vi "JSONtext Path Library Comparison.vi"() -> ()   [LabVIEW 2017]
uses:
  7f925563-714d-4489-9e01-5d8a939aa36c.vi
  <vilib>/addons/JSON API/JSON Value/Set from JSON string.vi
  Find Multiple Items.vi
  7f925563-714d-4489-9e01-5d8a939aa36c.vi/b1efde3c-89ab-4274-81c5-8c2e9ff736ec.vi
  String Subset.vi
  support/Strip Quotes and Unescape.vi
  Parse Full Path or Item Name.vi
  Find Item Locations by Path.vi
  support/Unescape JSON string.vi
  JSON text to Variant.vi
  <vilib>/addons/JSON API/Variant JSON/Get as Variant.vi
  <vilib>/addons/JSON API/JSON Value/JSON Value.lvclass
  <vilib>/addons/JSON API/Get Polymorphic/JSON GetSet.lvlib
  <vilib>/addons/JSON API/Variant JSON/Variant JSON.lvlib
  <vilib>/addons/_JKI.lib/Serialization/JSON/JKI JSON Serialization.lvlib
panel:
  in  "Library to use":T1(ring) caption="Enum 3"
  out "Array of Data":T2(array[cluster])
  out "JSON size (bytes)":i32 format="%.0p"
  out "Elements Returned":i32 format="%#.3p"
  out "Execution Time":dbl format="%#_3p"
  out "error out":errorcluster
  in  "Example JSON":string="[\n  {\n    \"_id\": \"59b53bcb02b0cb1b19bb98a8\",\n    \"index\": 0,\n    \"guid\": \"787c1912-662d-48b9-b395-2ad75d217224\",\n    \"isActive\": true,\n    \"balance\": \"$3,889.42\",\n    \"picture\": \"http://placehold.it/32x32\",\n    \"age\": 28,\n    \"eyeColor\": \"green\",\n    \"name\": \"Brady York\",\n    \"gender\": \"male\",\n    \"company\": \"ELEMANTRA\",\n    \"email\": \"bradyyork@elemantra.com\",\n    \"phone\": \"+1 (932) 487-2014\",\n    \"address\": \"349 Amber Street, Day, Rhode Island, 8815\",\n    \"about\": \"Culpa magna magna incididunt aliquip adipisicing incididunt. Culpa ex qui aliqua aliqua sint aliqua incididunt duis. Labore consectetur in pariatur qui anim reprehenderit duis.\\r\\n\",\n    \"registered\": \"2014-10-21T08:11:24 -01:00\",\n    \"latitude\": -14.331614,\n    \"longitude\": -65.032248,\n    \"tags\": [\n      \"sint\",\n      \"sint\",\n      \"magna\",\n      \"laboris\",\n      \"irure\",\n      \"aliquip\",\n      \"voluptate\"\n    ],\n    \"friends\": [\n      {\n        \"id\": 0,\n        \"name\": \"Magdalena Stanley\"\n      },\n      {\n        \"id\": 1,\n        \"name\": \"Gill Alvarez\"\n      },\n      {\n        \"id\": 2,\n        \"name\": \"Alston Pacheco\"\n      }\n    ],\n    \"greeting\": \"Hello, Brady York! You have 8 unread messages.\",\n    \"favoriteFruit\": \"banana\"\n  },\n  {\n    \"_id\": \"59b53bcb7e0f92dbc6bce359\",\n    \"index\": 1,\n    \"guid\": \"d1f7a7d2-daca-4b07-b037-18389dc096b8\",\n    \"isActive\": true,\n    \"balance\": \"$1,568.70\",\n    \"picture\": \"http://placehold.it/32x32\",\n    \"age\": 24,\n    \"eyeColor\": \"brown\",\n    \"name\": \"Eula Price\",\n    \"gender\": \"female\",\n    \"company\": \"LIMAGE\",\n    \"email\": \"eulaprice@limage.com\",\n    \"phone\": \"+1 (901) 569-3603\",\n    \"address\": \"883 Chester Avenue, Zeba, New Jersey, 8959\",\n    \"about\": \"Eiusmod aute do deserunt do sunt occaecat. Elit Lorem consequat consequat dolor. Ea ex exercitation nulla voluptate duis commodo fugiat tempor dolor exercitation nulla tempor. Incididunt ipsum sit minim eu excepteur commodo aliquip enim est incididunt dolore aute.\\r\\n\",\n    \"registered\": \"2017-06-22T12:52:36 -01:00\",\n    \"latitude\": -9.342636,\n    \"longitude\": -164.688312,\n    \"tags\": [\n      \"aliqua\",\n      \"anim\",\n      \"laboris\",\n      \"aliqua\",\n      \"dolore\",\n      \"reprehenderit\",\n      \"aute\"\n    ],\n    \"friends\": [\n      {\n        \"id\": 0,\n        \"name\": \"Lelia Gray\"\n      },\n      {\n        \"id\": 1,\n        \"name\": \"Gaines Owen\"\n      },\n      {\n        \"id\": 2,\n        \"name\": \"Lana Schneider\"\n      }\n    ],\n    \"greeting\": \"Hello, Eula Price! You have 6 unread messages.\",\n    \"favoriteFruit\": \"strawberry\"\n  },\n  {\n    \"_id\": \"59b53bcbc4753318b4f57283\",\n    \"index\": 2,\n    \"guid\": \"6fdbd945-01ed-452f-ad4a-aea4d254b9e8\",\n    \"isActive\": false,\n    \"balance\": \"$2,290.73\",\n    \"picture\": \"http://placehold.it/32x32\",\n    \"age\": 27,\n    \"eyeColor\": \"brown\",\n    \"name\": \"Kirk Battle\",\n    \"gender\": \"male\",\n    \"company\": \"TWIIST\",\n    \"email\": \"kirkbattle@twiist.com\",\n    \"phone\": \"+1 (880) 533-3536\",\n    \"address\": \"947 Evergreen Avenue, Eagletown, Kentucky, 5383\",\n    \"about\": \"Nostrud et pariatur labore sint. Est magna cillum enim consectetur veniam reprehenderit fugiat labore consectetur quis. Id ullamco minim amet ut cupidatat exercitation. Ullamco minim et do elit in voluptate voluptate duis. Voluptate duis ad sunt adipisicing minim officia velit dolore ea culpa eiusmod.\\r\\n\",\n    \"registered\": \"2015-06-20T10:39:15 -01:00\",\n    \"latitude\": 6.407172,\n    \"longitude\": -0.155464,\n    \"tags\": [\n      \"tempor\",\n      \"id\",\n      \"pariatur\",\n      \"dolore\",\n      \"nisi\",\n      \"sint\",\n      \"Lorem\"\n    ],\n    \"friends\": [\n      {\n        \"id\": 0,\n        \"name\": \"Dominguez Rasmussen\"\n      },\n      {\n        \"id\": 1,\n        \"name\": \"Augusta Gardner\"\n      },\n      {\n        \"id\": 2,\n        \"name\": \"Odom Nelson\"\n      }\n    ],\n    \"greeting\": \"Hello, Kirk Battle! You have 8 unread messages.\",\n    \"favoriteFruit\": \"banana\"\n  },\n  {\n    \"_id\": \"59b53bcb6051aabb2b97f0db\",\n    \"index\": 3,\n    \"guid\": \"2eb5b3b2-ee26-4324-ab7e-5653592530f9\",\n    \"isActive\": true,\n    \"balance\": \"$2,336.96\",\n    \"picture\": \"http://placehold.it/32x32\",\n    \"age\": 22,\n    \"eyeColor\": \"blue\",\n    \"name\": \"Bonnie Bell\",\n    \"gender\": \"female\",\n    \"company\": \"VIRVA\",\n    \"email\": \"bonniebell@virva.com\",\n    \"phone\": \"+1 (810) 554-2772\",\n    \"address\": \"559 Dakota Place, Kenmar, Arizona, 4025\",\n    \"about\": \"Anim in aliquip sunt fugiat laborum ea elit minim. Cillum nostrud ullamco ut minim nisi qui quis consequat deserunt in. Nostrud exercitation excepteur quis pariatur deserunt ea proident Lorem nostrud occaecat eu incididunt aute.\\r\\n\",\n    \"registered\": \"2016-10-31T11:45:40 -00:00\",\n    \"latitude\": -65.962147,\n    \"longitude\": 21.528794,\n    \"tags\": [\n      \"et\",\n      \"ex\",\n      \"in\",\n      \"ipsum\",\n      \"consectetur\",\n      \"eu\",\n      \"laborum\"\n    ],\n    \"friends\": [\n      {\n        \"id\": 0,\n        \"name\": \"Kirsten Keller\"\n      },\n      {\n        \"id\": 1,\n        \"name\": \"Martina Ferrell\"\n      },\n      {\n        \"id\": 2,\n        \"name\": \"Lambert Sutton\"\n      }\n    ],\n    \"greeting\": \"Hello, Bonnie Bell! You have 3 unread messages.\",\n    \"favoriteFruit\": \"banana\"\n  },\n  {\n    \"_id\": \"59b53bcb7231edd238041f2d\",\n    \"index\": 4,\n    \"guid\": \"f09317d0-8eee-46ff-9b91-58a5b0d46ece\",\n    \"isActive\": true,\n    \"balance\": \"$3,106.19\",\n    \"picture\": \"http://placehold.it/32x32\",\n    \"age\": 30,\n    \"eyeColor\": \"blue\",\n    \"name\": \"Krista Nichols\",\n    \"gender\": \"female\",\n    \"company\": \"ZORROMOP\",\n    \"email\": \"kristanichols@zorromop.com\",\n    \"phone\": \"+1 (807) 565-2677\",\n    \"address\": \"894 Norfolk Street, Clarktown, American Samoa, 9119\",\n    \"about\": \"Do est commodo esse in amet commodo non occaecat. Duis dolore ipsum fugiat amet aliqua ipsum est sunt est minim aliqua. Elit sit sit labore cupidatat do amet nulla.\\r\\n\",\n    \"registered\": \"2015-10-09T10:59:26 -01:00\",\n    \"latitude\": 54.865149,\n    \"longitude\": -44.341326,\n    \"tags\": [\n      \"sint\",\n      \"deserunt\",\n      \"elit\",\n      \"dolore\",\n      \"incididunt\",\n      \"sit\",\n      \"nostrud\"\n    ],\n    \"friends\": [\n      {\n        \"id\": 0,\n        \"name\": \"Sadie Carroll\"\n      },\n      {\n        \"id\": 1,\n        \"name\": \"Alice Oliver\"\n      },\n      {\n        \"id\": 2,\n        \"name\": \"Haynes Morris\"\n      }\n    ],\n    \"greeting\": \"Hello, Krista Nichols! You have 9 unread messages.\",\n    \"favoriteFruit\": \"banana\"\n  },\n  {\n    \"_id\": \"59b53bcbe9ba31e9db12c1da\",\n    \"index\": 5,\n    \"guid\": \"a3768281-1188-4880-8873-7d13400a9810\",\n    \"isActive\": true,\n    \"balance\": \"$2,102.60\",\n    \"picture\": \"http://placehold.it/32x32\",\n    \"age\": 37,\n    \"eyeColor\": \"blue\",\n    \"name\": \"Carver Gay\",\n    \"gender\": \"male\",\n    \"company\": \"COMTOURS\",\n    \"email\": \"carvergay@comtours.com\",\n    \"phone\": \"+1 (820) 410-2285\",\n    \"address\": \"253 Dare Court, Henrietta, Massachusetts, 2610\",\n    \"about\": \"Eiusmod magna Lorem anim incididunt do. Labore sunt id tempor veniam aliquip veniam non non reprehenderit reprehenderit consectetur amet. Do ad fugiat esse do ut proident dolore ad irure fugiat id fugiat aliqua consequat. Est quis consequat incididunt duis amet.\\r\\n\",\n    \"registered\": \"2016-03-09T10:06:33 -00:00\",\n    \"latitude\": -71.722611,\n    \"longitude\": 93.206354,\n    \"tags\": [\n      \"Lorem\",\n      \"laborum\",\n      \"cillum\",\n      \"culpa\",\n      \"quis\",\n      \"anim\",\n      \"Lorem\"\n    ],\n    \"friends\": [\n      {\n        \"id\": 0,\n        \"name\": \"Gibbs Silva\"\n      },\n      {\n        \"id\": 1,\n        \"name\": \"Vincent Herring\"\n      },\n      {\n        \"id\": 2,\n        \"name\": \"Bauer Edwards\"\n      }\n    ],\n    \"greeting\": \"Hello, Carver Gay! You have 2 unread messages.\",\n    \"favoriteFruit\": \"strawberry\"\n  },\n  {\n    \"_id\": \"59b53bcb7bbaae10a2aefeae\",\n    \"index\": 6,\n    \"guid\": \"bb9b5fd7-c1e4-4f49-b969-c4ee1fd49b81\",\n    \"isActive\": true,\n    \"balance\": \"$1,213.38\",\n    \"picture\": \"http://placehold.it/32x32\",\n    \"age\": 36,\n    \"eyeColor\": \"blue\",\n    \"name\": \"Jacobson Carlson\",\n    \"gender\": \"male\",\n    \"company\": \"GRONK\",\n    \"email\": \"jacobsoncarlson@gronk.com\",\n    \"phone\": \"+1 (892) 428-3382\",\n    \"address\": \"267 Empire Boulevard, Sena, Maine, 8522\",\n    \"about\": \"Eu nulla tempor reprehenderit laboris nostrud eiusmod. Elit aliquip veniam sit qui nisi ipsum enim cupidatat est qui adipisicing aute. Pariatur non et aliquip est. Consectetur cupidatat cupidatat consectetur nostrud dolor nostrud. Excepteur aliquip ut ipsum mollit culpa magna consequat adipisicing labore id est tempor amet. Incididunt ad tempor sit eiusmod officia duis amet.\\r\\n\",\n    \"registered\": \"2014-11-08T12:40:45 -00:00\",\n    \"latitude\": 74.024148,\n    \"longitude\": -149.038221,\n    \"tags\": [\n      \"deserunt\",\n      \"aliqua\",\n      \"do\",\n      \"excepteur\",\n      \"do\",\n      \"consequat\",\n      \"eiusmod\"\n    ],\n    \"friends\": [\n      {\n        \"id\": 0,\n        \"name\": \"Schmidt Boone\"\n      },\n      {\n        \"id\": 1,\n        \"name\": \"Chandler Guthrie\"\n      },\n      {\n        \"id\": 2,\n        \"name\": \"Mavis Beard\"\n      }\n    ],\n    \"greeting\": \"Hello, Jacobson Carlson! You have 4 unread messages.\",\n    \"favoriteFruit\": \"strawberry\"\n  },\n  {\n    \"_id\": \"59b53bcb03716bd89bef4059\",\n    \"index\": 7,\n    \"guid\": \"78ea5110-fabf-45ce-980c-5751b3eb6da0\",\n    \"isActive\": true,\n    \"balance\": \"$3,940.00\",\n    \"picture\": \"http://placehold.it/32x32\",\n    \"age\": 39,\n    \"eyeColor\": \"blue\",\n    \"name\": \"Holt Kirk\",\n    \"gender\": \"male\",\n    \"company\": \"GLEAMINK\",\n    \"email\": \"holtkirk@gleamink.com\",\n    \"phone\": \"+1 (978) 536-2129\",\n    \"address\": \"977 Maujer Street, Oberlin, Guam, 2555\",\n    \"about\": \"Ullamco dolore dolore cupidatat et occaecat nisi sunt et ea tempor qui est in. Elit amet ex ad ullamco tempor ea. Ipsum occaecat id culpa enim laborum id laborum aute dolor ullamco. Dolore est ut exercitation fugiat ad mollit consectetur. Labore esse non magna duis do. Est qui enim nisi exercitation ullamco ea cillum do ullamco.\\r\\n\",\n    \"registered\": \"2014-01-26T04:53:21 -00:00\",\n    \"latitude\": 80.154467,\n    \"longitude\": -139.457001,\n    \"tags\": [\n      \"in\",\n      \"proident\",\n      \"eu\",\n      \"esse\",\n      \"aute\",\n      \"ea\",\n      \"laborum\"\n    ],\n    \"friends\": [\n      {\n        \"id\": 0,\n        \"name\": \"Ayers Collins\"\n      },\n      {\n        \"id\": 1,\n        \"name\": \"Morgan Lynch\"\n      },\n      {\n        \"id\": 2,\n        \"name\": \"Millicent Rodriquez\"\n      }\n    ],\n    \"greeting\": \"Hello, Holt Kirk! You have 7 unread messages.\",\n    \"favoriteFruit\": \"strawberry\"\n  },\n  {\n    \"_id\": \"59b53bcbe46b05505f1d73c6\",\n    \"index\": 8,\n    \"guid\": \"5c0b76e2-83b6-48c8-a04b-d989644174a0\",\n    \"isActive\": false,\n    \"balance\": \"$2,251.01\",\n    \"picture\": \"http://placehold.it/32x32\",\n    \"age\": 34,\n    \"eyeColor\": \"blue\",\n    \"name\": \"Patrica Gates\",\n    \"gender\": \"female\",\n    \"company\": \"PAPRIKUT\",\n    \"email\": \"patricagates@paprikut.com\",\n    \"phone\": \"+1 (989) 486-2454\",\n    \"address\": \"284 Kane Street, Sheatown, Texas, 2404\",\n    \"about\": \"Veniam nostrud non veniam eiusmod mollit fugiat duis. Et Lorem elit ea eiusmod elit aute aute officia sit cillum. Consectetur cillum est duis sunt amet ex velit enim. Do consectetur sint deserunt deserunt minim esse dolore sit nisi ullamco cillum.\\r\\n\",\n    \"registered\": \"2014-10-22T11:45:11 -01:00\",\n    \"latitude\": -25.077939,\n    \"longitude\": -10.063782,\n    \"tags\": [\n      \"id\",\n      \"adipisicing\",\n      \"amet\",\n      \"nostrud\",\n      \"aliquip\",\n      \"ut\",\n      \"dolor\"\n    ],\n    \"friends\": [\n      {\n        \"id\": 0,\n        \"name\": \"Pollard Sawyer\"\n      },\n      {\n        \"id\": 1,\n        \"name\": \"Ortiz Perry\"\n      },\n      {\n        \"id\": 2,\n        \"name\": \"Britney Mullins\"\n      }\n    ],\n    \"greeting\": \"Hello, Patrica Gates! You have 5 unread messages.\",\n    \"favoriteFruit\": \"apple\"\n  },\n  {\n    \"_id\": \"59b53bcbcc629b542a162d0b\",\n    \"index\": 9,\n    \"guid\": \"4bc20eef-7f7d-48d6-8d1a-8c46d3ecaa0a\",\n    \"isActive\": true,\n    \"balance\": \"$1,093.57\",\n    \"picture\": \"http://placehold.it/32x32\",\n    \"age\": 24,\n    \"eyeColor\": \"green\",\n    \"name\": \"Latasha Holland\",\n    \"gender\": \"female\",\n    \"company\": \"CYTREX\",\n    \"email\": \"latashaholland@cytrex.com\",\n    \"phone\": \"+1 (898) 545-2211\",\n    \"address\": \"353 Elm Avenue, Steinhatchee, Colorado, 8565\",\n    \"about\": \"Laborum consectetur cupidatat fugiat laborum nulla enim exercitation. Esse amet quis eiusmod veniam est qui excepteur labore nisi ut aliqua incididunt occaecat ea. Tempor veniam laborum laboris in adipisicing veniam ex dolor nulla eiusmod voluptate qui ex irure.\\r\\n\",\n    \"registered\": \"2015-03-18T11:53:50 -00:00\",\n    \"latitude\": 18.52921,\n    \"longitude\": 82.506415,\n    \"tags\": [\n      \"ad\",\n      \"voluptate\",\n      \"aliquip\",\n      \"velit\",\n      \"non\",\n      \"qui\",\n      \"eiusmod\"\n    ],\n    \"friends\": [\n      {\n        \"id\": 0,\n        \"name\": \"Virginia Kramer\"\n      },\n      {\n        \"id\": 1,\n        \"name\": \"Alba Valencia\"\n      },\n      {\n        \"id\": 2,\n        \"name\": \"Alexandria Webster\"\n      }\n    ],\n    \"greeting\": \"Hello, Latasha Holland! You have 8 unread messages.\",\n    \"favoriteFruit\": \"strawberry\"\n  },\n  {\n    \"_id\": \"59b53bcb597148582fb2963b\",\n    \"index\": 10,\n    \"guid\": \"11d9df14-d3e9-4f7b-bb2c-951e6152d5dd\",\n    \"isActive\": false,\n    \"balance\": \"$1,684.85\",\n    \"picture\": \"http://placehold.it/32x32\",\n    \"age\": 39,\n    \"eyeColor\": \"green\",\n    \"name\": \"Dena Webb\",\n    \"gender\": \"female\",\n    \"company\": \"OPTIQUE\",\n    \"email\": \"denawebb@optique.com\",\n    \"phone\": \"+1 (814) 500-3050\",\n    \"address\": \"542 Bouck Court, Dixonville, Utah, 4706\",\n    \"about\": \"Ad esse duis id excepteur cillum est proident do ullamco. Nulla sunt non fugiat nulla velit ex qui pariatur reprehenderit proident ullamco est. Nulla culpa ullamco minim dolor elit cupidatat veniam sit incididunt mollit elit consequat sit velit. Est quis occaecat ut do id aute. Minim laboris minim ut duis labore do laboris officia. In occaecat et officia reprehenderit amet laborum dolor ullamco. Labore dolor ipsum anim qui cupidatat non magna sunt id mollit aliquip commodo id.\\r\\n\",\n    \"registered\": \"2014-06-03T06:37:29 -01:00\",\n    \"latitude\": 51.581221,\n    \"longitude\": 165.78903,\n    \"tags\": [\n      \"occaecat\",\n      \"magna\",\n      \"consequat\",\n      \"do\",\n      \"ullamco\",\n      \"eiusmod\",\n      \"consectetur\"\n    ],\n    \"friends\": [\n      {\n        \"id\": 0,\n        \"name\": \"Sharron Cleveland\"\n      },\n      {\n        \"id\": 1,\n        \"name\": \"Rosanna Chase\"\n      },\n      {\n        \"id\": 2,\n        \"name\": \"Amanda Lara\"\n      }\n    ],\n    \"greeting\": \"Hello, Dena Webb! You have 2 unread messages.\",\n    \"favoriteFruit\": \"banana\"\n  },\n  {\n    \"_id\": \"59b53bcbd26ca7bf6f477c07\",\n    \"index\": 11,\n    \"guid\": \"b2758586-d7dc-4aee-bf7e-ec0e02885def\",\n    \"isActive\": true,\n    \"balance\": \"$3,763.33\",\n    \"picture\": \"http://placehold.it/32x32\",\n    \"age\": 32,\n    \"eyeColor\": \"blue\",\n    \"name\": \"Howe Conner\",\n    \"gender\": \"male\",\n    \"company\": \"ATOMICA\",\n    \"email\": \"howeconner@atomica.com\",\n    \"phone\": \"+1 (945) 508-3886\",\n    \"address\": \"335 Cumberland Street, Glenville, Montana, 8652\",\n    \"about\": \"Aute culpa ipsum id anim veniam. Duis laboris ad ullamco proident veniam minim. Cillum velit aliqua amet est. Eu fugiat occaecat sunt pariatur ex.\\r\\n\",\n    \"registered\": \"2015-03-15T08:28:33 -00:00\",\n    \"latitude\": -28.365675,\n    \"longitude\": -65.023882,\n    \"tags\": [\n      \"adipisicing\",\n      \"proident\",\n      \"qui\",\n      \"aute\",\n      \"excepteur\",\n      \"Lorem\",\n      \"nostrud\"\n    ],\n    \"friends\": [\n      {\n        \"id\": 0,\n        \"name\": \"Lucinda Mcclain\"\n      },\n      {\n        \"id\": 1,\n        \"name\": \"Butler Guerrero\"\n      },\n      {\n        \"id\": 2,\n        \"name\": \"Lakeisha Spears\"\n      }\n    ],\n    \"greeting\": \"Hello, Howe Conner! You have 2 unread messages.\",\n    \"favoriteFruit\": \"banana\"\n  },\n  {\n    \"_id\": \"59b53bcbb5418a3e477d54c9\",\n    \"index\": 12,\n    \"guid\": \"e66672d5-084b-400c-9106-13a25f1ffc78\",\n    \"isActive\": true,\n    \"balance\": \"$1,591.82\",\n    \"picture\": \"http://placehold.it/32x32\",\n    \"age\": 27,\n    \"eyeColor\": \"brown\",\n    \"name\": \"Anne Nielsen\",\n    \"gender\": \"female\",\n    \"company\": \"VIOCULAR\",\n    \"email\": \"annenielsen@viocular.com\",\n    \"phone\": \"+1 (970) 495-2904\",\n    \"address\": \"855 Caton Place, Como, Maryland, 9034\",\n    \"about\": \"Tempor anim quis ut aliqua nulla officia occaecat do sit anim ad. Occaecat dolor dolor ad incididunt quis veniam. Labore velit do elit duis laborum consequat Lorem aliquip. Est aliqua occaecat reprehenderit eu laborum ea et sint ea anim consectetur. Anim dolore officia nostrud aute ad adipisicing laboris et occaecat mollit. Tempor dolor ex eu proident elit in.\\r\\n\",\n    \"registered\": \"2017-05-08T12:38:29 -01:00\",\n    \"latitude\": -47.604574,\n    \"longitude\": 7.244034,\n    \"tags\": [\n      \"amet\",\n      \"consequat\",\n      \"magna\",\n      \"excepteur\",\n      \"laboris\",\n      \"tempor\",\n      \"minim\"\n    ],\n    \"friends\": [\n      {\n        \"id\": 0,\n        \"name\": \"Nita Ellison\"\n      },\n      {\n        \"id\": 1,\n        \"name\": \"Kelley England\"\n      },\n      {\n        \"id\": 2,\n        \"name\": \"Blanca Duke\"\n      }\n    ],\n    \"greeting\": \"Hello, Anne Nielsen! You have 5 unread messages.\",\n    \"favoriteFruit\": \"strawberry\"\n  },\n  {\n    \"_id\": \"59b53bcb4ce81ca8bb52f70c\",\n    \"index\": 13,\n    \"guid\": \"2ab4ca63-31a2-4867-9969-bff002881044\",\n    \"isActive\": true,\n    \"balance\": \"$2,822.43\",\n    \"picture\": \"http://placehold.it/32x32\",\n    \"age\": 32,\n    \"eyeColor\": \"green\",\n    \"name\": \"Carroll Kline\",\n    \"gender\": \"male\",\n    \"company\": \"FORTEAN\",\n    \"email\": \"carrollkline@fortean.com\",\n    \"phone\": \"+1 (980) 498-3294\",\n    \"address\": \"111 Goodwin Place, Jardine, Connecticut, 370\",\n    \"about\": \"Lorem aute laborum id labore non nisi veniam ad fugiat labore. Minim fugiat reprehenderit exercitation aliqua ipsum velit Lorem labore ad aliquip nisi cillum eiusmod. Quis aliquip reprehenderit commodo pariatur aliquip eu aute quis dolore occaecat. Nisi id esse ea pariatur voluptate et elit ut ut mollit ea.\\r\\n\",\n    \"registered\": \"2014-12-13T11:18:37 -00:00\",\n    \"latitude\": 44.611706,\n    \"longitude\": -75.982853,\n    \"tags\": [\n      \"non\",\n      \"mollit\",\n      \"pariatur\",\n      \"ad\",\n      \"aliqua\",\n      \"do\",\n      \"laboris\"\n    ],\n    \"friends\": [\n      {\n        \"id\": 0,\n        \"name\": \"Cannon Navarro\"\n      },\n      {\n        \"id\": 1,\n        \"name\": \"Terri Byers\"\n      },\n      {\n        \"id\": 2,\n        \"name\": \"Janell Robinson\"\n      }\n    ],\n    \"greeting\": \"Hello, Carroll Kline! You have 4 unread messages.\",\n    \"favoriteFruit\": \"banana\"\n  },\n  {\n    \"_id\": \"59b53bcb034cefc38e5f718d\",\n    \"index\": 14,\n    \"guid\": \"1b75941b-966f-4520-bda0-746f5f72a03e\",\n    \"isActive\": false,\n    \"balance\": \"$2,799.30\",\n    \"picture\": \"http://placehold.it/32x32\",\n    \"age\": 32,\n    \"eyeColor\": \"brown\",\n    \"name\": \"Forbes Tran\",\n    \"gender\": \"male\",\n    \"company\": \"LYRIA\",\n    \"email\": \"forbestran@lyria.com\",\n    \"phone\": \"+1 (932) 582-3482\",\n    \"address\": \"689 Cook Street, Cleary, Iowa, 2553\",\n    \"about\": \"Occaecat tempor sint nisi amet ex veniam culpa adipisicing ad. Incididunt duis elit amet deserunt eiusmod officia occaecat eiusmod qui incididunt. Eiusmod laboris esse sit incididunt enim eu excepteur est mollit anim ad quis. Mollit nulla culpa veniam incididunt ipsum sit officia sunt aliqua reprehenderit dolor dolore. Culpa excepteur consequat magna elit id ullamco deserunt est in et irure.\\r\\n\",\n    \"registered\": \"2015-05-22T09:52:23 -01:00\",\n    \"latitude\": 9.60954,\n    \"longitude\": -42.310375,\n    \"tags\": [\n      \"mollit\",\n      \"proident\",\n      \"veniam\",\n      \"irure\",\n      \"esse\",\n      \"Lorem\",\n      \"dolore\"\n    ],\n    \"friends\": [\n      {\n        \"id\": 0,\n        \"name\": \"Leila Sims\"\n      },\n      {\n        \"id\": 1,\n        \"name\": \"Desiree Savage\"\n      },\n      {\n        \"id\": 2,\n        \"name\": \"Johnston Hensley\"\n      }\n    ],\n    \"greeting\": \"Hello, Forbes Tran! You have 3 unread messages.\",\n    \"favoriteFruit\": \"banana\"\n  },\n  {\n    \"_id\": \"59b53bcb9a6e9676f507278e\",\n    \"index\": 15,\n    \"guid\": \"3bed5db5-ef23-4804-a3e0-08b3c940d53f\",\n    \"isActive\": true,\n    \"balance\": \"$1,219.22\",\n    \"picture\": \"http://placehold.it/32x32\",\n    \"age\": 39,\n    \"eyeColor\": \"brown\",\n    \"name\": \"Carlson Klein\",\n    \"gender\": \"male\",\n    \"company\": \"AQUACINE\",\n    \"email\": \"carlsonklein@aquacine.com\",\n    \"phone\": \"+1 (978) 572-2330\",\n    \"address\": \"863 Woods Place, Movico, Wyoming, 810\",\n    \"about\": \"Do excepteur nostrud est nisi minim incididunt cillum. Et veniam do in proident deserunt minim sit. Sunt pariatur ipsum tempor elit duis sint sit non non qui laborum duis esse. Sint eiusmod irure pariatur occaecat reprehenderit anim.\\r\\n\",\n    \"registered\": \"2014-05-03T11:19:28 -01:00\",\n    \"latitude\": -56.803333,\n    \"longitude\": -128.863204,\n    \"tags\": [\n      \"tempor\",\n      \"velit\",\n      \"voluptate\",\n      \"et\",\n      \"laboris\",\n      \"consequat\",\n      \"cillum\"\n    ],\n    \"friends\": [\n      {\n        \"id\": 0,\n        \"name\": \"Liliana Sellers\"\n      },\n      {\n        \"id\": 1,\n        \"name\": \"Garcia Larsen\"\n      },\n      {\n        \"id\": 2,\n        \"name\": \"Long Fitzpatrick\"\n      }\n    ],\n    \"greeting\": \"Hello, Carlson Klein! You have 4 unread messages.\",\n    \"favoriteFruit\": \"strawberry\"\n  },\n  {\n    \"_id\": \"59b53bcbac141192de4ff36f\",\n    \"index\": 16,\n    \"guid\": \"5c96733c-76df-40fa-b2b3-d65d58dc0720\",\n    \"isActive\": true,\n    \"balance\": \"$2,144.12\",\n    \"picture\": \"http://placehold.it/32x32\",\n    \"age\": 38,\n    \"eyeColor\": \"blue\",\n    \"name\": \"Maryann Adams\",\n    \"gender\": \"female\",\n    \"company\": \"GEEKY\",\n    \"email\": \"maryannadams@geeky.com\",\n    \"phone\": \"+1 (814) 507-3036\",\n    \"address\": \"701 Albemarle Terrace, Datil, Marshall Islands, 1322\",\n    \"about\": \"Ipsum velit nostrud minim aute velit ut esse occaecat ad voluptate qui ad. Mollit pariatur ullamco Lorem quis elit incididunt anim ullamco officia laborum. Ad incididunt ut ipsum elit elit culpa magna. Nulla quis ex est elit commodo deserunt culpa culpa sint occaecat do. Consectetur irure officia culpa id ex. Et est id minim proident Lorem ea esse aute et qui. Quis enim duis minim sint elit nostrud.\\r\\n\",\n    \"registered\": \"2016-11-20T04:37:14 -00:00\",\n    \"latitude\": -61.054651,\n    \"longitude\": -110.864468,\n    \"tags\": [\n      \"excepteur\",\n      \"minim\",\n      \"amet\",\n      \"magna\",\n      \"fugiat\",\n      \"excepteur\",\n      \"consectetur\"\n    ],\n    \"friends\": [\n      {\n        \"id\": 0,\n        \"name\": \"Megan Petersen\"\n      },\n      {\n        \"id\": 1,\n        \"name\": \"Arline Solis\"\n      },\n      {\n        \"id\": 2,\n        \"name\": \"Carpenter Bishop\"\n      }\n    ],\n    \"greeting\": \"Hello, Maryann Adams! You have 4 unread messages.\",\n    \"favoriteFruit\": \"apple\"\n  },\n  {\n    \"_id\": \"59b53bcbd4794b54dacb02ff\",\n    \"index\": 17,\n    \"guid\": \"9b12691d-534a-49ef-9453-e6db5e086fa3\",\n    \"isActive\": true,\n    \"balance\": \"$1,444.83\",\n    \"picture\": \"http://placehold.it/32x32\",\n    \"age\": 23,\n    \"eyeColor\": \"brown\",\n    \"name\": \"Zelma Hooper\",\n    \"gender\": \"female\",\n    \"company\": \"ENDICIL\",\n    \"email\": \"zelmahooper@endicil.com\",\n    \"phone\": \"+1 (953) 529-2225\",\n    \"address\": \"327 Cherry Street, Sylvanite, Nevada, 1609\",\n    \"about\": \"Aliquip consectetur dolor magna irure voluptate ea. Labore id aute incididunt eiusmod ad cillum est exercitation excepteur officia cupidatat aute. Sit et magna duis duis excepteur ad est sit sint adipisicing commodo. Sint est quis amet ullamco cupidatat nisi enim sint do et.\\r\\n\",\n    \"registered\": \"2015-10-10T05:49:22 -01:00\",\n    \"latitude\": -69.361083,\n    \"longitude\": -9.671064,\n    \"tags\": [\n      \"veniam\",\n      \"officia\",\n      \"dolore\",\n      \"dolore\",\n      \"occaecat\",\n      \"excepteur\",\n      \"dolore\"\n    ],\n    \"friends\": [\n      {\n        \"id\": 0,\n        \"name\": \"Hughes Mcgowan\"\n      },\n      {\n        \"id\": 1,\n        \"name\": \"Corrine Velazquez\"\n      },\n      {\n        \"id\": 2,\n        \"name\": \"Wade Kirkland\"\n      }\n    ],\n    \"greeting\": \"Hello, Zelma Hooper! You have 6 unread messages.\",\n    \"favoriteFruit\": \"strawberry\"\n  },\n  {\n    \"_id\": \"59b53bcb68e219d872f06a49\",\n    \"index\": 18,\n    \"guid\": \"861c801f-0f15-4390-8104-311e6d6f83d8\",\n    \"isActive\": true,\n    \"balance\": \"$2,222.35\",\n    \"picture\": \"http://placehold.it/32x32\",\n    \"age\": 34,\n    \"eyeColor\": \"green\",\n    \"name\": \"Gwen Cook\",\n    \"gender\": \"female\",\n    \"company\": \"BESTO\",\n    \"email\": \"gwencook@besto.com\",\n    \"phone\": \"+1 (999) 515-3826\",\n    \"address\": \"151 Wythe Place, Hessville, North Carolina, 3410\",\n    \"about\": \"Fugiat aliqua nulla ea et do tempor ex sit mollit. Aliquip id dolor incididunt eu anim. Qui ex Lorem ut tempor veniam sit nostrud. Sint elit adipisicing laboris exercitation enim sint. Ipsum in anim quis magna. Ullamco deserunt voluptate reprehenderit tempor ea proident ea. Ea ad deserunt esse anim quis.\\r\\n\",\n    \"registered\": \"2016-01-02T10:58:42 -00:00\",\n    \"latitude\": 62.88102,\n    \"longitude\": -110.611076,\n    \"tags\": [\n      \"veniam\",\n      \"consectetur\",\n      \"consequat\",\n      \"fugiat\",\n      \"aliqua\",\n      \"incididunt\",\n      \"deserunt\"\n    ],\n    \"friends\": [\n      {\n        \"id\": 0,\n        \"name\": \"Powell Burris\"\n      },\n      {\n        \"id\": 1,\n        \"name\": \"Nina Burt\"\n      },\n      {\n        \"id\": 2,\n        \"name\": \"Brandi Barber\"\n      }\n    ],\n    \"greeting\": \"Hello, Gwen Cook! You have 4 unread messages.\",\n    \"favoriteFruit\": \"apple\"\n  },\n  {\n    \"_id\": \"59b53bcb7b31d5c7dd72738c\",\n    \"index\": 19,\n    \"guid\": \"a44d6ef3-72ce-47e3-be35-e26aef54e05c\",\n    \"isActive\": true,\n    \"balance\": \"$2,772.61\",\n    \"picture\": \"http://placehold.it/32x32\",\n    \"age\": 27,\n    \"eyeColor\": \"brown\",\n    \"name\": \"Ray Sheppard\",\n    \"gender\": \"male\",\n    \"company\": \"STEELFAB\",\n    \"email\": \"raysheppard@steelfab.com\",\n    \"phone\": \"+1 (833) 576-3166\",\n    \"address\": \"421 Noel Avenue, Fruitdale, New Mexico, 1023\",\n    \"about\": \"Nisi tempor ea nostrud reprehenderit labore Lorem proident adipisicing aliqua anim ad. Lorem id mollit nisi et minim nostrud proident commodo et dolore ex. Lorem anim eu eu sint exercitation sint.\\r\\n\",\n    \"registered\": \"2016-10-14T02:28:34 -01:00\",\n    \"latitude\": -21.473911,\n    \"longitude\": -178.75414,\n    \"tags\": [\n      \"deserunt\",\n      \"sint\",\n      \"culpa\",\n      \"mollit\",\n      \"minim\",\n      \"aute\",\n      \"dolor\"\n    ],\n    \"friends\": [\n      {\n        \"id\": 0,\n        \"name\": \"Joan Donaldson\"\n      },\n      {\n        \"id\": 1,\n        \"name\": \"Lilly Hansen\"\n      },\n      {\n        \"id\": 2,\n        \"name\": \"Francis Foster\"\n      }\n    ],\n    \"greeting\": \"Hello, Ray Sheppard! You have 1 unread messages.\",\n    \"favoriteFruit\": \"banana\"\n  },\n  {\n    \"_id\": \"59b53bcbfc475205683d24fb\",\n    \"index\": 20,\n    \"guid\": \"70656bad-68de-4581-9553-567f23d70256\",\n    \"isActive\": false,\n    \"balance\": \"$1,071.41\",\n    \"picture\": \"http://placehold.it/32x32\",\n    \"age\": 23,\n    \"eyeColor\": \"green\",\n    \"name\": \"Kerr Bowman\",\n    \"gender\": \"male\",\n    \"company\": \"SUPPORTAL\",\n    \"email\": \"kerrbowman@supportal.com\",\n    \"phone\": \"+1 (915) 525-3701\",\n    \"address\": \"387 Gallatin Place, Williston, Michigan, 658\",\n    \"about\": \"Sint nostrud qui deserunt sit tempor esse do sunt amet exercitation anim nulla. Eiusmod ex tempor in officia consequat dolor exercitation irure incididunt nulla nulla do. Mollit magna do et ea cupidatat elit ipsum adipisicing voluptate cupidatat eiusmod non.\\r\\n\",\n    \"registered\": \"2015-07-19T05:10:09 -01:00\",\n    \"latitude\": -61.588655,\n    \"longitude\": -69.987029,\n    \"tags\": [\n      \"laborum\",\n      \"laborum\",\n      \"consequat\",\n      \"ut\",\n      \"magna\",\n      \"voluptate\",\n      \"esse\"\n    ],\n    \"friends\": [\n      {\n        \"id\": 0,\n        \"name\": \"Beryl Wolfe\"\n      },\n      {\n        \"id\": 1,\n        \"name\": \"Viola Hamilton\"\n      },\n      {\n        \"id\": 2,\n        \"name\": \"Jannie Whitehead\"\n      }\n    ],\n    \"greeting\": \"Hello, Kerr Bowman! You have 2 unread messages.\",\n    \"favoriteFruit\": \"banana\"\n  },\n  {\n    \"_id\": \"59b53bcb8d287deabf6d0b79\",\n    \"index\": 21,\n    \"guid\": \"7c1a5e48-bb0e-4c13-81d4-88d15f5cbdd2\",\n    \"isActive\": false,\n    \"balance\": \"$3,025.85\",\n    \"picture\": \"http://placehold.it/32x32\",\n    \"age\": 31,\n    \"eyeColor\": \"green\",\n    \"name\": \"Aline Fleming\",\n    \"gender\": \"female\",\n    \"company\": \"COMCUR\",\n    \"email\": \"alinefleming@comcur.com\",\n    \"phone\": \"+1 (973) 454-2935\",\n    \"address\": \"736 Harbor Court, Allison, Oregon, 7524\",\n    \"about\": \"Do dolore deserunt dolor anim ex cillum ea amet ipsum in irure. Labore nisi culpa deserunt ipsum quis exercitation fugiat esse velit dolor reprehenderit. Ea id non quis ipsum officia. Enim veniam minim excepteur do dolore commodo nulla culpa irure.\\r\\n\",\n    \"registered\": \"2015-03-20T09:17:16 -00:00\",\n    \"latitude\": -85.661732,\n    \"longitude\": -109.540686,\n    \"tags\": [\n      \"laborum\",\n      \"aute\",\n      \"do\",\n      \"magna\",\n      \"do\",\n      \"Lorem\",\n      \"officia\"\n    ],\n    \"friends\": [\n      {\n        \"id\": 0,\n        \"name\": \"Corinne Rush\"\n      },\n      {\n        \"id\": 1,\n        \"name\": \"Pearlie Fuentes\"\n      },\n      {\n        \"id\": 2,\n        \"name\": \"Shelton Mendoza\"\n      }\n    ],\n    \"greeting\": \"Hello, Aline Fleming! You have 9 unread messages.\",\n    \"favoriteFruit\": \"banana\"\n  },\n  {\n    \"_id\": \"59b53bcb21bc1b9e689f86cd\",\n    \"index\": 22,\n    \"guid\": \"89e79c28-d1d3-4cf0-a7db-e52663288896\",\n    \"isActive\": false,\n    \"balance\": \"$1,913.46\",\n    \"picture\": \"http://placehold.it/32x32\",\n    \"age\": 20,\n    \"eyeColor\": \"green\",\n    \"name\": \"Stacey Hickman\",\n    \"gender\": \"female\",\n    \"company\": \"OLYMPIX\",\n    \"email\": \"staceyhickman@olympix.com\",\n    \"phone\": \"+1 (885) 484-3824\",\n    \"address\": \"738 Oxford Walk, Bagtown, Florida, 6859\",\n    \"about\": \"Occaecat in in do commodo esse aute. Consectetur voluptate amet dolore ad amet reprehenderit. Ut ullamco velit labore exercitation commodo adipisicing ea ea. Cupidatat do pariatur excepteur commodo tempor aute sint exercitation.\\r\\n\",\n    \"registered\": \"2017-06-13T05:36:22 -01:00\",\n    \"latitude\": 48.262654,\n    \"longitude\": -98.857032,\n    \"tags\": [\n      \"culpa\",\n      \"excepteur\",\n      \"irure\",\n      \"officia\",\n      \"minim\",\n      \"mollit\",\n      \"officia\"\n    ],\n    \"friends\": [\n      {\n        \"id\": 0,\n        \"name\": \"Natasha Anderson\"\n      },\n      {\n        \"id\": 1,\n        \"name\": \"Blackwell Blanchard\"\n      },\n      {\n        \"id\": 2,\n        \"name\": \"Iva Riggs\"\n      }\n    ],\n    \"greeting\": \"Hello, Stacey Hickman! You have 1 unread messages.\",\n    \"favoriteFruit\": \"banana\"\n  },\n  {\n    \"_id\": \"59b53bcbf9cf2b4cfa69d511\",\n    \"index\": 23,\n    \"guid\": \"54e3fdd1-4f8d-42dc-9828-ba8270d810c4\",\n    \"isActive\": true,\n    \"balance\": \"$1,863.08\",\n    \"picture\": \"http://placehold.it/32x32\",\n    \"age\": 30,\n    \"eyeColor\": \"brown\",\n    \"name\": \"Dora Larson\",\n    \"gender\": \"female\",\n    \"company\": \"XTH\",\n    \"email\": \"doralarson@xth.com\",\n    \"phone\": \"+1 (817) 432-2284\",\n    \"address\": \"433 Love Lane, Cliff, Minnesota, 8201\",\n    \"about\": \"Ad id pariatur nulla Lorem consequat. In veniam dolore do nisi incididunt. Mollit occaecat quis irure ut consectetur in duis culpa adipisicing in sunt consequat adipisicing.\\r\\n\",\n    \"registered\": \"2015-03-08T09:12:31 -00:00\",\n    \"latitude\": 42.824631,\n    \"longitude\": -141.172328,\n    \"tags\": [\n      \"laborum\",\n      \"ut\",\n      \"fugiat\",\n      \"veniam\",\n      \"cupidatat\",\n      \"sit\",\n      \"et\"\n    ],\n    \"friends\": [\n      {\n        \"id\": 0,\n        \"name\": \"Coffey Munoz\"\n      },\n      {\n        \"id\": 1,\n        \"name\": \"Hope Case\"\n      },\n      {\n        \"id\": 2,\n        \"name\": \"Marquez Hutchinson\"\n      }\n    ],\n    \"greeting\": \"Hello, Dora Larson! You have 9 unread messages.\",\n    \"favoriteFruit\": \"banana\"\n  },\n  {\n    \"_id\": \"59b53bcb7452ac2216503911\",\n    \"index\": 24,\n    \"guid\": \"305c5641-1f82-4362-953f-80e8de19eacf\",\n    \"isActive\": false,\n    \"balance\": \"$3,504.96\",\n    \"picture\": \"http://placehold.it/32x32\",\n    \"age\": 32,\n    \"eyeColor\": \"brown\",\n    \"name\": \"Estes Wilkins\",\n    \"gender\": \"male\",\n    \"company\": \"GUSHKOOL\",\n    \"email\": \"esteswilkins@gushkool.com\",\n    \"phone\": \"+1 (957) 533-3834\",\n    \"address\": \"168 Krier Place, Cartwright, Hawaii, 187\",\n    \"about\": \"Elit consectetur minim quis esse proident cillum cupidatat. Occaecat aute velit do Lorem ullamco esse. Duis eu sint dolore ut mollit cupidatat consectetur minim et in nostrud. Adipisicing labore incididunt id eiusmod elit reprehenderit. Ea ullamco aliquip cillum proident mollit aliqua nostrud. Dolore aliqua mollit deserunt aliqua deserunt veniam.\\r\\n\",\n    \"registered\": \"2015-06-16T05:18:07 -01:00\",\n    \"latitude\": -48.357251,\n    \"longitude\": 179.978918,\n    \"tags\": [\n      \"id\",\n      \"ullamco\",\n      \"exercitation\",\n      \"adipisicing\",\n      \"esse\",\n      \"eu\",\n      \"veniam\"\n    ],\n    \"friends\": [\n      {\n        \"id\": 0,\n        \"name\": \"Small Gibson\"\n      },\n      {\n        \"id\": 1,\n        \"name\": \"Gonzalez Potts\"\n      },\n      {\n        \"id\": 2,\n        \"name\": \"Alvarez Mcguire\"\n      }\n    ],\n    \"greeting\": \"Hello, Estes Wilkins! You have 10 unread messages.\",\n    \"favoriteFruit\": \"strawberry\"\n  },\n  {\n    \"_id\": \"59b53bcb9a5eee5c2af3c441\",\n    \"index\": 25,\n    \"guid\": \"c524b090-0f2c-4b34-b60b-c57e786f3800\",\n    \"isActive\": false,\n    \"balance\": \"$3,668.62\",\n    \"picture\": \"http://placehold.it/32x32\",\n    \"age\": 25,\n    \"eyeColor\": \"blue\",\n    \"name\": \"Betsy Leblanc\",\n    \"gender\": \"female\",\n    \"company\": \"FANFARE\",\n    \"email\": \"betsyleblanc@fanfare.com\",\n    \"phone\": \"+1 (879) 416-2965\",\n    \"address\": \"393 Prospect Avenue, Thermal, Pennsylvania, 1021\",\n    \"about\": \"Voluptate do duis amet ut dolor eiusmod nisi deserunt fugiat consequat. Proident officia reprehenderit voluptate nisi qui anim incididunt reprehenderit id. Culpa dolor adipisicing eu duis aute occaecat irure adipisicing aliqua. Duis sunt eiusmod occaecat ipsum do anim elit consectetur magna irure elit. Laboris nisi ea in elit sit pariatur est nostrud amet.\\r\\n\",\n    \"registered\": \"2014-08-22T09:02:28 -01:00\",\n    \"latitude\": -20.158386,\n    \"longitude\": 36.762045,\n    \"tags\": [\n      \"veniam\",\n      \"id\",\n      \"deserunt\",\n      \"aliquip\",\n      \"labore\",\n      \"consectetur\",\n      \"voluptate\"\n    ],\n    \"friends\": [\n      {\n        \"id\": 0,\n        \"name\": \"Esperanza Meadows\"\n      },\n      {\n        \"id\": 1,\n        \"name\": \"Jacquelyn Booker\"\n      },\n      {\n        \"id\": 2,\n        \"name\": \"Justine Higgins\"\n      }\n    ],\n    \"greeting\": \"Hello, Betsy Leblanc! You have 4 unread messages.\",\n    \"favoriteFruit\": \"apple\"\n  },\n  {\n    \"_id\": \"59b53bcb8b6a556b334bc9b5\",\n    \"index\": 26,\n    \"guid\": \"c4d258cd-4b15-4f62-a48a-45ae318736cc\",\n    \"isActive\": false,\n    \"balance\": \"$1,381.58\",\n    \"picture\": \"http://placehold.it/32x32\",\n    \"age\": 27,\n    \"eyeColor\": \"brown\",\n    \"name\": \"Gabriela Knowles\",\n    \"gender\": \"female\",\n    \"company\": \"GOLISTIC\",\n    \"email\": \"gabrielaknowles@golistic.com\",\n    \"phone\": \"+1 (984) 554-3557\",\n    \"address\": \"108 Gerry Street, Ryderwood, Virginia, 954\",\n    \"about\": \"Nostrud adipisicing duis cupidatat mollit incididunt velit commodo ea elit commodo. Magna duis consectetur labore ullamco ullamco. Proident enim ad enim ex aliquip dolor duis non ipsum nulla do enim nostrud cillum. Anim cillum labore mollit proident cillum esse culpa consequat id exercitation dolor officia sunt. Anim ipsum deserunt enim proident cupidatat tempor.\\r\\n\",\n    \"registered\": \"2017-03-10T12:46:33 -00:00\",\n    \"latitude\": -72.605964,\n    \"longitude\": -124.787196,\n    \"tags\": [\n      \"in\",\n      \"dolore\",\n      \"elit\",\n      \"magna\",\n      \"in\",\n      \"occaecat\",\n      \"ipsum\"\n    ],\n    \"friends\": [\n      {\n        \"id\": 0,\n        \"name\": \"Shannon Nolan\"\n      },\n      {\n        \"id\": 1,\n        \"name\": \"Leann Herrera\"\n      },\n      {\n        \"id\": 2,\n        \"name\": \"Sheppard Frost\"\n      }\n    ],\n    \"greeting\": \"Hello, Gabriela Knowles! You have 6 unread messages.\",\n    \"favoriteFruit\": \"banana\"\n  },\n  {\n    \"_id\": \"59b53bcb93de39cd0c0af940\",\n    \"index\": 27,\n    \"guid\": \"0f0552d9-e7b3-4c57-b6c7-1e2135a1104f\",\n    \"isActive\": false,\n    \"balance\": \"$3,811.17\",\n    \"picture\": \"http://placehold.it/32x32\",\n    \"age\": 38,\n    \"eyeColor\": \"brown\",\n    \"name\": \"Merrill Ray\",\n    \"gender\": \"male\",\n    \"company\": \"SOLAREN\",\n    \"email\": \"merrillray@solaren.com\",\n    \"phone\": \"+1 (835) 524-2354\",\n    \"address\": \"227 Seacoast Terrace, Waterford, Kansas, 9740\",\n    \"about\": \"Magna eiusmod duis pariatur eiusmod minim et officia sit amet ipsum ut sint magna Lorem. Nisi velit sit adipisicing deserunt voluptate consectetur dolor officia voluptate elit adipisicing sit. Sint dolore occaecat ea duis voluptate duis sint ullamco in quis pariatur irure. Ipsum magna voluptate nulla deserunt eiusmod consectetur ut tempor qui pariatur quis duis. Lorem dolore qui adipisicing pariatur mollit cillum sunt nisi id deserunt tempor nisi amet. Sit cillum nisi dolore magna exercitation anim ad id consequat duis.\\r\\n\",\n    \"registered\": \"2016-06-15T02:30:18 -01:00\",\n    \"latitude\": 82.245484,\n    \"longitude\": -22.28782,\n    \"tags\": [\n      \"quis\",\n      \"pariatur\",\n      \"nisi\",\n      \"culpa\",\n      \"ut\",\n      \"minim\",\n      \"amet\"\n    ],\n    \"friends\": [\n      {\n        \"id\": 0,\n        \"name\": \"Fleming Rosario\"\n      },\n      {\n        \"id\": 1,\n        \"name\": \"Mcconnell Griffin\"\n      },\n      {\n        \"id\": 2,\n        \"name\": \"Marian Bradley\"\n      }\n    ],\n    \"greeting\": \"Hello, Merrill Ray! You have 3 unread messages.\",\n    \"favoriteFruit\": \"strawberry\"\n  },\n  {\n    \"_id\": \"59b53bcb56ebb2118edadabb\",\n    \"index\": 28,\n    \"guid\": \"31fd77e0-df37-4030-b598-6469f87deaaa\",\n    \"isActive\": false,\n    \"balance\": \"$1,128.38\",\n    \"picture\": \"http://placehold.it/32x32\",\n    \"age\": 22,\n    \"eyeColor\": \"green\",\n    \"name\": \"Cunningham Blevins\",\n    \"gender\": \"male\",\n    \"company\": \"SHOPABOUT\",\n    \"email\": \"cunninghamblevins@shopabout.com\",\n    \"phone\": \"+1 (960) 458-2822\",\n    \"address\": \"730 Llama Court, Riner, Puerto Rico, 7836\",\n    \"about\": \"Dolor quis officia nulla dolor amet sint excepteur enim esse est do. Eu ex ut aliquip velit do sint ullamco laborum. Occaecat eiusmod eiusmod velit adipisicing sit. Mollit eu pariatur eu consequat dolore irure fugiat sunt eiusmod cillum duis adipisicing eiusmod. Do commodo nisi irure cillum magna nulla enim aliqua dolor ullamco dolore pariatur.\\r\\n\",\n    \"registered\": \"2016-09-06T04:22:46 -01:00\",\n    \"latitude\": 83.759644,\n    \"longitude\": -43.131498,\n    \"tags\": [\n      \"velit\",\n      \"fugiat\",\n      \"dolor\",\n      \"ad\",\n      \"elit\",\n      \"dolore\",\n      \"ea\"\n    ],\n    \"friends\": [\n      {\n        \"id\": 0,\n        \"name\": \"Sanford Shannon\"\n      },\n      {\n        \"id\": 1,\n        \"name\": \"Burt Cherry\"\n      },\n      {\n        \"id\": 2,\n        \"name\": \"Kline Hale\"\n      }\n    ],\n    \"greeting\": \"Hello, Cunningham Blevins! You have 10 unread messages.\",\n    \"favoriteFruit\": \"strawberry\"\n  },\n  {\n    \"_id\": \"59b53bcb90a0cd7d08d9bf70\",\n    \"index\": 29,\n    \"guid\": \"8fb07447-f204-4b08-975d-44052bc193eb\",\n    \"isActive\": false,\n    \"balance\": \"$3,739.37\",\n    \"picture\": \"http://placehold.it/32x32\",\n    \"age\": 36,\n    \"eyeColor\": \"brown\",\n    \"name\": \"Bonner Lane\",\n    \"gender\": \"male\",\n    \"company\": \"COMVEY\",\n    \"email\": \"bonnerlane@comvey.com\",\n    \"phone\": \"+1 (847) 514-2794\",\n    \"address\": \"269 Dupont Street, Cedarville, South Carolina, 6587\",\n    \"about\": \"Velit Lorem magna deserunt minim ea exercitation quis veniam. Culpa cillum do aliquip exercitation enim aute in incididunt nostrud esse nostrud ullamco in. Amet mollit laborum eu laborum magna. Duis ad proident cillum esse fugiat enim est sit commodo. Dolore consectetur ut duis deserunt elit aliqua ad fugiat consectetur. Est aute aliquip ea consequat reprehenderit eiusmod. Consectetur tempor consequat duis voluptate mollit elit labore voluptate do cillum ex.\\r\\n\",\n    \"registered\": \"2017-02-20T02:31:32 -00:00\",\n    \"latitude\": -71.168208,\n    \"longitude\": -127.709761,\n    \"tags\": [\n      \"voluptate\",\n      \"consequat\",\n      \"incididunt\",\n      \"occaecat\",\n      \"amet\",\n      \"consequat\",\n      \"id\"\n    ],\n    \"friends\": [\n      {\n        \"id\": 0,\n        \"name\": \"Josie Horne\"\n      },\n      {\n        \"id\": 1,\n        \"name\": \"Nichole Weiss\"\n      },\n      {\n        \"id\": 2,\n        \"name\": \"Kristina Davidson\"\n      }\n    ],\n    \"greeting\": \"Hello, Bonner Lane! You have 3 unread messages.\",\n    \"favoriteFruit\": \"apple\"\n  },\n  {\n    \"_id\": \"59b53bcb35a25f2270b16071\",\n    \"index\": 30,\n    \"guid\": \"267938cb-8119-471f-85af-aa7a668d65fd\",\n    \"isActive\": false,\n    \"balance\": \"$2,354.36\",\n    \"picture\": \"http://placehold.it/32x32\",\n    \"age\": 35,\n    \"eyeColor\": \"blue\",\n    \"name\": \"Nielsen Burnett\",\n    \"gender\": \"male\",\n    \"company\": \"TURNABOUT\",\n    \"email\": \"nielsenburnett@turnabout.com\",\n    \"phone\": \"+1 (901) 404-2369\",\n    \"address\": \"499 Hart Place, Chesterfield, Mississippi, 6896\",\n    \"about\": \"Sunt magna sint ea deserunt reprehenderit aliqua in et proident. Minim consectetur dolore et commodo. Voluptate consectetur qui occaecat dolore eiusmod proident fugiat aute nulla id ad culpa exercitation occaecat.\\r\\n\",\n    \"registered\": \"2015-02-20T12:03:11 -00:00\",\n    \"latitude\": -46.775808,\n    \"longitude\": 173.193033,\n    \"tags\": [\n      \"enim\",\n      \"dolor\",\n      \"duis\",\n      \"Lorem\",\n      \"in\",\n      \"reprehenderit\",\n      \"ullamco\"\n    ],\n    \"friends\": [\n      {\n        \"id\": 0,\n        \"name\": \"Barlow Mcfadden\"\n      },\n      {\n        \"id\": 1,\n        \"name\": \"Clarissa Charles\"\n      },\n      {\n        \"id\": 2,\n        \"name\": \"Bray Patel\"\n      }\n    ],\n    \"greeting\": \"Hello, Nielsen Burnett! You have 7 unread messages.\",\n    \"favoriteFruit\": \"strawberry\"\n  },\n  {\n    \"_id\": \"59b53bcbe85d478fcadd3603\",\n    \"index\": 31,\n    \"guid\": \"3be04d8f-e807-4ad6-8ebd-c23cdbfe3dc4\",\n    \"isActive\": false,\n    \"balance\": \"$1,972.40\",\n    \"picture\": \"http://placehold.it/32x32\",\n    \"age\": 37,\n    \"eyeColor\": \"blue\",\n    \"name\": \"Elaine Allison\",\n    \"gender\": \"female\",\n    \"company\": \"QUANTASIS\",\n    \"email\": \"elaineallison@quantasis.com\",\n    \"phone\": \"+1 (981) 596-2824\",\n    \"address\": \"921 Kent Avenue, Breinigsville, Wisconsin, 3750\",\n    \"about\": \"Minim cillum ea irure officia. Irure in dolor ea veniam adipisicing sint nisi amet ipsum excepteur nisi excepteur est deserunt. Consequat voluptate mollit sint magna Lorem in nulla proident Lorem. Proident est id esse ad ea. Dolore Lorem aliquip officia veniam anim velit et id ullamco et dolor eu aliqua quis. Dolore magna est mollit in ut ea voluptate nostrud do aliquip. In reprehenderit non eiusmod veniam ex.\\r\\n\",\n    \"registered\": \"2017-03-24T04:15:39 -00:00\",\n    \"latitude\": 7.656665,\n    \"longitude\": 56.755826,\n    \"tags\": [\n      \"nisi\",\n      \"labore\",\n      \"fugiat\",\n      \"ex\",\n      \"reprehenderit\",\n      \"nisi\",\n      \"sint\"\n    ],\n    \"friends\": [\n      {\n        \"id\": 0,\n        \"name\": \"Alta Bruce\"\n      },\n      {\n        \"id\": 1,\n        \"name\": \"Cora Ruiz\"\n      },\n      {\n        \"id\": 2,\n        \"name\": \"Mercer Barron\"\n      }\n    ],\n    \"greeting\": \"Hello, Elaine Allison! You have 1 unread messages.\",\n    \"favoriteFruit\": \"banana\"\n  },\n  {\n    \"_id\": \"59b53bcbf5dcc9341b3c298d\",\n    \"index\": 32,\n    \"guid\": \"bf62375b-123f-4c02-85e3-3a78c18e6f70\",\n    \"isActive\": false,\n    \"balance\": \"$1,895.96\",\n    \"picture\": \"http://placehold.it/32x32\",\n    \"age\": 28,\n    \"eyeColor\": \"brown\",\n    \"name\": \"Christa Robertson\",\n    \"gender\": \"female\",\n    \"company\": \"ICOLOGY\",\n    \"email\": \"christarobertson@icology.com\",\n    \"phone\": \"+1 (888) 410-3337\",\n    \"address\": \"989 Clara Street, Ogema, Indiana, 2922\",\n    \"about\": \"Enim mollit officia occaecat non nostrud ad cupidatat amet. Sunt ipsum proident consectetur voluptate id excepteur id magna. Do commodo culpa id esse officia cupidatat dolore duis non laboris veniam. Laboris ad dolor qui anim et ut dolor excepteur irure elit adipisicing ex labore eiusmod. Sunt minim velit nostrud irure quis consequat officia fugiat amet ipsum. Nostrud laboris do fugiat proident reprehenderit duis exercitation aute enim ex ullamco proident. Qui sint adipisicing occaecat aliqua non culpa esse id dolor voluptate ipsum deserunt in.\\r\\n\",\n    \"registered\": \"2015-02-16T07:12:55 -00:00\",\n    \"latitude\": 52.102423,\n    \"longitude\": -24.794434,\n    \"tags\": [\n      \"dolore\",\n      \"fugiat\",\n      \"aliqua\",\n      \"minim\",\n      \"pariatur\",\n      \"laborum\",\n      \"qui\"\n    ],\n    \"friends\": [\n      {\n        \"id\": 0,\n        \"name\": \"Cathy Cohen\"\n      },\n      {\n        \"id\": 1,\n        \"name\": \"Shawna Green\"\n      },\n      {\n        \"id\": 2,\n        \"name\": \"Ward Mckay\"\n      }\n    ],\n    \"greeting\": \"Hello, Christa Robertson! You have 9 unread messages.\",\n    \"favoriteFruit\": \"banana\"\n  },\n  {\n    \"_id\": \"59b53bcb8f369a2e50811288\",\n    \"index\": 33,\n    \"guid\": \"74275f14-281e-4519-a0c4-b708fa901d88\",\n    \"isActive\": true,\n    \"balance\": \"$2,269.82\",\n    \"picture\": \"http://placehold.it/32x32\",\n    \"age\": 36,\n    \"eyeColor\": \"green\",\n    \"name\": \"Castillo Kerr\",\n    \"gender\": \"male\",\n    \"company\": \"ZENTHALL\",\n    \"email\": \"castillokerr@zenthall.com\",\n    \"phone\": \"+1 (964) 406-2670\",\n    \"address\": \"210 Campus Road, Templeton, Tennessee, 2482\",\n    \"about\": \"Irure ut nisi adipisicing non duis mollit. Tempor deserunt ut nostrud ipsum enim dolore Lorem labore. Duis sint magna nisi et anim ex. Ea eu exercitation est laboris nostrud qui eiusmod. Ullamco amet ut Lorem eu adipisicing incididunt qui aliquip pariatur sint proident anim voluptate veniam. Excepteur aute velit deserunt deserunt et ex elit excepteur enim reprehenderit. Commodo ad aliquip Lorem excepteur reprehenderit quis in ea sint esse proident.\\r\\n\",\n    \"registered\": \"2016-05-03T04:24:26 -01:00\",\n    \"latitude\": -38.877683,\n    \"longitude\": -171.766918,\n    \"tags\": [\n      \"officia\",\n      \"aliquip\",\n      \"consequat\",\n      \"voluptate\",\n      \"cillum\",\n      \"do\",\n      \"officia\"\n    ],\n    \"friends\": [\n      {\n        \"id\": 0,\n        \"name\": \"Cara Hoffman\"\n      },\n      {\n        \"id\": 1,\n        \"name\": \"Joyner Beasley\"\n      },\n      {\n        \"id\": 2,\n        \"name\": \"Lucy Grimes\"\n      }\n    ],\n    \"greeting\": \"Hello, Castillo Kerr! You have 9 unread messages.\",\n    \"favoriteFruit\": \"strawberry\"\n  },\n  {\n    \"_id\": \"59b53bcbb2ac6162cf8d89a7\",\n    \"index\": 34,\n    \"guid\": \"3d62cd17-ac67-4b71-a5da-4ccef6cce1d0\",\n    \"isActive\": false,\n    \"balance\": \"$1,731.00\",\n    \"picture\": \"http://placehold.it/32x32\",\n    \"age\": 24,\n    \"eyeColor\": \"blue\",\n    \"name\": \"Melissa Gregory\",\n    \"gender\": \"female\",\n    \"company\": \"UPLINX\",\n    \"email\": \"melissagregory@uplinx.com\",\n    \"phone\": \"+1 (907) 532-2994\",\n    \"address\": \"394 Miller Avenue, Cashtown, Georgia, 520\",\n    \"about\": \"Consequat mollit occaecat proident officia reprehenderit. Ipsum minim ex reprehenderit et reprehenderit sunt. Esse ea quis nulla do. Cupidatat sit et tempor tempor voluptate qui est ad. Ad magna adipisicing excepteur excepteur ad quis. Fugiat laborum adipisicing do commodo ex qui ut minim ipsum commodo irure ex ea. Fugiat ad anim dolor do adipisicing veniam laboris laboris nostrud reprehenderit mollit eiusmod dolore laboris.\\r\\n\",\n    \"registered\": \"2016-03-22T12:23:21 -00:00\",\n    \"latitude\": -13.24058,\n    \"longitude\": 174.343852,\n    \"tags\": [\n      \"aliqua\",\n      \"veniam\",\n      \"do\",\n      \"tempor\",\n      \"voluptate\",\n      \"officia\",\n      \"id\"\n    ],\n    \"friends\": [\n      {\n        \"id\": 0,\n        \"name\": \"Mccall Baker\"\n      },\n      {\n        \"id\": 1,\n        \"name\": \"Elena Raymond\"\n      },\n      {\n        \"id\": 2,\n        \"name\": \"Harvey Hubbard\"\n      }\n    ],\n    \"greeting\": \"Hello, Melissa Gregory! You have 7 unread messages.\",\n    \"favoriteFruit\": \"banana\"\n  },\n  {\n    \"_id\": \"59b53bcb9bea1476ae4824c8\",\n    \"index\": 35,\n    \"guid\": \"705c7090-a759-43dc-b18c-63ad736d29ca\",\n    \"isActive\": false,\n    \"balance\": \"$2,004.78\",\n    \"picture\": \"http://placehold.it/32x32\",\n    \"age\": 37,\n    \"eyeColor\": \"brown\",\n    \"name\": \"Lancaster Welch\",\n    \"gender\": \"male\",\n    \"company\": \"JIMBIES\",\n    \"email\": \"lancasterwelch@jimbies.com\",\n    \"phone\": \"+1 (961) 509-2893\",\n    \"address\": \"477 Crystal Street, Lindcove, New Hampshire, 655\",\n    \"about\": \"Anim ex duis laboris non ullamco non deserunt magna ex voluptate mollit in excepteur. Sit excepteur proident ad magna esse elit veniam qui ad veniam cupidatat non duis. Eiusmod laboris id cupidatat exercitation quis adipisicing sunt eiusmod enim magna. Qui aliqua qui dolore enim veniam consequat ea cillum cupidatat voluptate excepteur in. Eu culpa anim veniam nisi officia consectetur ut exercitation fugiat quis sit ipsum enim quis. Lorem ut magna in sit.\\r\\n\",\n    \"registered\": \"2016-07-01T05:06:00 -01:00\",\n    \"latitude\": 29.49636,\n    \"longitude\": -45.617538,\n    \"tags\": [\n      \"adipisicing\",\n      \"enim\",\n      \"do\",\n      \"culpa\",\n      \"esse\",\n      \"proident\",\n      \"velit\"\n    ],\n    \"friends\": [\n      {\n        \"id\": 0,\n        \"name\": \"Whitehead Moss\"\n      },\n      {\n        \"id\": 1,\n        \"name\": \"Melisa Bridges\"\n      },\n      {\n        \"id\": 2,\n        \"name\": \"Helene Barrett\"\n      }\n    ],\n    \"greeting\": \"Hello, Lancaster Welch! You have 4 unread messages.\",\n    \"favoriteFruit\": \"strawberry\"\n  },\n  {\n    \"_id\": \"59b53bcb1dfb6733db2fc827\",\n    \"index\": 36,\n    \"guid\": \"0d80f8b7-650a-4492-b9ae-8c5d36bf2d83\",\n    \"isActive\": true,\n    \"balance\": \"$3,087.53\",\n    \"picture\": \"http://placehold.it/32x32\",\n    \"age\": 21,\n    \"eyeColor\": \"brown\",\n    \"name\": \"Clemons Juarez\",\n    \"gender\": \"male\",\n    \"company\": \"EMERGENT\",\n    \"email\": \"clemonsjuarez@emergent.com\",\n    \"phone\": \"+1 (899) 574-2444\",\n    \"address\": \"962 Seagate Avenue, Diaperville, Louisiana, 9282\",\n    \"about\": \"Labore adipisicing in enim eu laboris veniam minim sit do velit. Nulla amet ullamco anim cupidatat. Aliquip officia laborum nulla nisi aliqua dolore elit aute tempor ut culpa commodo. Esse cupidatat officia pariatur pariatur.\\r\\n\",\n    \"registered\": \"2015-07-29T04:09:12 -01:00\",\n    \"latitude\": 16.025236,\n    \"longitude\": -68.678922,\n    \"tags\": [\n      \"et\",\n      \"sunt\",\n      \"enim\",\n      \"dolor\",\n      \"labore\",\n      \"nostrud\",\n      \"adipisicing\"\n    ],\n    \"friends\": [\n      {\n        \"id\": 0,\n        \"name\": \"Dorothea Barnett\"\n      },\n      {\n        \"id\": 1,\n        \"name\": \"Terrie Knox\"\n      },\n      {\n        \"id\": 2,\n        \"name\": \"Dodson Dale\"\n      }\n    ],\n    \"greeting\": \"Hello, Clemons Juarez! You have 7 unread messages.\",\n    \"favoriteFruit\": \"apple\"\n  },\n  {\n    \"_id\": \"59b53bcba7232f419ad64f14\",\n    \"index\": 37,\n    \"guid\": \"15bec63f-2a77-45db-a3cf-11092f20cb9e\",\n    \"isActive\": false,\n    \"balance\": \"$3,716.74\",\n    \"picture\": \"http://placehold.it/32x32\",\n    \"age\": 29,\n    \"eyeColor\": \"green\",\n    \"name\": \"Hillary Waller\",\n    \"gender\": \"female\",\n    \"company\": \"MUSIX\",\n    \"email\": \"hillarywaller@musix.com\",\n    \"phone\": \"+1 (947) 549-3976\",\n    \"address\": \"601 Kay Court, Rockhill, Oklahoma, 5198\",\n    \"about\": \"Sit reprehenderit ad mollit reprehenderit do aliquip fugiat aute consectetur eu excepteur eiusmod dolor Lorem. Deserunt consectetur ex et deserunt velit quis excepteur labore deserunt cillum. Dolore mollit qui proident minim eiusmod.\\r\\n\",\n    \"registered\": \"2015-10-22T03:23:57 -01:00\",\n    \"latitude\": 2.128634,\n    \"longitude\": 43.198503,\n    \"tags\": [\n      \"duis\",\n      \"non\",\n      \"dolore\",\n      \"aliqua\",\n      \"culpa\",\n      \"proident\",\n      \"sint\"\n    ],\n    \"friends\": [\n      {\n        \"id\": 0,\n        \"name\": \"Vega Lawson\"\n      },\n      {\n        \"id\": 1,\n        \"name\": \"Phelps Wolf\"\n      },\n      {\n        \"id\": 2,\n        \"name\": \"Gloria Mcmillan\"\n      }\n    ],\n    \"greeting\": \"Hello, Hillary Waller! You have 10 unread messages.\",\n    \"favoriteFruit\": \"apple\"\n  },\n  {\n    \"_id\": \"59b53bcb1344ea6331b52625\",\n    \"index\": 38,\n    \"guid\": \"561edd27-6d57-4a6f-956c-f3bf54efe435\",\n    \"isActive\": true,\n    \"balance\": \"$3,213.23\",\n    \"picture\": \"http://placehold.it/32x32\",\n    \"age\": 32,\n    \"eyeColor\": \"brown\",\n    \"name\": \"Jackie Lott\",\n    \"gender\": \"female\",\n    \"company\": \"ORBIN\",\n    \"email\": \"jackielott@orbin.com\",\n    \"phone\": \"+1 (825) 509-2344\",\n    \"address\": \"921 Frost Street, Dubois, Alaska, 1796\",\n    \"about\": \"Reprehenderit veniam Lorem ea do proident in fugiat aliqua. Id proident nostrud aliqua tempor reprehenderit eiusmod ullamco velit duis. Anim ipsum nulla reprehenderit do exercitation consequat nisi in commodo qui fugiat nostrud.\\r\\n\",\n    \"registered\": \"2017-08-19T04:32:54 -01:00\",\n    \"latitude\": 23.292166,\n    \"longitude\": 35.845555,\n    \"tags\": [\n      \"dolore\",\n      \"veniam\",\n      \"labore\",\n      \"et\",\n      \"culpa\",\n      \"est\",\n      \"officia\"\n    ],\n    \"friends\": [\n      {\n        \"id\": 0,\n        \"name\": \"Diaz Warren\"\n      },\n      {\n        \"id\": 1,\n        \"name\": \"Sullivan Watkins\"\n      },\n      {\n        \"id\": 2,\n        \"name\": \"Maynard Page\"\n      }\n    ],\n    \"greeting\": \"Hello, Jackie Lott! You have 4 unread messages.\",\n    \"favoriteFruit\": \"apple\"\n  },\n  {\n    \"_id\": \"59b53bcb21e1aba2d54ad2f8\",\n    \"index\": 39,\n    \"guid\": \"c9ee8206-d3bd-48ae-9fda-5b5529ac4057\",\n    \"isActive\": false,\n    \"balance\": \"$3,035.61\",\n    \"picture\": \"http://placehold.it/32x32\",\n    \"age\": 29,\n    \"eyeColor\": \"green\",\n    \"name\": \"Flynn Pruitt\",\n    \"gender\": \"male\",\n    \"company\": \"ORBEAN\",\n    \"email\": \"flynnpruitt@orbean.com\",\n    \"phone\": \"+1 (866) 596-2533\",\n    \"address\": \"274 Ridgewood Place, Durham, North Dakota, 3534\",\n    \"about\": \"Commodo sint irure deserunt Lorem laboris laborum mollit ea ipsum incididunt laboris adipisicing proident. Velit tempor minim et occaecat exercitation et commodo consequat velit. Minim irure esse ullamco commodo labore ex mollit esse. Ipsum nostrud est ex Lorem culpa.\\r\\n\",\n    \"registered\": \"2015-06-20T09:17:37 -01:00\",\n    \"latitude\": -50.018521,\n    \"longitude\": 165.121492,\n    \"tags\": [\n      \"irure\",\n      \"ea\",\n      \"quis\",\n      \"dolore\",\n      \"irure\",\n      \"aliqua\",\n      \"pariatur\"\n    ],\n    \"friends\": [\n      {\n        \"id\": 0,\n        \"name\": \"Carla Snow\"\n      },\n      {\n        \"id\": 1,\n        \"name\": \"Cochran Thomas\"\n      },\n      {\n        \"id\": 2,\n        \"name\": \"Guy Roberts\"\n      }\n    ],\n    \"greeting\": \"Hello, Flynn Pruitt! You have 10 unread messages.\",\n    \"favoriteFruit\": \"banana\"\n  },\n  {\n    \"_id\": \"59b53bcb88a5fd7e5b5805c7\",\n    \"index\": 40,\n    \"guid\": \"ef10c0b3-7ab0-4313-b2b2-462164f5485a\",\n    \"isActive\": true,\n    \"balance\": \"$1,173.28\",\n    \"picture\": \"http://placehold.it/32x32\",\n    \"age\": 39,\n    \"eyeColor\": \"brown\",\n    \"name\": \"Shelby Albert\",\n    \"gender\": \"female\",\n    \"company\": \"HYDROCOM\",\n    \"email\": \"shelbyalbert@hydrocom.com\",\n    \"phone\": \"+1 (977) 400-2351\",\n    \"address\": \"393 Glendale Court, Catharine, Washington, 6629\",\n    \"about\": \"Do laborum exercitation eiusmod sunt esse laboris qui Lorem dolor amet consectetur id. Officia est exercitation proident pariatur culpa ea sint veniam reprehenderit aliquip. Laborum dolore ad mollit nostrud cillum ad tempor anim occaecat sit. Amet consequat eiusmod laboris consectetur.\\r\\n\",\n    \"registered\": \"2015-07-17T06:49:02 -01:00\",\n    \"latitude\": -32.156776,\n    \"longitude\": -68.42255,\n    \"tags\": [\n      \"laborum\",\n      \"dolor\",\n      \"sit\",\n      \"sit\",\n      \"ad\",\n      \"sunt\",\n      \"minim\"\n    ],\n    \"friends\": [\n      {\n        \"id\": 0,\n        \"name\": \"Huber Hahn\"\n      },\n      {\n        \"id\": 1,\n        \"name\": \"Felicia Mooney\"\n      },\n      {\n        \"id\": 2,\n        \"name\": \"Kathryn Alvarado\"\n      }\n    ],\n    \"greeting\": \"Hello, Shelby Albert! You have 1 unread messages.\",\n    \"favoriteFruit\": \"banana\"\n  },\n  {\n    \"_id\": \"59b53bcbacd63a0258d513a3\",\n    \"index\": 41,\n    \"guid\": \"7142ec6a-9741-41fd-8c8f-fba9cc5ff0ab\",\n    \"isActive\": true,\n    \"balance\": \"$3,196.96\",\n    \"picture\": \"http://placehold.it/32x32\",\n    \"age\": 34,\n    \"eyeColor\": \"brown\",\n    \"name\": \"Bailey Snyder\",\n    \"gender\": \"male\",\n    \"company\": \"ISOSURE\",\n    \"email\": \"baileysnyder@isosure.com\",\n    \"phone\": \"+1 (976) 469-3334\",\n    \"address\": \"754 Emerson Place, Stagecoach, New York, 1029\",\n    \"about\": \"Veniam dolore qui elit ea qui ipsum exercitation sunt sunt in ad mollit. Excepteur adipisicing et consectetur proident veniam laborum adipisicing consectetur eiusmod. Culpa consequat officia ipsum nisi proident proident velit. Fugiat commodo ad do commodo tempor proident excepteur mollit magna.\\r\\n\",\n    \"registered\": \"2015-09-25T01:25:56 -01:00\",\n    \"latitude\": -76.0324,\n    \"longitude\": -73.748444,\n    \"tags\": [\n      \"minim\",\n      \"adipisicing\",\n      \"Lorem\",\n      \"eu\",\n      \"ex\",\n      \"deserunt\",\n      \"eu\"\n    ],\n    \"friends\": [\n      {\n        \"id\": 0,\n        \"name\": \"Waters Hartman\"\n      },\n      {\n        \"id\": 1,\n        \"name\": \"Valdez Baird\"\n      },\n      {\n        \"id\": 2,\n        \"name\": \"Serena Mills\"\n      }\n    ],\n    \"greeting\": \"Hello, Bailey Snyder! You have 5 unread messages.\",\n    \"favoriteFruit\": \"strawberry\"\n  },\n  {\n    \"_id\": \"59b53bcba4a6b906f6c552ad\",\n    \"index\": 42,\n    \"guid\": \"46d7ec6e-a1f2-4133-bd5d-cc56e5102a00\",\n    \"isActive\": true,\n    \"balance\": \"$3,341.48\",\n    \"picture\": \"http://placehold.it/32x32\",\n    \"age\": 32,\n    \"eyeColor\": \"brown\",\n    \"name\": \"Erika Porter\",\n    \"gender\": \"female\",\n    \"company\": \"ZENTIME\",\n    \"email\": \"erikaporter@zentime.com\",\n    \"phone\": \"+1 (937) 468-3114\",\n    \"address\": \"917 Ovington Avenue, Stouchsburg, Alabama, 9680\",\n    \"about\": \"Consectetur reprehenderit nisi cupidatat deserunt nulla laboris ut. Nisi deserunt dolore occaecat fugiat esse pariatur quis non commodo laboris elit voluptate. Nulla ex laborum Lorem ipsum incididunt reprehenderit elit dolore ullamco amet duis esse est ullamco. Enim in mollit labore laborum sunt.\\r\\n\",\n    \"registered\": \"2015-01-22T11:40:33 -00:00\",\n    \"latitude\": 53.845955,\n    \"longitude\": -126.430992,\n    \"tags\": [\n      \"incididunt\",\n      \"elit\",\n      \"duis\",\n      \"deserunt\",\n      \"sint\",\n      \"labore\",\n      \"irure\"\n    ],\n    \"friends\": [\n      {\n        \"id\": 0,\n        \"name\": \"Monica Lyons\"\n      },\n      {\n        \"id\": 1,\n        \"name\": \"Katrina Brennan\"\n      },\n      {\n        \"id\": 2,\n        \"name\": \"Kim Francis\"\n      }\n    ],\n    \"greeting\": \"Hello, Erika Porter! You have 4 unread messages.\",\n    \"favoriteFruit\": \"strawberry\"\n  },\n  {\n    \"_id\": \"59b53bcb1c73edcfc9efe849\",\n    \"index\": 43,\n    \"guid\": \"84a42cb7-4fea-42c7-961d-2535547c818b\",\n    \"isActive\": true,\n    \"balance\": \"$1,840.08\",\n    \"picture\": \"http://placehold.it/32x32\",\n    \"age\": 29,\n    \"eyeColor\": \"brown\",\n    \"name\": \"Marjorie Craig\",\n    \"gender\": \"female\",\n    \"company\": \"PROGENEX\",\n    \"email\": \"marjoriecraig@progenex.com\",\n    \"phone\": \"+1 (898) 534-3929\",\n    \"address\": \"262 Exeter Street, Elliott, Arkansas, 9839\",\n    \"about\": \"Ipsum esse irure dolor consectetur amet ullamco. Ut nostrud anim occaecat dolor dolor sit adipisicing cupidatat. Veniam velit pariatur id magna in sit.\\r\\n\",\n    \"registered\": \"2014-11-10T05:13:50 -00:00\",\n    \"latitude\": 74.482858,\n    \"longitude\": 69.078973,\n    \"tags\": [\n      \"excepteur\",\n      \"cillum\",\n      \"minim\",\n      \"aliqua\",\n      \"exercitation\",\n      \"incididunt\",\n      \"dolor\"\n    ],\n    \"friends\": [\n      {\n        \"id\": 0,\n        \"name\": \"Horton Taylor\"\n      },\n      {\n        \"id\": 1,\n        \"name\": \"Melinda Ashley\"\n      },\n      {\n        \"id\": 2,\n        \"name\": \"Margie Roy\"\n      }\n    ],\n    \"greeting\": \"Hello, Marjorie Craig! You have 6 unread messages.\",\n    \"favoriteFruit\": \"banana\"\n  },\n  {\n    \"_id\": \"59b53bcb2edcfd9a5f058115\",\n    \"index\": 44,\n    \"guid\": \"8101a8ef-a578-4a86-9b90-204b2b6ca3bc\",\n    \"isActive\": false,\n    \"balance\": \"$1,295.45\",\n    \"picture\": \"http://placehold.it/32x32\",\n    \"age\": 20,\n    \"eyeColor\": \"blue\",\n    \"name\": \"Tina Browning\",\n    \"gender\": \"female\",\n    \"company\": \"KNOWLYSIS\",\n    \"email\": \"tinabrowning@knowlysis.com\",\n    \"phone\": \"+1 (878) 557-2240\",\n    \"address\": \"470 Lawton Street, Avoca, Northern Mariana Islands, 1174\",\n    \"about\": \"Officia quis reprehenderit eiusmod sit mollit duis minim duis elit exercitation sunt quis aliquip est. Velit esse occaecat irure deserunt amet dolore voluptate deserunt exercitation id. Dolor culpa dolor adipisicing do irure. Ullamco incididunt elit non mollit excepteur nisi proident ut eu sit dolor excepteur. Reprehenderit Lorem adipisicing deserunt eu labore laborum cillum ullamco nisi esse magna. Amet et ad nisi ad elit velit in in sunt veniam occaecat pariatur quis exercitation.\\r\\n\",\n    \"registered\": \"2015-10-18T08:14:25 -01:00\",\n    \"latitude\": 35.369634,\n    \"longitude\": -88.568524,\n    \"tags\": [\n      \"eu\",\n      \"veniam\",\n      \"quis\",\n      \"sint\",\n      \"excepteur\",\n      \"fugiat\",\n      \"minim\"\n    ],\n    \"friends\": [\n      {\n        \"id\": 0,\n        \"name\": \"Yolanda Mcgee\"\n      },\n      {\n        \"id\": 1,\n        \"name\": \"Tara Rich\"\n      },\n      {\n        \"id\": 2,\n        \"name\": \"Walton Maynard\"\n      }\n    ],\n    \"greeting\": \"Hello, Tina Browning! You have 8 unread messages.\",\n    \"favoriteFruit\": \"apple\"\n  },\n  {\n    \"_id\": \"59b53bcb3e923247d8ec4740\",\n    \"index\": 45,\n    \"guid\": \"b966f77e-3e7a-4bc1-8268-d15e38d760e2\",\n    \"isActive\": false,\n    \"balance\": \"$1,071.05\",\n    \"picture\": \"http://placehold.it/32x32\",\n    \"age\": 34,\n    \"eyeColor\": \"blue\",\n    \"name\": \"Estela Morrison\",\n    \"gender\": \"female\",\n    \"company\": \"DELPHIDE\",\n    \"email\": \"estelamorrison@delphide.com\",\n    \"phone\": \"+1 (895) 541-2685\",\n    \"address\": \"492 Ryder Avenue, Sims, West Virginia, 7864\",\n    \"about\": \"Est aliqua sit consectetur do occaecat ullamco commodo fugiat et. Culpa amet ipsum enim quis duis exercitation non nisi adipisicing aliquip incididunt irure. Labore aliqua sint nulla reprehenderit in reprehenderit tempor ullamco quis ipsum. Fugiat irure ut sit adipisicing cillum magna ad sit enim elit irure. Proident aliqua eu et anim est reprehenderit fugiat non. Commodo enim id nulla sit nisi. Excepteur tempor officia ipsum in pariatur.\\r\\n\",\n    \"registered\": \"2015-01-29T12:06:00 -00:00\",\n    \"latitude\": -31.693065,\n    \"longitude\": -53.009874,\n    \"tags\": [\n      \"magna\",\n      \"consequat\",\n      \"enim\",\n      \"velit\",\n      \"anim\",\n      \"velit\",\n      \"ad\"\n    ],\n    \"friends\": [\n      {\n        \"id\": 0,\n        \"name\": \"Callahan King\"\n      },\n      {\n        \"id\": 1,\n        \"name\": \"Key Wallace\"\n      },\n      {\n        \"id\": 2,\n        \"name\": \"Carney Arnold\"\n      }\n    ],\n    \"greeting\": \"Hello, Estela Morrison! You have 3 unread messages.\",\n    \"favoriteFruit\": \"apple\"\n  },\n  {\n    \"_id\": \"59b53bcb1526a6fceba75760\",\n    \"index\": 46,\n    \"guid\": \"5ef8b250-99fd-4d8e-99c0-bb5f3d3bdac3\",\n    \"isActive\": false,\n    \"balance\": \"$2,675.97\",\n    \"picture\": \"http://placehold.it/32x32\",\n    \"age\": 31,\n    \"eyeColor\": \"green\",\n    \"name\": \"Adela Ryan\",\n    \"gender\": \"female\",\n    \"company\": \"FLUMBO\",\n    \"email\": \"adelaryan@flumbo.com\",\n    \"phone\": \"+1 (906) 429-3206\",\n    \"address\": \"952 Richmond Street, Rodanthe, South Dakota, 2236\",\n    \"about\": \"Ea non aliquip fugiat Lorem magna pariatur excepteur officia qui quis officia occaecat quis est. Amet incididunt nisi duis commodo sint cillum tempor. Minim reprehenderit ut Lorem labore eu magna proident voluptate occaecat amet quis. Ipsum nulla ullamco ad enim duis velit eiusmod consectetur aliqua ad. Nisi aliquip esse proident nostrud officia non sit laboris amet excepteur dolor commodo ad. Cillum velit et ad aliquip esse mollit in enim tempor dolor. Aliqua esse excepteur mollit mollit.\\r\\n\",\n    \"registered\": \"2014-08-15T04:54:20 -01:00\",\n    \"latitude\": 49.702844,\n    \"longitude\": 154.358542,\n    \"tags\": [\n      \"nostrud\",\n      \"non\",\n      \"laboris\",\n      \"nostrud\",\n      \"eu\",\n      \"adipisicing\",\n      \"ad\"\n    ],\n    \"friends\": [\n      {\n        \"id\": 0,\n        \"name\": \"Moss Bright\"\n      },\n      {\n        \"id\": 1,\n        \"name\": \"Houston Glass\"\n      },\n      {\n        \"id\": 2,\n        \"name\": \"Cherry Moon\"\n      }\n    ],\n    \"greeting\": \"Hello, Adela Ryan! You have 2 unread messages.\",\n    \"favoriteFruit\": \"apple\"\n  },\n  {\n    \"_id\": \"59b53bcbb6aeae8f27f300a9\",\n    \"index\": 47,\n    \"guid\": \"8e8ffd1c-34dd-4984-9245-b4713cc73b00\",\n    \"isActive\": true,\n    \"balance\": \"$3,353.90\",\n    \"picture\": \"http://placehold.it/32x32\",\n    \"age\": 36,\n    \"eyeColor\": \"blue\",\n    \"name\": \"Cote Barlow\",\n    \"gender\": \"male\",\n    \"company\": \"BEZAL\",\n    \"email\": \"cotebarlow@bezal.com\",\n    \"phone\": \"+1 (987) 473-2295\",\n    \"address\": \"560 Emmons Avenue, Wolcott, Delaware, 8148\",\n    \"about\": \"Qui aliqua sit laboris eu consectetur commodo qui ullamco cupidatat id enim ex sit. Anim reprehenderit tempor ut fugiat. Sunt et consequat proident proident. Irure sunt adipisicing commodo do enim exercitation fugiat aliqua consequat anim do et sint. Enim excepteur reprehenderit deserunt pariatur do voluptate ullamco aliqua magna labore deserunt tempor id. Enim dolor nostrud qui ullamco cillum officia mollit.\\r\\n\",\n    \"registered\": \"2014-04-10T08:27:55 -01:00\",\n    \"latitude\": 66.218671,\n    \"longitude\": 64.565323,\n    \"tags\": [\n      \"magna\",\n      \"reprehenderit\",\n      \"velit\",\n      \"nulla\",\n      \"aliqua\",\n      \"quis\",\n      \"nisi\"\n    ],\n    \"friends\": [\n      {\n        \"id\": 0,\n        \"name\": \"Stark Yates\"\n      },\n      {\n        \"id\": 1,\n        \"name\": \"Ginger Wilkinson\"\n      },\n      {\n        \"id\": 2,\n        \"name\": \"Bradford Durham\"\n      }\n    ],\n    \"greeting\": \"Hello, Cote Barlow! You have 10 unread messages.\",\n    \"favoriteFruit\": \"apple\"\n  },\n  {\n    \"_id\": \"59b53bcbb025a60e792d23e8\",\n    \"index\": 48,\n    \"guid\": \"399c42d0-8971-45d8-ac59-af2f1ffaebd0\",\n    \"isActive\": true,\n    \"balance\": \"$3,820.26\",\n    \"picture\": \"http://placehold.it/32x32\",\n    \"age\": 32,\n    \"eyeColor\": \"brown\",\n    \"name\": \"Higgins Randall\",\n    \"gender\": \"male\",\n    \"company\": \"ECSTASIA\",\n    \"email\": \"higginsrandall@ecstasia.com\",\n    \"phone\": \"+1 (895) 474-3692\",\n    \"address\": \"325 John Street, Welch, Nebraska, 2056\",\n    \"about\": \"Cupidatat non minim occaecat proident enim consectetur occaecat Lorem duis ut. Quis incididunt nostrud amet ut laborum consequat aliquip excepteur. Dolor ipsum aute consectetur id quis Lorem culpa nostrud sint ipsum esse reprehenderit aliqua. Dolor id ex consequat nisi quis esse officia veniam. Sit amet cillum ea irure consectetur exercitation laboris culpa deserunt magna aute dolor. Cillum deserunt irure velit quis ipsum esse cillum cillum ullamco id.\\r\\n\",\n    \"registered\": \"2014-04-12T05:46:39 -01:00\",\n    \"latitude\": -75.882125,\n    \"longitude\": -169.69303,\n    \"tags\": [\n      \"deserunt\",\n      \"nostrud\",\n      \"do\",\n      \"est\",\n      \"laboris\",\n      \"excepteur\",\n      \"fugiat\"\n    ],\n    \"friends\": [\n      {\n        \"id\": 0,\n        \"name\": \"Tran Baldwin\"\n      },\n      {\n        \"id\": 1,\n        \"name\": \"James Joyner\"\n      },\n      {\n        \"id\": 2,\n        \"name\": \"Lessie Velez\"\n      }\n    ],\n    \"greeting\": \"Hello, Higgins Randall! You have 5 unread messages.\",\n    \"favoriteFruit\": \"banana\"\n  },\n  {\n    \"_id\": \"59b53bcb5f007cb90b5b92ad\",\n    \"index\": 49,\n    \"guid\": \"9ae4ab4d-ba1b-405e-a321-ccd78ef7b7e2\",\n    \"isActive\": true,\n    \"balance\": \"$3,496.51\",\n    \"picture\": \"http://placehold.it/32x32\",\n    \"age\": 39,\n    \"eyeColor\": \"blue\",\n    \"name\": \"Roach Mosley\",\n    \"gender\": \"male\",\n    \"company\": \"GADTRON\",\n    \"email\": \"roachmosley@gadtron.com\",\n    \"phone\": \"+1 (866) 580-2668\",\n    \"address\": \"709 Hendrickson Place, Mooresburg, California, 2507\",\n    \"about\": \"Et nostrud voluptate sunt laborum id enim irure pariatur ea anim ex Lorem est sint. Cupidatat aliqua fugiat proident sunt ea et non sint sint. Ut cupidatat aliquip magna ullamco sit ipsum duis mollit Lorem exercitation ut qui consectetur.\\r\\n\",\n    \"registered\": \"2016-08-14T07:34:15 -01:00\",\n    \"latitude\": 35.818251,\n    \"longitude\": -110.714479,\n    \"tags\": [\n      \"et\",\n      \"enim\",\n      \"fugiat\",\n      \"dolore\",\n      \"enim\",\n      \"voluptate\",\n      \"sit\"\n    ],\n    \"friends\": [\n      {\n        \"id\": 0,\n        \"name\": \"Olga Bryant\"\n      },\n      {\n        \"id\": 1,\n        \"name\": \"Patricia Gill\"\n      },\n      {\n        \"id\": 2,\n        \"name\": \"Mandy Gallagher\"\n      }\n    ],\n    \"greeting\": \"Hello, Roach Mosley! You have 2 unread messages.\",\n    \"favoriteFruit\": \"apple\"\n  },\n  {\n    \"_id\": \"59b53bcbc26b07d63737890c\",\n    \"index\": 50,\n    \"guid\": \"5b403f4d-e53f-470c-9842-b661322b636e\",\n    \"isActive\": false,\n    \"balance\": \"$2,414.71\",\n    \"picture\": \"http://placehold.it/32x32\",\n    \"age\": 22,\n    \"eyeColor\": \"green\",\n    \"name\": \"Cleo Glenn\",\n    \"gender\": \"female\",\n    \"company\": \"OVERPLEX\",\n    \"email\": \"cleoglenn@overplex.com\",\n    \"phone\": \"+1 (814) 562-3233\",\n    \"address\": \"181 Grand Street, Bawcomville, Ohio, 9691\",\n    \"about\": \"Laboris dolor ullamco ad elit mollit magna. Ipsum velit cillum et sint ut ipsum voluptate ea commodo cupidatat pariatur ipsum irure. Ad nostrud sit Lorem ex proident irure.\\r\\n\",\n    \"registered\": \"2016-02-16T07:07:22 -00:00\",\n    \"latitude\": -8.199302,\n    \"longitude\": 101.098002,\n    \"tags\": [\n      \"consequat\",\n      \"voluptate\",\n      \"enim\",\n      \"sint\",\n      \"Lorem\",\n      \"cupidatat\",\n      \"ipsum\"\n    ],\n    \"friends\": [\n      {\n        \"id\": 0,\n        \"name\": \"Ollie Stafford\"\n      },\n      {\n        \"id\": 1,\n        \"name\": \"Meredith Terrell\"\n      },\n      {\n        \"id\": 2,\n        \"name\": \"Mcgee Salazar\"\n      }\n    ],\n    \"greeting\": \"Hello, Cleo Glenn! You have 9 unread messages.\",\n    \"favoriteFruit\": \"banana\"\n  },\n  {\n    \"_id\": \"59b53bcb235cd8621ba76b75\",\n    \"index\": 51,\n    \"guid\": \"d05378a5-ec58-4631-9007-10eb3f9b63c4\",\n    \"isActive\": true,\n    \"balance\": \"$2,009.31\",\n    \"picture\": \"http://placehold.it/32x32\",\n    \"age\": 38,\n    \"eyeColor\": \"blue\",\n    \"name\": \"Little Beck\",\n    \"gender\": \"male\",\n    \"company\": \"GOGOL\",\n    \"email\": \"littlebeck@gogol.com\",\n    \"phone\": \"+1 (928) 571-3851\",\n    \"address\": \"709 Willmohr Street, Jenkinsville, Federated States Of Micronesia, 8660\",\n    \"about\": \"Exercitation occaecat minim aute ex quis in qui ex cillum aute velit. Velit qui sunt velit exercitation veniam incididunt culpa nostrud do tempor non eiusmod. Ad do ad velit eiusmod laborum laboris reprehenderit occaecat tempor do. Excepteur laboris consectetur id occaecat qui cupidatat enim ullamco anim anim. Laborum occaecat dolor aliqua ipsum dolor labore in elit sit.\\r\\n\",\n    \"registered\": \"2014-06-22T01:39:32 -01:00\",\n    \"latitude\": 38.221291,\n    \"longitude\": -172.966121,\n    \"tags\": [\n      \"labore\",\n      \"ullamco\",\n      \"mollit\",\n      \"pariatur\",\n      \"quis\",\n      \"ipsum\",\n      \"qui\"\n    ],\n    \"friends\": [\n      {\n        \"id\": 0,\n        \"name\": \"Mckay Skinner\"\n      },\n      {\n        \"id\": 1,\n        \"name\": \"Amalia Valdez\"\n      },\n      {\n        \"id\": 2,\n        \"name\": \"Vazquez Cox\"\n      }\n    ],\n    \"greeting\": \"Hello, Little Beck! You have 3 unread messages.\",\n    \"favoriteFruit\": \"banana\"\n  },\n  {\n    \"_id\": \"59b53bcbd3aa145075803296\",\n    \"index\": 52,\n    \"guid\": \"bb4f7000-690a-4c88-be2f-37aaf08d774a\",\n    \"isActive\": false,\n    \"balance\": \"$3,595.09\",\n    \"picture\": \"http://placehold.it/32x32\",\n    \"age\": 37,\n    \"eyeColor\": \"green\",\n    \"name\": \"Alexander Jensen\",\n    \"gender\": \"male\",\n    \"company\": \"QUILK\",\n    \"email\": \"alexanderjensen@quilk.com\",\n    \"phone\": \"+1 (939) 458-3826\",\n    \"address\": \"911 Mill Street, Wyoming, Palau, 9790\",\n    \"about\": \"Ex nostrud id qui pariatur ex dolor velit adipisicing consectetur sit velit ullamco do. Reprehenderit incididunt labore commodo Lorem ex. Ea excepteur ullamco velit id non. Aliquip exercitation pariatur ullamco fugiat ad ipsum aute. Ipsum reprehenderit et consectetur eiusmod reprehenderit id. Aute eiusmod eu id do ut incididunt dolor occaecat cupidatat labore excepteur enim commodo deserunt.\\r\\n\",\n    \"registered\": \"2014-08-29T01:54:27 -01:00\",\n    \"latitude\": -67.074581,\n    \"longitude\": 64.927721,\n    \"tags\": [\n      \"cupidatat\",\n      \"nisi\",\n      \"tempor\",\n      \"reprehenderit\",\n      \"id\",\n      \"eiusmod\",\n      \"ad\"\n    ],\n    \"friends\": [\n      {\n        \"id\": 0,\n        \"name\": \"Hayes Reynolds\"\n      },\n      {\n        \"id\": 1,\n        \"name\": \"Saundra Travis\"\n      },\n      {\n        \"id\": 2,\n        \"name\": \"Fuller Lucas\"\n      }\n    ],\n    \"greeting\": \"Hello, Alexander Jensen! You have 10 unread messages.\",\n    \"favoriteFruit\": \"apple\"\n  },\n  {\n    \"_id\": \"59b53bcb9eed49e2dc2bb115\",\n    \"index\": 53,\n    \"guid\": \"813e3bc6-1517-40ea-8506-03e41eb6ac3a\",\n    \"isActive\": true,\n    \"balance\": \"$1,392.46\",\n    \"picture\": \"http://placehold.it/32x32\",\n    \"age\": 33,\n    \"eyeColor\": \"green\",\n    \"name\": \"Rivas Rosales\",\n    \"gender\": \"male\",\n    \"company\": \"IPLAX\",\n    \"email\": \"rivasrosales@iplax.com\",\n    \"phone\": \"+1 (931) 434-2575\",\n    \"address\": \"124 Lake Avenue, Marysville, District Of Columbia, 5693\",\n    \"about\": \"Anim in duis adipisicing elit cupidatat aliqua tempor excepteur consectetur exercitation. Excepteur occaecat eiusmod incididunt anim sit in occaecat reprehenderit. Eu officia mollit ipsum aliquip adipisicing in ex consectetur enim Lorem irure pariatur irure ex. Ipsum nostrud labore commodo tempor. Occaecat ut sint tempor sunt anim nostrud nostrud excepteur duis aliqua consequat excepteur. Dolore ullamco enim irure magna anim nisi nostrud eiusmod proident.\\r\\n\",\n    \"registered\": \"2015-10-29T07:59:47 -00:00\",\n    \"latitude\": 35.539559,\n    \"longitude\": -171.582713,\n    \"tags\": [\n      \"qui\",\n      \"dolore\",\n      \"duis\",\n      \"nulla\",\n      \"est\",\n      \"ad\",\n      \"nulla\"\n    ],\n    \"friends\": [\n      {\n        \"id\": 0,\n        \"name\": \"Richard Chen\"\n      },\n      {\n        \"id\": 1,\n        \"name\": \"Pennington Garner\"\n      },\n      {\n        \"id\": 2,\n        \"name\": \"Ball Jackson\"\n      }\n    ],\n    \"greeting\": \"Hello, Rivas Rosales! You have 1 unread messages.\",\n    \"favoriteFruit\": \"apple\"\n  },\n  {\n    \"_id\": \"59b53bcb9e6f7027ee03d702\",\n    \"index\": 54,\n    \"guid\": \"577fde9f-2854-4414-9b96-06448ecb4488\",\n    \"isActive\": false,\n    \"balance\": \"$2,398.27\",\n    \"picture\": \"http://placehold.it/32x32\",\n    \"age\": 33,\n    \"eyeColor\": \"blue\",\n    \"name\": \"Jody Lancaster\",\n    \"gender\": \"female\",\n    \"company\": \"KEENGEN\",\n    \"email\": \"jodylancaster@keengen.com\",\n    \"phone\": \"+1 (898) 502-2640\",\n    \"address\": \"996 Quentin Street, Hoehne, Missouri, 4990\",\n    \"about\": \"Ipsum aute aute elit ea commodo amet laborum. Culpa quis reprehenderit proident consequat et enim. Adipisicing occaecat velit do labore eu eu id exercitation veniam ullamco elit. In ad Lorem ipsum proident enim. Tempor dolore Lorem et aute do excepteur dolore esse ad. Ut laboris pariatur elit officia anim consequat consequat officia eiusmod qui velit fugiat occaecat. Irure reprehenderit laborum cupidatat sint exercitation fugiat voluptate fugiat.\\r\\n\",\n    \"registered\": \"2015-08-06T02:13:32 -01:00\",\n    \"latitude\": 50.613083,\n    \"longitude\": 133.267848,\n    \"tags\": [\n      \"occaecat\",\n      \"dolore\",\n      \"quis\",\n      \"ullamco\",\n      \"ex\",\n      \"in\",\n      \"occaecat\"\n    ],\n    \"friends\": [\n      {\n        \"id\": 0,\n        \"name\": \"Barber Parks\"\n      },\n      {\n        \"id\": 1,\n        \"name\": \"Tamika Whitney\"\n      },\n      {\n        \"id\": 2,\n        \"name\": \"Boyle Melendez\"\n      }\n    ],\n    \"greeting\": \"Hello, Jody Lancaster! You have 6 unread messages.\",\n    \"favoriteFruit\": \"apple\"\n  },\n  {\n    \"_id\": \"59b53bcb218762e06bacfef0\",\n    \"index\": 55,\n    \"guid\": \"527e3426-cbe5-4fdc-ba02-0376d706325b\",\n    \"isActive\": true,\n    \"balance\": \"$2,126.86\",\n    \"picture\": \"http://placehold.it/32x32\",\n    \"age\": 22,\n    \"eyeColor\": \"brown\",\n    \"name\": \"Stout Lowe\",\n    \"gender\": \"male\",\n    \"company\": \"CHORIZON\",\n    \"email\": \"stoutlowe@chorizon.com\",\n    \"phone\": \"+1 (868) 502-2344\",\n    \"address\": \"228 Bliss Terrace, Loma, Illinois, 3866\",\n    \"about\": \"Nostrud et cillum nisi ea duis voluptate consequat excepteur labore laborum ut duis. Magna quis duis adipisicing duis elit nisi consequat duis laborum sint dolore. Esse adipisicing consectetur est esse amet ipsum Lorem aute incididunt amet. Enim est ea exercitation incididunt in.\\r\\n\",\n    \"registered\": \"2017-03-06T09:36:11 -00:00\",\n    \"latitude\": -33.017343,\n    \"longitude\": -113.928437,\n    \"tags\": [\n      \"labore\",\n      \"veniam\",\n      \"commodo\",\n      \"minim\",\n      \"qui\",\n      \"ad\",\n      \"et\"\n    ],\n    \"friends\": [\n      {\n        \"id\": 0,\n        \"name\": \"Trujillo Britt\"\n      },\n      {\n        \"id\": 1,\n        \"name\": \"Frye Moody\"\n      },\n      {\n        \"id\": 2,\n        \"name\": \"Gertrude Oneil\"\n      }\n    ],\n    \"greeting\": \"Hello, Stout Lowe! You have 1 unread messages.\",\n    \"favoriteFruit\": \"banana\"\n  },\n  {\n    \"_id\": \"59b53bcb16085e98ed2cea70\",\n    \"index\": 56,\n    \"guid\": \"3a610b27-0f08-447e-9216-39f2ad19273d\",\n    \"isActive\": true,\n    \"balance\": \"$1,799.97\",\n    \"picture\": \"http://placehold.it/32x32\",\n    \"age\": 38,\n    \"eyeColor\": \"brown\",\n    \"name\": \"Gwendolyn Farrell\",\n    \"gender\": \"female\",\n    \"company\": \"GEEKMOSIS\",\n    \"email\": \"gwendolynfarrell@geekmosis.com\",\n    \"phone\": \"+1 (807) 531-2875\",\n    \"address\": \"158 Chase Court, Riegelwood, Idaho, 6733\",\n    \"about\": \"Et Lorem reprehenderit aliqua pariatur velit dolor laboris fugiat. Consequat est dolor cillum consectetur cillum adipisicing laborum deserunt commodo non laboris. Non officia consequat consequat esse esse consequat. Eu fugiat minim ex deserunt.\\r\\n\",\n    \"registered\": \"2016-11-20T08:50:14 -00:00\",\n    \"latitude\": -38.469019,\n    \"longitude\": 102.32787,\n    \"tags\": [\n      \"ullamco\",\n      \"labore\",\n      \"dolor\",\n      \"consectetur\",\n      \"nisi\",\n      \"elit\",\n      \"cupidatat\"\n    ],\n    \"friends\": [\n      {\n        \"id\": 0,\n        \"name\": \"Blair Jordan\"\n      },\n      {\n        \"id\": 1,\n        \"name\": \"Wheeler Cannon\"\n      },\n      {\n        \"id\": 2,\n        \"name\": \"Dillon Fernandez\"\n      }\n    ],\n    \"greeting\": \"Hello, Gwendolyn Farrell! You have 4 unread messages.\",\n    \"favoriteFruit\": \"banana\"\n  },\n  {\n    \"_id\": \"59b53bcbd8b24e12c8941f72\",\n    \"index\": 57,\n    \"guid\": \"49be7373-8c53-4df1-9f56-ab81f211b8bf\",\n    \"isActive\": false,\n    \"balance\": \"$1,098.85\",\n    \"picture\": \"http://placehold.it/32x32\",\n    \"age\": 32,\n    \"eyeColor\": \"blue\",\n    \"name\": \"Gentry Anthony\",\n    \"gender\": \"male\",\n    \"company\": \"COGENTRY\",\n    \"email\": \"gentryanthony@cogentry.com\",\n    \"phone\": \"+1 (961) 457-3294\",\n    \"address\": \"807 Lewis Avenue, Aberdeen, Virgin Islands, 4388\",\n    \"about\": \"Qui cupidatat do veniam labore anim ullamco. Quis minim eu eiusmod labore consequat nulla labore. Est aliquip ut deserunt eiusmod occaecat laborum occaecat. Deserunt aliquip elit nostrud voluptate culpa magna occaecat non fugiat tempor labore elit cupidatat labore.\\r\\n\",\n    \"registered\": \"2016-04-30T03:18:07 -01:00\",\n    \"latitude\": 43.380138,\n    \"longitude\": -135.024374,\n    \"tags\": [\n      \"laboris\",\n      \"cillum\",\n      \"deserunt\",\n      \"excepteur\",\n      \"exercitation\",\n      \"do\",\n      \"tempor\"\n    ],\n    \"friends\": [\n      {\n        \"id\": 0,\n        \"name\": \"Janis Drake\"\n      },\n      {\n        \"id\": 1,\n        \"name\": \"Morse Huffman\"\n      },\n      {\n        \"id\": 2,\n        \"name\": \"Luna Davenport\"\n      }\n    ],\n    \"greeting\": \"Hello, Gentry Anthony! You have 7 unread messages.\",\n    \"favoriteFruit\": \"strawberry\"\n  },\n  {\n    \"_id\": \"59b53bcb21054f548ac53e2c\",\n    \"index\": 58,\n    \"guid\": \"efd6f059-3641-4df4-867c-58f72b8188dc\",\n    \"isActive\": false,\n    \"balance\": \"$3,534.32\",\n    \"picture\": \"http://placehold.it/32x32\",\n    \"age\": 26,\n    \"eyeColor\": \"brown\",\n    \"name\": \"Potter Hays\",\n    \"gender\": \"male\",\n    \"company\": \"ENTROFLEX\",\n    \"email\": \"potterhays@entroflex.com\",\n    \"phone\": \"+1 (905) 442-3818\",\n    \"address\": \"813 Erasmus Street, Northridge, Rhode Island, 5582\",\n    \"about\": \"Eiusmod Lorem laboris fugiat cupidatat qui dolore nulla nisi qui adipisicing. Cillum aute aliqua Lorem eiusmod. Ipsum sint eiusmod veniam pariatur excepteur officia consectetur deserunt. Cillum deserunt amet nostrud eiusmod deserunt labore nisi.\\r\\n\",\n    \"registered\": \"2017-05-24T04:37:42 -01:00\",\n    \"latitude\": 33.926864,\n    \"longitude\": -111.931141,\n    \"tags\": [\n      \"ipsum\",\n      \"commodo\",\n      \"dolor\",\n      \"nisi\",\n      \"dolore\",\n      \"laborum\",\n      \"incididunt\"\n    ],\n    \"friends\": [\n      {\n        \"id\": 0,\n        \"name\": \"Rosalie Livingston\"\n      },\n      {\n        \"id\": 1,\n        \"name\": \"Hannah Hardin\"\n      },\n      {\n        \"id\": 2,\n        \"name\": \"Madge Copeland\"\n      }\n    ],\n    \"greeting\": \"Hello, Potter Hays! You have 1 unread messages.\",\n    \"favoriteFruit\": \"apple\"\n  },\n  {\n    \"_id\": \"59b53bcbb0f4dd29011a5262\",\n    \"index\": 59,\n    \"guid\": \"530d5f1b-e3eb-49cc-8c7a-fc6f01b8ecdd\",\n    \"isActive\": false,\n    \"balance\": \"$3,138.39\",\n    \"picture\": \"http://placehold.it/32x32\",\n    \"age\": 20,\n    \"eyeColor\": \"blue\",\n    \"name\": \"Silvia Ortega\",\n    \"gender\": \"female\",\n    \"company\": \"CENTREXIN\",\n    \"email\": \"silviaortega@centrexin.com\",\n    \"phone\": \"+1 (980) 426-2287\",\n    \"address\": \"800 Williams Place, Chicopee, New Jersey, 3296\",\n    \"about\": \"Voluptate dolore do velit Lorem est voluptate ipsum aliquip ad officia exercitation laborum. Commodo consequat quis anim minim qui ut consectetur quis pariatur. Aute veniam sit Lorem voluptate esse amet. Esse cupidatat consequat cupidatat deserunt cillum magna ut reprehenderit esse non velit sint. Dolore nostrud ullamco ipsum culpa ad duis duis exercitation excepteur. Id consequat eu duis aliqua mollit.\\r\\n\",\n    \"registered\": \"2015-08-22T11:24:13 -01:00\",\n    \"latitude\": 81.63324,\n    \"longitude\": -118.965344,\n    \"tags\": [\n      \"laborum\",\n      \"excepteur\",\n      \"labore\",\n      \"ut\",\n      \"officia\",\n      \"in\",\n      \"eu\"\n    ],\n    \"friends\": [\n      {\n        \"id\": 0,\n        \"name\": \"Santiago Gentry\"\n      },\n      {\n        \"id\": 1,\n        \"name\": \"Melendez Pierce\"\n      },\n      {\n        \"id\": 2,\n        \"name\": \"Wood Stokes\"\n      }\n    ],\n    \"greeting\": \"Hello, Silvia Ortega! You have 8 unread messages.\",\n    \"favoriteFruit\": \"banana\"\n  },\n  {\n    \"_id\": \"59b53bcb2f824ae4587d2af7\",\n    \"index\": 60,\n    \"guid\": \"afe00138-7d3e-4a5b-9411-00d6155745e7\",\n    \"isActive\": true,\n    \"balance\": \"$2,759.26\",\n    \"picture\": \"http://placehold.it/32x32\",\n    \"age\": 34,\n    \"eyeColor\": \"green\",\n    \"name\": \"Combs Frazier\",\n    \"gender\": \"male\",\n    \"company\": \"ZIGGLES\",\n    \"email\": \"combsfrazier@ziggles.com\",\n    \"phone\": \"+1 (941) 567-3129\",\n    \"address\": \"154 Sedgwick Street, Elbert, Kentucky, 5956\",\n    \"about\": \"Anim incididunt dolor in eiusmod nulla do. Non consequat fugiat mollit laborum laborum occaecat nisi sunt Lorem consectetur laborum. Consequat laborum cupidatat dolore excepteur consequat adipisicing voluptate veniam aliquip elit do. Sint ut proident ex ea dolor aute fugiat et consequat minim pariatur do. Commodo laboris ea labore eiusmod labore fugiat consectetur enim. Cupidatat occaecat non minim dolor est commodo laborum excepteur anim. Eiusmod laboris laboris ullamco aliquip reprehenderit velit commodo aliqua magna anim irure non Lorem esse.\\r\\n\",\n    \"registered\": \"2016-07-23T05:27:36 -01:00\",\n    \"latitude\": -60.790167,\n    \"longitude\": -6.995975,\n    \"tags\": [\n      \"eu\",\n      \"irure\",\n      \"cupidatat\",\n      \"pariatur\",\n      \"sint\",\n      \"dolor\",\n      \"aliqua\"\n    ],\n    \"friends\": [\n      {\n        \"id\": 0,\n        \"name\": \"Karin Cortez\"\n      },\n      {\n        \"id\": 1,\n        \"name\": \"Ellen Ramos\"\n      },\n      {\n        \"id\": 2,\n        \"name\": \"Lynda Underwood\"\n      }\n    ],\n    \"greeting\": \"Hello, Combs Frazier! You have 6 unread messages.\",\n    \"favoriteFruit\": \"strawberry\"\n  },\n  {\n    \"_id\": \"59b53bcbebab6fc06e22bcf4\",\n    \"index\": 61,\n    \"guid\": \"30d1f10f-aad1-41f4-8621-5280977328d7\",\n    \"isActive\": true,\n    \"balance\": \"$2,802.02\",\n    \"picture\": \"http://placehold.it/32x32\",\n    \"age\": 33,\n    \"eyeColor\": \"blue\",\n    \"name\": \"Lyons Mccormick\",\n    \"gender\": \"male\",\n    \"company\": \"DECRATEX\",\n    \"email\": \"lyonsmccormick@decratex.com\",\n    \"phone\": \"+1 (978) 591-2593\",\n    \"address\": \"574 Kingsland Avenue, Calvary, Arizona, 2085\",\n    \"about\": \"Dolore cupidatat magna esse est est eiusmod non fugiat ipsum minim non duis do elit. Ut ad voluptate quis ea nostrud duis deserunt sit aliqua est sit consectetur. Aute eiusmod Lorem labore sint qui commodo. Quis quis ut minim ullamco. Nostrud in et enim sunt do voluptate qui nisi laborum non excepteur.\\r\\n\",\n    \"registered\": \"2014-08-18T12:17:12 -01:00\",\n    \"latitude\": 3.509991,\n    \"longitude\": -45.531481,\n    \"tags\": [\n      \"aliqua\",\n      \"culpa\",\n      \"et\",\n      \"eiusmod\",\n      \"nulla\",\n      \"esse\",\n      \"ad\"\n    ],\n    \"friends\": [\n      {\n        \"id\": 0,\n        \"name\": \"Rollins Owens\"\n      },\n      {\n        \"id\": 1,\n        \"name\": \"Erna Kim\"\n      },\n      {\n        \"id\": 2,\n        \"name\": \"Ferrell Blackburn\"\n      }\n    ],\n    \"greeting\": \"Hello, Lyons Mccormick! You have 3 unread messages.\",\n    \"favoriteFruit\": \"strawberry\"\n  },\n  {\n    \"_id\": \"59b53bcb4179085566efccff\",\n    \"index\": 62,\n    \"guid\": \"00011346-88e6-4501-9736-1458bea145f9\",\n    \"isActive\": false,\n    \"balance\": \"$3,659.33\",\n    \"picture\": \"http://placehold.it/32x32\",\n    \"age\": 40,\n    \"eyeColor\": \"green\",\n    \"name\": \"Cornelia Bray\",\n    \"gender\": \"female\",\n    \"company\": \"COMVEYER\",\n    \"email\": \"corneliabray@comveyer.com\",\n    \"phone\": \"+1 (959) 580-2744\",\n    \"address\": \"532 Butler Street, Crumpler, American Samoa, 8116\",\n    \"about\": \"Commodo commodo id amet minim labore mollit nulla et magna irure duis laboris. Culpa sunt Lorem eu cupidatat do aute nulla esse duis non velit incididunt commodo nulla. Pariatur in labore Lorem id in sit magna enim. Lorem Lorem exercitation velit sint do ullamco. Ipsum quis consequat elit nisi dolore ipsum. Non cillum est ad est sint nisi et. Reprehenderit tempor do minim ullamco consectetur.\\r\\n\",\n    \"registered\": \"2016-12-09T07:09:57 -00:00\",\n    \"latitude\": 2.702237,\n    \"longitude\": -80.758148,\n    \"tags\": [\n      \"cillum\",\n      \"excepteur\",\n      \"enim\",\n      \"amet\",\n      \"ipsum\",\n      \"mollit\",\n      \"dolore\"\n    ],\n    \"friends\": [\n      {\n        \"id\": 0,\n        \"name\": \"Hazel Steele\"\n      },\n      {\n        \"id\": 1,\n        \"name\": \"Beach Harmon\"\n      },\n      {\n        \"id\": 2,\n        \"name\": \"Olive Burton\"\n      }\n    ],\n    \"greeting\": \"Hello, Cornelia Bray! You have 7 unread messages.\",\n    \"favoriteFruit\": \"banana\"\n  },\n  {\n    \"_id\": \"59b53bcb3405dcede35b5a96\",\n    \"index\": 63,\n    \"guid\": \"db2142fc-3e37-4bd8-9c17-9891fe34a3b2\",\n    \"isActive\": true,\n    \"balance\": \"$1,405.92\",\n    \"picture\": \"http://placehold.it/32x32\",\n    \"age\": 36,\n    \"eyeColor\": \"brown\",\n    \"name\": \"Mcdonald Wade\",\n    \"gender\": \"male\",\n    \"company\": \"COMVERGES\",\n    \"email\": \"mcdonaldwade@comverges.com\",\n    \"phone\": \"+1 (937) 425-2339\",\n    \"address\": \"793 Elliott Walk, Waumandee, Massachusetts, 219\",\n    \"about\": \"Tempor irure minim proident adipisicing ad veniam magna minim nulla non sunt. Et eu ad non ea in occaecat irure dolore ex ipsum sunt. Adipisicing quis fugiat nostrud proident ullamco enim nostrud. Deserunt excepteur dolore anim sunt deserunt dolore non exercitation ex cupidatat eiusmod do. Tempor fugiat elit commodo id.\\r\\n\",\n    \"registered\": \"2015-04-21T01:38:34 -01:00\",\n    \"latitude\": -86.33219,\n    \"longitude\": -116.14479,\n    \"tags\": [\n      \"ex\",\n      \"in\",\n      \"et\",\n      \"est\",\n      \"officia\",\n      \"Lorem\",\n      \"qui\"\n    ],\n    \"friends\": [\n      {\n        \"id\": 0,\n        \"name\": \"Mariana Massey\"\n      },\n      {\n        \"id\": 1,\n        \"name\": \"Rosanne Strong\"\n      },\n      {\n        \"id\": 2,\n        \"name\": \"Fitzpatrick Riddle\"\n      }\n    ],\n    \"greeting\": \"Hello, Mcdonald Wade! You have 2 unread messages.\",\n    \"favoriteFruit\": \"apple\"\n  },\n  {\n    \"_id\": \"59b53bcb75995c65fa8a794e\",\n    \"index\": 64,\n    \"guid\": \"2d6b262c-1f4c-4818-8e0c-de99bc67de84\",\n    \"isActive\": false,\n    \"balance\": \"$3,597.88\",\n    \"picture\": \"http://placehold.it/32x32\",\n    \"age\": 20,\n    \"eyeColor\": \"green\",\n    \"name\": \"Leanne Briggs\",\n    \"gender\": \"female\",\n    \"company\": \"NAMEGEN\",\n    \"email\": \"leannebriggs@namegen.com\",\n    \"phone\": \"+1 (821) 566-2729\",\n    \"address\": \"126 Havens Place, Forbestown, Maine, 4804\",\n    \"about\": \"Exercitation sunt aliquip culpa cupidatat ad consectetur est dolor labore. Officia excepteur duis consectetur minim aliqua consectetur elit excepteur ipsum eiusmod aliquip mollit est. Incididunt pariatur id eiusmod nostrud nostrud Lorem culpa commodo fugiat officia ipsum aliquip. Reprehenderit aliquip irure ullamco proident elit minim ullamco sit pariatur dolore. Cillum voluptate anim amet cillum aliquip reprehenderit aliqua magna occaecat sit adipisicing laboris ea. Veniam aute dolore aliqua consectetur amet voluptate. Aliquip pariatur velit sit cillum nulla nostrud elit qui ipsum.\\r\\n\",\n    \"registered\": \"2017-01-31T02:36:59 -00:00\",\n    \"latitude\": -15.400663,\n    \"longitude\": 132.732197,\n    \"tags\": [\n      \"aute\",\n      \"quis\",\n      \"mollit\",\n      \"quis\",\n      \"pariatur\",\n      \"commodo\",\n      \"cupidatat\"\n    ],\n    \"friends\": [\n      {\n        \"id\": 0,\n        \"name\": \"Moran Curry\"\n      },\n      {\n        \"id\": 1,\n        \"name\": \"Mullins Ramsey\"\n      },\n      {\n        \"id\": 2,\n        \"name\": \"Pamela Perez\"\n      }\n    ],\n    \"greeting\": \"Hello, Leanne Briggs! You have 3 unread messages.\",\n    \"favoriteFruit\": \"banana\"\n  },\n  {\n    \"_id\": \"59b53bcbe6083b02455e297a\",\n    \"index\": 65,\n    \"guid\": \"114311fc-f902-4429-9713-509ccb6ad25e\",\n    \"isActive\": false,\n    \"balance\": \"$1,225.19\",\n    \"picture\": \"http://placehold.it/32x32\",\n    \"age\": 30,\n    \"eyeColor\": \"brown\",\n    \"name\": \"Lila Schmidt\",\n    \"gender\": \"female\",\n    \"company\": \"NEPTIDE\",\n    \"email\": \"lilaschmidt@neptide.com\",\n    \"phone\": \"+1 (904) 414-2477\",\n    \"address\": \"263 Degraw Street, Soham, Guam, 3945\",\n    \"about\": \"Anim culpa proident laboris non laboris. Velit nisi non nulla est Lorem laboris eu aliquip ex ea cupidatat aute nisi. Anim dolor sint pariatur cillum nisi nisi culpa. Fugiat velit non et anim non ex sint sint. Quis ex non labore commodo sit mollit eiusmod magna cillum laboris amet. Esse consequat qui velit et dolore pariatur id fugiat anim occaecat duis culpa in laborum.\\r\\n\",\n    \"registered\": \"2016-12-27T08:25:17 -00:00\",\n    \"latitude\": 21.703515,\n    \"longitude\": -54.394255,\n    \"tags\": [\n      \"incididunt\",\n      \"laboris\",\n      \"nulla\",\n      \"fugiat\",\n      \"aliquip\",\n      \"tempor\",\n      \"do\"\n    ],\n    \"friends\": [\n      {\n        \"id\": 0,\n        \"name\": \"Jordan Palmer\"\n      },\n      {\n        \"id\": 1,\n        \"name\": \"Leon Mcleod\"\n      },\n      {\n        \"id\": 2,\n        \"name\": \"Mcbride Simon\"\n      }\n    ],\n    \"greeting\": \"Hello, Lila Schmidt! You have 5 unread messages.\",\n    \"favoriteFruit\": \"strawberry\"\n  },\n  {\n    \"_id\": \"59b53bcb48e4a6fa9e53affd\",\n    \"index\": 66,\n    \"guid\": \"34a3b2a0-9e97-4dab-881d-bc809370ed0b\",\n    \"isActive\": true,\n    \"balance\": \"$2,539.75\",\n    \"picture\": \"http://placehold.it/32x32\",\n    \"age\": 38,\n    \"eyeColor\": \"green\",\n    \"name\": \"Melba House\",\n    \"gender\": \"female\",\n    \"company\": \"NETUR\",\n    \"email\": \"melbahouse@netur.com\",\n    \"phone\": \"+1 (975) 559-3215\",\n    \"address\": \"688 Tillary Street, Ruffin, Texas, 920\",\n    \"about\": \"Ad non aliquip tempor aute ea anim cillum officia qui proident esse culpa reprehenderit. Consectetur eiusmod quis velit sint dolore est velit voluptate laboris sunt occaecat consectetur consectetur ipsum. Proident sint elit dolor amet occaecat. Dolore reprehenderit consectetur commodo mollit pariatur aliqua magna fugiat nostrud cupidatat. Nostrud do esse laboris ipsum ullamco dolore officia. Ut labore elit non labore aute magna pariatur laborum ullamco velit laborum duis elit do. Ullamco labore nulla eiusmod sint.\\r\\n\",\n    \"registered\": \"2016-04-17T08:18:11 -01:00\",\n    \"latitude\": 87.963824,\n    \"longitude\": 65.388805,\n    \"tags\": [\n      \"est\",\n      \"cillum\",\n      \"veniam\",\n      \"exercitation\",\n      \"aliqua\",\n      \"velit\",\n      \"nulla\"\n    ],\n    \"friends\": [\n      {\n        \"id\": 0,\n        \"name\": \"Erica Moran\"\n      },\n      {\n        \"id\": 1,\n        \"name\": \"Peck Rios\"\n      },\n      {\n        \"id\": 2,\n        \"name\": \"Irene Wiley\"\n      }\n    ],\n    \"greeting\": \"Hello, Melba House! You have 3 unread messages.\",\n    \"favoriteFruit\": \"banana\"\n  },\n  {\n    \"_id\": \"59b53bcb23c882b00ccbeb78\",\n    \"index\": 67,\n    \"guid\": \"43870cc3-e38d-40e7-ba96-33fff3de9315\",\n    \"isActive\": false,\n    \"balance\": \"$2,394.68\",\n    \"picture\": \"http://placehold.it/32x32\",\n    \"age\": 20,\n    \"eyeColor\": \"brown\",\n    \"name\": \"Vance Thompson\",\n    \"gender\": \"male\",\n    \"company\": \"BIOSPAN\",\n    \"email\": \"vancethompson@biospan.com\",\n    \"phone\": \"+1 (930) 463-3961\",\n    \"address\": \"573 Dearborn Court, Jacumba, Colorado, 1903\",\n    \"about\": \"Duis aliquip aliquip ut pariatur cupidatat magna enim qui. Culpa tempor laboris et culpa eiusmod. Aute excepteur nulla ullamco nulla aute cillum laborum irure eiusmod. Id exercitation nostrud veniam elit eu excepteur quis id ad. Aute velit sit nulla incididunt amet consectetur anim.\\r\\n\",\n    \"registered\": \"2015-01-06T09:28:15 -00:00\",\n    \"latitude\": 16.206121,\n    \"longitude\": 2.066817,\n    \"tags\": [\n      \"proident\",\n      \"officia\",\n      \"do\",\n      \"irure\",\n      \"qui\",\n      \"sint\",\n      \"consequat\"\n    ],\n    \"friends\": [\n      {\n        \"id\": 0,\n        \"name\": \"Marilyn Justice\"\n      },\n      {\n        \"id\": 1,\n        \"name\": \"Pacheco Frank\"\n      },\n      {\n        \"id\": 2,\n        \"name\": \"Warner Neal\"\n      }\n    ],\n    \"greeting\": \"Hello, Vance Thompson! You have 8 unread messages.\",\n    \"favoriteFruit\": \"banana\"\n  },\n  {\n    \"_id\": \"59b53bcb41a2c54c5e49f6e2\",\n    \"index\": 68,\n    \"guid\": \"f0ac1d16-e1c6-4208-8964-a7f523b09527\",\n    \"isActive\": false,\n    \"balance\": \"$2,631.00\",\n    \"picture\": \"http://placehold.it/32x32\",\n    \"age\": 36,\n    \"eyeColor\": \"brown\",\n    \"name\": \"Burton Dorsey\",\n    \"gender\": \"male\",\n    \"company\": \"ROTODYNE\",\n    \"email\": \"burtondorsey@rotodyne.com\",\n    \"phone\": \"+1 (824) 463-3076\",\n    \"address\": \"914 Belmont Avenue, Takilma, Utah, 4995\",\n    \"about\": \"Fugiat irure proident quis duis laborum occaecat. Irure voluptate deserunt dolor reprehenderit do anim deserunt adipisicing. Ex in quis eu irure qui laborum duis do occaecat. Reprehenderit commodo commodo officia do incididunt velit ipsum. Voluptate elit ullamco cupidatat enim duis magna consequat ipsum mollit.\\r\\n\",\n    \"registered\": \"2015-06-21T09:38:28 -01:00\",\n    \"latitude\": 29.679351,\n    \"longitude\": 55.009156,\n    \"tags\": [\n      \"id\",\n      \"anim\",\n      \"do\",\n      \"eiusmod\",\n      \"sunt\",\n      \"dolor\",\n      \"ullamco\"\n    ],\n    \"friends\": [\n      {\n        \"id\": 0,\n        \"name\": \"Estrada Frederick\"\n      },\n      {\n        \"id\": 1,\n        \"name\": \"Pratt Bernard\"\n      },\n      {\n        \"id\": 2,\n        \"name\": \"Bobbie Pope\"\n      }\n    ],\n    \"greeting\": \"Hello, Burton Dorsey! You have 1 unread messages.\",\n    \"favoriteFruit\": \"apple\"\n  },\n  {\n    \"_id\": \"59b53bcbd77a0c5752db5b53\",\n    \"index\": 69,\n    \"guid\": \"9c501418-7230-4ccb-832a-d344a905dd2d\",\n    \"isActive\": true,\n    \"balance\": \"$3,815.52\",\n    \"picture\": \"http://placehold.it/32x32\",\n    \"age\": 27,\n    \"eyeColor\": \"brown\",\n    \"name\": \"Hatfield Ball\",\n    \"gender\": \"male\",\n    \"company\": \"ZINCA\",\n    \"email\": \"hatfieldball@zinca.com\",\n    \"phone\": \"+1 (989) 422-3125\",\n    \"address\": \"768 Guernsey Street, Brewster, Montana, 139\",\n    \"about\": \"Aute eiusmod eu nisi ut cupidatat. Duis minim sunt amet labore. Ullamco nisi Lorem ipsum qui anim id laboris incididunt excepteur id culpa sit excepteur dolore. Nulla eu excepteur do id quis. Ullamco culpa cupidatat culpa non aliquip tempor duis ad et sunt minim consectetur. Aliquip sit aliqua nisi sunt elit ea.\\r\\n\",\n    \"registered\": \"2014-06-10T12:39:52 -01:00\",\n    \"latitude\": 56.126846,\n    \"longitude\": 40.545126,\n    \"tags\": [\n      \"amet\",\n      \"veniam\",\n      \"dolor\",\n      \"in\",\n      \"excepteur\",\n      \"nulla\",\n      \"qui\"\n    ],\n    \"friends\": [\n      {\n        \"id\": 0,\n        \"name\": \"Stewart Peterson\"\n      },\n      {\n        \"id\": 1,\n        \"name\": \"Heather Mayo\"\n      },\n      {\n        \"id\": 2,\n        \"name\": \"Murray Brady\"\n      }\n    ],\n    \"greeting\": \"Hello, Hatfield Ball! You have 8 unread messages.\",\n    \"favoriteFruit\": \"apple\"\n  },\n  {\n    \"_id\": \"59b53bcb1fec7ace6110275b\",\n    \"index\": 70,\n    \"guid\": \"f7def176-2ac0-4c08-b1dc-d51a5a67dc0b\",\n    \"isActive\": true,\n    \"balance\": \"$2,019.28\",\n    \"picture\": \"http://placehold.it/32x32\",\n    \"age\": 22,\n    \"eyeColor\": \"blue\",\n    \"name\": \"Hill Shelton\",\n    \"gender\": \"male\",\n    \"company\": \"EMTRAK\",\n    \"email\": \"hillshelton@emtrak.com\",\n    \"phone\": \"+1 (868) 415-2186\",\n    \"address\": \"231 Loring Avenue, Jeff, Maryland, 4988\",\n    \"about\": \"Veniam id eu deserunt laborum. Veniam labore anim amet sunt officia ea cupidatat deserunt. Aute proident commodo est mollit amet laborum dolore pariatur culpa. Ad adipisicing ea laboris excepteur ex id est magna reprehenderit. Excepteur aliqua do commodo cupidatat velit do.\\r\\n\",\n    \"registered\": \"2016-09-29T01:14:11 -01:00\",\n    \"latitude\": 9.893931,\n    \"longitude\": 1.018174,\n    \"tags\": [\n      \"anim\",\n      \"fugiat\",\n      \"culpa\",\n      \"mollit\",\n      \"do\",\n      \"voluptate\",\n      \"consequat\"\n    ],\n    \"friends\": [\n      {\n        \"id\": 0,\n        \"name\": \"Glass Walter\"\n      },\n      {\n        \"id\": 1,\n        \"name\": \"Joyce Church\"\n      },\n      {\n        \"id\": 2,\n        \"name\": \"Kari Bowen\"\n      }\n    ],\n    \"greeting\": \"Hello, Hill Shelton! You have 8 unread messages.\",\n    \"favoriteFruit\": \"apple\"\n  },\n  {\n    \"_id\": \"59b53bcb0018db268644035f\",\n    \"index\": 71,\n    \"guid\": \"892c26d8-1618-4249-a5cd-2e4f72a42917\",\n    \"isActive\": true,\n    \"balance\": \"$3,320.73\",\n    \"picture\": \"http://placehold.it/32x32\",\n    \"age\": 22,\n    \"eyeColor\": \"brown\",\n    \"name\": \"Jamie Curtis\",\n    \"gender\": \"female\",\n    \"company\": \"OPTICON\",\n    \"email\": \"jamiecurtis@opticon.com\",\n    \"phone\": \"+1 (987) 560-2955\",\n    \"address\": \"798 Woodpoint Road, Zarephath, Connecticut, 258\",\n    \"about\": \"Occaecat duis commodo et eiusmod amet. Et minim aliqua commodo ipsum dolore cupidatat aute quis sint ullamco laborum. Culpa consequat dolor sunt mollit magna ad nisi cillum aliqua eu veniam nostrud. Velit tempor consequat culpa et irure. Aute culpa duis cupidatat nulla ut et incididunt officia magna irure enim do esse.\\r\\n\",\n    \"registered\": \"2016-05-17T11:58:35 -01:00\",\n    \"latitude\": -25.764923,\n    \"longitude\": 176.326556,\n    \"tags\": [\n      \"veniam\",\n      \"reprehenderit\",\n      \"reprehenderit\",\n      \"sunt\",\n      \"ea\",\n      \"non\",\n      \"veniam\"\n    ],\n    \"friends\": [\n      {\n        \"id\": 0,\n        \"name\": \"Katy Mccoy\"\n      },\n      {\n        \"id\": 1,\n        \"name\": \"Marianne Merrill\"\n      },\n      {\n        \"id\": 2,\n        \"name\": \"Bass Pugh\"\n      }\n    ],\n    \"greeting\": \"Hello, Jamie Curtis! You have 3 unread messages.\",\n    \"favoriteFruit\": \"apple\"\n  },\n  {\n    \"_id\": \"59b53bcb66c0788939f5655d\",\n    \"index\": 72,\n    \"guid\": \"2d7d871b-187c-4eea-9abc-7d1b4a70dd40\",\n    \"isActive\": false,\n    \"balance\": \"$1,923.95\",\n    \"picture\": \"http://placehold.it/32x32\",\n    \"age\": 35,\n    \"eyeColor\": \"brown\",\n    \"name\": \"Wanda Cote\",\n    \"gender\": \"female\",\n    \"company\": \"RONBERT\",\n    \"email\": \"wandacote@ronbert.com\",\n    \"phone\": \"+1 (953) 577-2066\",\n    \"address\": \"352 Louisiana Avenue, Wadsworth, Iowa, 354\",\n    \"about\": \"Qui ad duis consequat Lorem et nisi fugiat non et deserunt pariatur. Ullamco et velit aute magna officia ullamco culpa. Laborum pariatur ex deserunt laborum.\\r\\n\",\n    \"registered\": \"2016-07-05T06:46:18 -01:00\",\n    \"latitude\": 74.488765,\n    \"longitude\": 47.891038,\n    \"tags\": [\n      \"adipisicing\",\n      \"anim\",\n      \"sit\",\n      \"quis\",\n      \"ipsum\",\n      \"aliqua\",\n      \"officia\"\n    ],\n    \"friends\": [\n      {\n        \"id\": 0,\n        \"name\": \"Heath Joseph\"\n      },\n      {\n        \"id\": 1,\n        \"name\": \"Manning Jarvis\"\n      },\n      {\n        \"id\": 2,\n        \"name\": \"Wall Heath\"\n      }\n    ],\n    \"greeting\": \"Hello, Wanda Cote! You have 8 unread messages.\",\n    \"favoriteFruit\": \"apple\"\n  },\n  {\n    \"_id\": \"59b53bcb084c37005beb12b0\",\n    \"index\": 73,\n    \"guid\": \"b7330764-4c34-40a3-9958-195fab4b3d91\",\n    \"isActive\": false,\n    \"balance\": \"$2,499.95\",\n    \"picture\": \"http://placehold.it/32x32\",\n    \"age\": 29,\n    \"eyeColor\": \"blue\",\n    \"name\": \"Herman Parsons\",\n    \"gender\": \"male\",\n    \"company\": \"CANOPOLY\",\n    \"email\": \"hermanparsons@canopoly.com\",\n    \"phone\": \"+1 (858) 469-2039\",\n    \"address\": \"406 Ingraham Street, Freeburn, Wyoming, 9051\",\n    \"about\": \"Officia fugiat voluptate dolore ut ex elit. Proident non sint culpa incididunt ipsum aliquip occaecat dolore. Non enim anim aute consectetur in ex. Pariatur sint labore anim non dolor duis amet nisi cupidatat sit laborum anim veniam eiusmod. Do veniam voluptate eiusmod irure eiusmod ullamco veniam adipisicing laborum est laborum aliquip. Deserunt ex in magna eu aute excepteur ea. Excepteur ipsum aliquip nostrud anim.\\r\\n\",\n    \"registered\": \"2016-03-18T07:09:45 -00:00\",\n    \"latitude\": 45.260943,\n    \"longitude\": 94.785454,\n    \"tags\": [\n      \"nisi\",\n      \"ipsum\",\n      \"esse\",\n      \"culpa\",\n      \"dolore\",\n      \"elit\",\n      \"in\"\n    ],\n    \"friends\": [\n      {\n        \"id\": 0,\n        \"name\": \"Walsh Mcdaniel\"\n      },\n      {\n        \"id\": 1,\n        \"name\": \"Hardin Carter\"\n      },\n      {\n        \"id\": 2,\n        \"name\": \"Stuart Hall\"\n      }\n    ],\n    \"greeting\": \"Hello, Herman Parsons! You have 8 unread messages.\",\n    \"favoriteFruit\": \"banana\"\n  },\n  {\n    \"_id\": \"59b53bcb527263f7fc30c523\",\n    \"index\": 74,\n    \"guid\": \"61ea1af5-38ec-49ca-a918-8c9be1df0919\",\n    \"isActive\": true,\n    \"balance\": \"$2,336.60\",\n    \"picture\": \"http://placehold.it/32x32\",\n    \"age\": 36,\n    \"eyeColor\": \"brown\",\n    \"name\": \"Patterson Benton\",\n    \"gender\": \"male\",\n    \"company\": \"UTARIAN\",\n    \"email\": \"pattersonbenton@utarian.com\",\n    \"phone\": \"+1 (976) 509-3593\",\n    \"address\": \"459 Hampton Place, Leola, Marshall Islands, 109\",\n    \"about\": \"Cupidatat do anim deserunt enim. Sint id consectetur culpa consectetur duis ex occaecat eiusmod eu mollit ipsum minim. Sint incididunt aliqua velit in. Aliquip eiusmod esse ad est aute laborum est sunt ea esse. Quis eu deserunt aute pariatur qui. Proident incididunt nisi id mollit et dolor veniam adipisicing aliqua eu excepteur id sint exercitation.\\r\\n\",\n    \"registered\": \"2016-09-11T07:59:11 -01:00\",\n    \"latitude\": -34.270598,\n    \"longitude\": 173.169207,\n    \"tags\": [\n      \"voluptate\",\n      \"consectetur\",\n      \"voluptate\",\n      \"fugiat\",\n      \"laboris\",\n      \"cillum\",\n      \"occaecat\"\n    ],\n    \"friends\": [\n      {\n        \"id\": 0,\n        \"name\": \"Campbell Swanson\"\n      },\n      {\n        \"id\": 1,\n        \"name\": \"Jenkins Fuller\"\n      },\n      {\n        \"id\": 2,\n        \"name\": \"Boyer Maxwell\"\n      }\n    ],\n    \"greeting\": \"Hello, Patterson Benton! You have 3 unread messages.\",\n    \"favoriteFruit\": \"banana\"\n  },\n  {\n    \"_id\": \"59b53bcb55cf0122e1804227\",\n    \"index\": 75,\n    \"guid\": \"6410aae3-9791-4171-bc46-fe1160c2d3d4\",\n    \"isActive\": false,\n    \"balance\": \"$2,752.83\",\n    \"picture\": \"http://placehold.it/32x32\",\n    \"age\": 31,\n    \"eyeColor\": \"green\",\n    \"name\": \"Gracie Luna\",\n    \"gender\": \"female\",\n    \"company\": \"NEWCUBE\",\n    \"email\": \"gracieluna@newcube.com\",\n    \"phone\": \"+1 (950) 514-3889\",\n    \"address\": \"112 Arlington Place, Alfarata, Nevada, 8390\",\n    \"about\": \"Quis amet amet proident magna aliqua pariatur id cupidatat. Et duis ipsum eiusmod exercitation cillum voluptate voluptate cupidatat veniam elit veniam culpa. Eiusmod excepteur proident est in occaecat. Cillum veniam eiusmod laboris irure qui nostrud sit duis ullamco. Nostrud ullamco sint ad esse laborum consectetur anim aliquip ea veniam voluptate in. Adipisicing tempor ea pariatur ex nisi deserunt nostrud duis. Quis pariatur in deserunt Lorem laborum laborum.\\r\\n\",\n    \"registered\": \"2016-01-24T04:20:49 -00:00\",\n    \"latitude\": 65.338318,\n    \"longitude\": -113.569985,\n    \"tags\": [\n      \"Lorem\",\n      \"proident\",\n      \"pariatur\",\n      \"nisi\",\n      \"ex\",\n      \"sit\",\n      \"minim\"\n    ],\n    \"friends\": [\n      {\n        \"id\": 0,\n        \"name\": \"Marshall Whitaker\"\n      },\n      {\n        \"id\": 1,\n        \"name\": \"Franco Randolph\"\n      },\n      {\n        \"id\": 2,\n        \"name\": \"Rodgers Acevedo\"\n      }\n    ],\n    \"greeting\": \"Hello, Gracie Luna! You have 2 unread messages.\",\n    \"favoriteFruit\": \"banana\"\n  },\n  {\n    \"_id\": \"59b53bcb8af5d0cb60390e81\",\n    \"index\": 76,\n    \"guid\": \"e3634b1c-9b8a-4352-811b-26ea270eb854\",\n    \"isActive\": true,\n    \"balance\": \"$2,462.40\",\n    \"picture\": \"http://placehold.it/32x32\",\n    \"age\": 39,\n    \"eyeColor\": \"blue\",\n    \"name\": \"Landry Townsend\",\n    \"gender\": \"male\",\n    \"company\": \"COMTRACT\",\n    \"email\": \"landrytownsend@comtract.com\",\n    \"phone\": \"+1 (904) 551-3761\",\n    \"address\": \"223 Rockwell Place, Coalmont, North Carolina, 9268\",\n    \"about\": \"Dolore ipsum occaecat quis deserunt excepteur consequat officia sit elit ea deserunt deserunt ut velit. Magna cupidatat dolore velit duis ullamco cupidatat eu fugiat do sint cupidatat dolore. In qui amet occaecat nisi consectetur consectetur ipsum aliquip excepteur nostrud ut quis fugiat dolor. Fugiat eu proident proident fugiat enim anim cupidatat elit sint consectetur irure est eu.\\r\\n\",\n    \"registered\": \"2015-12-01T12:13:22 -00:00\",\n    \"latitude\": 26.684426,\n    \"longitude\": 37.304822,\n    \"tags\": [\n      \"reprehenderit\",\n      \"officia\",\n      \"ad\",\n      \"Lorem\",\n      \"proident\",\n      \"amet\",\n      \"minim\"\n    ],\n    \"friends\": [\n      {\n        \"id\": 0,\n        \"name\": \"Tommie Hayes\"\n      },\n      {\n        \"id\": 1,\n        \"name\": \"Ana Morgan\"\n      },\n      {\n        \"id\": 2,\n        \"name\": \"Snow Sherman\"\n      }\n    ],\n    \"greeting\": \"Hello, Landry Townsend! You have 4 unread messages.\",\n    \"favoriteFruit\": \"banana\"\n  },\n  {\n    \"_id\": \"59b53bcb2c27fefc63f2a7ae\",\n    \"index\": 77,\n    \"guid\": \"88476412-4c1a-4f8f-994a-6d052651dcd4\",\n    \"isActive\": true,\n    \"balance\": \"$1,302.88\",\n    \"picture\": \"http://placehold.it/32x32\",\n    \"age\": 36,\n    \"eyeColor\": \"blue\",\n    \"name\": \"Janelle Patton\",\n    \"gender\": \"female\",\n    \"company\": \"QUAREX\",\n    \"email\": \"janellepatton@quarex.com\",\n    \"phone\": \"+1 (913) 416-3894\",\n    \"address\": \"890 Waldane Court, Clinton, New Mexico, 861\",\n    \"about\": \"Pariatur deserunt Lorem magna aliquip ea esse aliqua irure. Esse eiusmod esse excepteur et sit proident cupidatat adipisicing officia et fugiat. Et esse eiusmod laboris aute est elit. Incididunt consequat et irure cupidatat incididunt qui reprehenderit aliqua in. Labore aliqua qui amet elit. Magna in exercitation incididunt esse fugiat deserunt deserunt Lorem tempor. Et pariatur pariatur incididunt labore ut occaecat laboris pariatur pariatur.\\r\\n\",\n    \"registered\": \"2015-06-17T10:19:36 -01:00\",\n    \"latitude\": -46.295286,\n    \"longitude\": 176.279204,\n    \"tags\": [\n      \"do\",\n      \"reprehenderit\",\n      \"voluptate\",\n      \"ullamco\",\n      \"duis\",\n      \"do\",\n      \"culpa\"\n    ],\n    \"friends\": [\n      {\n        \"id\": 0,\n        \"name\": \"Brandy Dalton\"\n      },\n      {\n        \"id\": 1,\n        \"name\": \"Norris Sparks\"\n      },\n      {\n        \"id\": 2,\n        \"name\": \"Cobb Dyer\"\n      }\n    ],\n    \"greeting\": \"Hello, Janelle Patton! You have 8 unread messages.\",\n    \"favoriteFruit\": \"apple\"\n  },\n  {\n    \"_id\": \"59b53bcbeaa09930d8cb67e3\",\n    \"index\": 78,\n    \"guid\": \"aa15604b-5a80-4a46-ac58-e1f7b908819a\",\n    \"isActive\": false,\n    \"balance\": \"$3,040.74\",\n    \"picture\": \"http://placehold.it/32x32\",\n    \"age\": 30,\n    \"eyeColor\": \"blue\",\n    \"name\": \"Agnes Frye\",\n    \"gender\": \"female\",\n    \"company\": \"SARASONIC\",\n    \"email\": \"agnesfrye@sarasonic.com\",\n    \"phone\": \"+1 (883) 528-2733\",\n    \"address\": \"798 Evans Street, Freelandville, Michigan, 1541\",\n    \"about\": \"Aliqua veniam ullamco nisi amet. Officia in anim minim amet minim cupidatat esse laborum. Quis sint fugiat deserunt incididunt enim sit magna occaecat mollit.\\r\\n\",\n    \"registered\": \"2014-01-11T05:01:09 -00:00\",\n    \"latitude\": -55.686363,\n    \"longitude\": -121.895445,\n    \"tags\": [\n      \"nostrud\",\n      \"adipisicing\",\n      \"proident\",\n      \"reprehenderit\",\n      \"minim\",\n      \"incididunt\",\n      \"do\"\n    ],\n    \"friends\": [\n      {\n        \"id\": 0,\n        \"name\": \"Bowman Haynes\"\n      },\n      {\n        \"id\": 1,\n        \"name\": \"Rosalind Dejesus\"\n      },\n      {\n        \"id\": 2,\n        \"name\": \"Mayra Finch\"\n      }\n    ],\n    \"greeting\": \"Hello, Agnes Frye! You have 4 unread messages.\",\n    \"favoriteFruit\": \"apple\"\n  },\n  {\n    \"_id\": \"59b53bcb9737cc098f392507\",\n    \"index\": 79,\n    \"guid\": \"14e019ee-c0ef-4d9f-a34b-1e266fe4f201\",\n    \"isActive\": true,\n    \"balance\": \"$2,153.21\",\n    \"picture\": \"http://placehold.it/32x32\",\n    \"age\": 36,\n    \"eyeColor\": \"blue\",\n    \"name\": \"Edwards Dennis\",\n    \"gender\": \"male\",\n    \"company\": \"ARCTIQ\",\n    \"email\": \"edwardsdennis@arctiq.com\",\n    \"phone\": \"+1 (883) 475-3655\",\n    \"address\": \"269 Melba Court, Soudan, Oregon, 9327\",\n    \"about\": \"Fugiat exercitation sit est excepteur enim culpa. Adipisicing fugiat labore adipisicing fugiat commodo minim. Dolor amet nisi ea deserunt nisi consequat. Duis aliqua in qui veniam exercitation officia labore amet fugiat. Dolore deserunt ullamco quis esse enim incididunt cupidatat. Dolore in laborum dolor id in mollit esse ut sit laborum deserunt duis consequat. Aliqua consectetur nulla esse ad laborum est amet veniam incididunt est anim cillum ad reprehenderit.\\r\\n\",\n    \"registered\": \"2014-11-20T11:02:11 -00:00\",\n    \"latitude\": 4.916048,\n    \"longitude\": 67.818849,\n    \"tags\": [\n      \"ipsum\",\n      \"ea\",\n      \"nisi\",\n      \"fugiat\",\n      \"qui\",\n      \"occaecat\",\n      \"duis\"\n    ],\n    \"friends\": [\n      {\n        \"id\": 0,\n        \"name\": \"Pearson Obrien\"\n      },\n      {\n        \"id\": 1,\n        \"name\": \"Jaime Castillo\"\n      },\n      {\n        \"id\": 2,\n        \"name\": \"Fowler Branch\"\n      }\n    ],\n    \"greeting\": \"Hello, Edwards Dennis! You have 3 unread messages.\",\n    \"favoriteFruit\": \"apple\"\n  },\n  {\n    \"_id\": \"59b53bcbc88425d302bb5dc9\",\n    \"index\": 80,\n    \"guid\": \"8d66411d-3632-46fa-adba-de988295c355\",\n    \"isActive\": true,\n    \"balance\": \"$1,048.45\",\n    \"picture\": \"http://placehold.it/32x32\",\n    \"age\": 20,\n    \"eyeColor\": \"brown\",\n    \"name\": \"Tonya Harrell\",\n    \"gender\": \"female\",\n    \"company\": \"MIRACLIS\",\n    \"email\": \"tonyaharrell@miraclis.com\",\n    \"phone\": \"+1 (955) 521-2821\",\n    \"address\": \"458 Hart Street, Otranto, Florida, 9320\",\n    \"about\": \"Sit laboris tempor do reprehenderit. Reprehenderit exercitation consectetur aliquip nisi nisi occaecat magna magna pariatur. Reprehenderit eiusmod cillum irure aliqua laboris dolore occaecat anim commodo ad dolore. Laborum fugiat minim pariatur sunt enim qui cupidatat labore ex esse cupidatat id aliquip.\\r\\n\",\n    \"registered\": \"2016-08-02T02:36:17 -01:00\",\n    \"latitude\": 60.952856,\n    \"longitude\": 45.278246,\n    \"tags\": [\n      \"minim\",\n      \"nulla\",\n      \"laboris\",\n      \"exercitation\",\n      \"duis\",\n      \"eiusmod\",\n      \"amet\"\n    ],\n    \"friends\": [\n      {\n        \"id\": 0,\n        \"name\": \"Clara Harding\"\n      },\n      {\n        \"id\": 1,\n        \"name\": \"Corine Lindsey\"\n      },\n      {\n        \"id\": 2,\n        \"name\": \"Mcfarland Martinez\"\n      }\n    ],\n    \"greeting\": \"Hello, Tonya Harrell! You have 2 unread messages.\",\n    \"favoriteFruit\": \"strawberry\"\n  },\n  {\n    \"_id\": \"59b53bcb6dc7404c96b23788\",\n    \"index\": 81,\n    \"guid\": \"d16339bd-0d5a-4fda-9a80-3523f38c2607\",\n    \"isActive\": false,\n    \"balance\": \"$3,172.05\",\n    \"picture\": \"http://placehold.it/32x32\",\n    \"age\": 26,\n    \"eyeColor\": \"blue\",\n    \"name\": \"Robertson Malone\",\n    \"gender\": \"male\",\n    \"company\": \"UNIA\",\n    \"email\": \"robertsonmalone@unia.com\",\n    \"phone\": \"+1 (962) 481-2396\",\n    \"address\": \"590 Newel Street, Joppa, Minnesota, 5936\",\n    \"about\": \"Do duis laboris elit dolor amet exercitation. Irure aliqua veniam consectetur culpa enim in officia voluptate ad. Adipisicing sint do et commodo. Culpa in adipisicing voluptate aliqua Lorem exercitation sunt ullamco pariatur voluptate mollit aliquip. Laboris quis labore minim officia. Dolor Lorem tempor aute minim commodo duis incididunt laboris enim sit sint mollit.\\r\\n\",\n    \"registered\": \"2016-07-26T05:07:36 -01:00\",\n    \"latitude\": 74.88141,\n    \"longitude\": -149.072395,\n    \"tags\": [\n      \"sit\",\n      \"commodo\",\n      \"Lorem\",\n      \"ex\",\n      \"fugiat\",\n      \"fugiat\",\n      \"dolor\"\n    ],\n    \"friends\": [\n      {\n        \"id\": 0,\n        \"name\": \"Winifred Tate\"\n      },\n      {\n        \"id\": 1,\n        \"name\": \"Curtis Reid\"\n      },\n      {\n        \"id\": 2,\n        \"name\": \"Chase Keith\"\n      }\n    ],\n    \"greeting\": \"Hello, Robertson Malone! You have 7 unread messages.\",\n    \"favoriteFruit\": \"apple\"\n  },\n  {\n    \"_id\": \"59b53bcb51c65aa434aa3d1f\",\n    \"index\": 82,\n    \"guid\": \"2774080d-3b85-4a4f-97f3-157e9148c011\",\n    \"isActive\": true,\n    \"balance\": \"$3,693.94\",\n    \"picture\": \"http://placehold.it/32x32\",\n    \"age\": 21,\n    \"eyeColor\": \"blue\",\n    \"name\": \"Mercedes Leonard\",\n    \"gender\": \"female\",\n    \"company\": \"MIRACULA\",\n    \"email\": \"mercedesleonard@miracula.com\",\n    \"phone\": \"+1 (847) 435-3340\",\n    \"address\": \"900 Grafton Street, Mulberry, Hawaii, 4401\",\n    \"about\": \"Consectetur laborum eu occaecat occaecat id minim. Duis do veniam adipisicing voluptate consectetur labore quis elit. Cillum dolore ex fugiat deserunt sint ea magna cillum reprehenderit amet consectetur proident. Culpa ut cillum nulla sit voluptate voluptate veniam qui. Ut anim minim pariatur velit dolor cupidatat ut. Irure Lorem fugiat incididunt ad cillum sit nisi sunt sint dolor elit. Elit non minim laborum ex dolor commodo labore quis irure officia duis labore.\\r\\n\",\n    \"registered\": \"2015-09-07T03:13:08 -01:00\",\n    \"latitude\": -37.746734,\n    \"longitude\": 158.145458,\n    \"tags\": [\n      \"ipsum\",\n      \"dolor\",\n      \"occaecat\",\n      \"aute\",\n      \"dolor\",\n      \"ex\",\n      \"id\"\n    ],\n    \"friends\": [\n      {\n        \"id\": 0,\n        \"name\": \"Jerri Miller\"\n      },\n      {\n        \"id\": 1,\n        \"name\": \"Huff Pitts\"\n      },\n      {\n        \"id\": 2,\n        \"name\": \"Kristine Pittman\"\n      }\n    ],\n    \"greeting\": \"Hello, Mercedes Leonard! You have 7 unread messages.\",\n    \"favoriteFruit\": \"apple\"\n  },\n  {\n    \"_id\": \"59b53bcbb5cb7bde1ba115a7\",\n    \"index\": 83,\n    \"guid\": \"5fa9bb18-fd83-47f9-8f54-1c8eab99fa1f\",\n    \"isActive\": false,\n    \"balance\": \"$2,449.67\",\n    \"picture\": \"http://placehold.it/32x32\",\n    \"age\": 27,\n    \"eyeColor\": \"brown\",\n    \"name\": \"Rebekah Cardenas\",\n    \"gender\": \"female\",\n    \"company\": \"MEDCOM\",\n    \"email\": \"rebekahcardenas@medcom.com\",\n    \"phone\": \"+1 (930) 526-2666\",\n    \"address\": \"585 Conduit Boulevard, Edenburg, Pennsylvania, 5520\",\n    \"about\": \"Sint magna ad consequat cupidatat ut quis duis ut deserunt duis sit consequat. Nisi ea ad ex occaecat adipisicing voluptate quis aliquip nostrud amet quis. Veniam consectetur amet magna adipisicing commodo ea esse elit occaecat labore pariatur. Adipisicing laboris Lorem sit incididunt pariatur eu. Do ipsum laborum excepteur cillum in.\\r\\n\",\n    \"registered\": \"2015-04-23T12:08:15 -01:00\",\n    \"latitude\": -70.810485,\n    \"longitude\": -5.673714,\n    \"tags\": [\n      \"eu\",\n      \"elit\",\n      \"do\",\n      \"laboris\",\n      \"eu\",\n      \"pariatur\",\n      \"sunt\"\n    ],\n    \"friends\": [\n      {\n        \"id\": 0,\n        \"name\": \"Selma Hughes\"\n      },\n      {\n        \"id\": 1,\n        \"name\": \"Laverne Ware\"\n      },\n      {\n        \"id\": 2,\n        \"name\": \"Cortez Reilly\"\n      }\n    ],\n    \"greeting\": \"Hello, Rebekah Cardenas! You have 5 unread messages.\",\n    \"favoriteFruit\": \"strawberry\"\n  },\n  {\n    \"_id\": \"59b53bcbf398f609774512fb\",\n    \"index\": 84,\n    \"guid\": \"9798106c-d85b-4df5-a840-9220e34cb34d\",\n    \"isActive\": true,\n    \"balance\": \"$3,845.69\",\n    \"picture\": \"http://placehold.it/32x32\",\n    \"age\": 28,\n    \"eyeColor\": \"brown\",\n    \"name\": \"Rena Norman\",\n    \"gender\": \"female\",\n    \"company\": \"AQUOAVO\",\n    \"email\": \"renanorman@aquoavo.com\",\n    \"phone\": \"+1 (983) 520-2908\",\n    \"address\": \"635 Cedar Street, Richford, Virginia, 7412\",\n    \"about\": \"Id incididunt in veniam officia nisi veniam dolore laboris duis. Eu dolore labore excepteur tempor exercitation pariatur est commodo elit ullamco quis voluptate. Culpa magna anim ad nisi cupidatat proident dolor sit esse aute reprehenderit deserunt id non. Aliquip consequat nulla aliqua mollit dolore nostrud officia amet pariatur commodo proident. Dolore occaecat ex cupidatat ea exercitation velit amet. Laborum officia non anim ea eiusmod tempor consequat laboris est enim culpa irure enim. Sit dolor dolore dolore nisi magna deserunt sint culpa est excepteur aute.\\r\\n\",\n    \"registered\": \"2015-12-14T03:36:58 -00:00\",\n    \"latitude\": -35.296091,\n    \"longitude\": 130.813918,\n    \"tags\": [\n      \"laboris\",\n      \"nisi\",\n      \"ipsum\",\n      \"qui\",\n      \"reprehenderit\",\n      \"ipsum\",\n      \"incididunt\"\n    ],\n    \"friends\": [\n      {\n        \"id\": 0,\n        \"name\": \"Fry Pace\"\n      },\n      {\n        \"id\": 1,\n        \"name\": \"Levy Norton\"\n      },\n      {\n        \"id\": 2,\n        \"name\": \"Lupe Snider\"\n      }\n    ],\n    \"greeting\": \"Hello, Rena Norman! You have 3 unread messages.\",\n    \"favoriteFruit\": \"banana\"\n  },\n  {\n    \"_id\": \"59b53bcb388b74959570b328\",\n    \"index\": 85,\n    \"guid\": \"ef150b45-285d-447c-8120-8e1ae6b7ddb0\",\n    \"isActive\": false,\n    \"balance\": \"$3,528.91\",\n    \"picture\": \"http://placehold.it/32x32\",\n    \"age\": 33,\n    \"eyeColor\": \"green\",\n    \"name\": \"Russell Hunter\",\n    \"gender\": \"male\",\n    \"company\": \"KONNECT\",\n    \"email\": \"russellhunter@konnect.com\",\n    \"phone\": \"+1 (923) 579-2669\",\n    \"address\": \"991 Agate Court, Westwood, Kansas, 7904\",\n    \"about\": \"Mollit officia duis anim laborum et sunt dolor commodo est fugiat. Cillum ipsum minim irure ea pariatur officia non deserunt aliqua sit Lorem veniam. Cillum amet deserunt occaecat eiusmod magna esse mollit. Eiusmod fugiat et cillum minim ullamco velit sint enim qui exercitation. Magna nostrud deserunt adipisicing nisi ullamco quis culpa aliquip voluptate do.\\r\\n\",\n    \"registered\": \"2014-01-24T12:47:30 -00:00\",\n    \"latitude\": -4.402596,\n    \"longitude\": -44.068437,\n    \"tags\": [\n      \"duis\",\n      \"aliqua\",\n      \"aliquip\",\n      \"ullamco\",\n      \"nulla\",\n      \"anim\",\n      \"eiusmod\"\n    ],\n    \"friends\": [\n      {\n        \"id\": 0,\n        \"name\": \"Jolene Bonner\"\n      },\n      {\n        \"id\": 1,\n        \"name\": \"Head Calhoun\"\n      },\n      {\n        \"id\": 2,\n        \"name\": \"Kate Reyes\"\n      }\n    ],\n    \"greeting\": \"Hello, Russell Hunter! You have 6 unread messages.\",\n    \"favoriteFruit\": \"strawberry\"\n  },\n  {\n    \"_id\": \"59b53bcb2db0467411e874a7\",\n    \"index\": 86,\n    \"guid\": \"c8749167-fdd7-4919-911e-bf0b7c47fa22\",\n    \"isActive\": true,\n    \"balance\": \"$3,021.98\",\n    \"picture\": \"http://placehold.it/32x32\",\n    \"age\": 30,\n    \"eyeColor\": \"green\",\n    \"name\": \"Singleton May\",\n    \"gender\": \"male\",\n    \"company\": \"OBONES\",\n    \"email\": \"singletonmay@obones.com\",\n    \"phone\": \"+1 (809) 470-2340\",\n    \"address\": \"513 Stuyvesant Avenue, Fairlee, Puerto Rico, 6772\",\n    \"about\": \"Ea irure Lorem nulla duis do do et nostrud exercitation. Voluptate exercitation aute consequat eu est. Et cillum labore consectetur amet. Ea pariatur magna et excepteur anim sit pariatur occaecat velit sunt veniam anim.\\r\\n\",\n    \"registered\": \"2016-04-15T10:43:19 -01:00\",\n    \"latitude\": -67.961908,\n    \"longitude\": -28.926166,\n    \"tags\": [\n      \"consequat\",\n      \"pariatur\",\n      \"tempor\",\n      \"et\",\n      \"excepteur\",\n      \"incididunt\",\n      \"tempor\"\n    ],\n    \"friends\": [\n      {\n        \"id\": 0,\n        \"name\": \"Mendoza Estes\"\n      },\n      {\n        \"id\": 1,\n        \"name\": \"Bean Bolton\"\n      },\n      {\n        \"id\": 2,\n        \"name\": \"Holder Villarreal\"\n      }\n    ],\n    \"greeting\": \"Hello, Singleton May! You have 3 unread messages.\",\n    \"favoriteFruit\": \"apple\"\n  },\n  {\n    \"_id\": \"59b53bcbaefe5ada14509d19\",\n    \"index\": 87,\n    \"guid\": \"ead04019-6a40-4420-a798-b8883cd03185\",\n    \"isActive\": true,\n    \"balance\": \"$1,396.19\",\n    \"picture\": \"http://placehold.it/32x32\",\n    \"age\": 39,\n    \"eyeColor\": \"blue\",\n    \"name\": \"Jewell Bradshaw\",\n    \"gender\": \"female\",\n    \"company\": \"JUMPSTACK\",\n    \"email\": \"jewellbradshaw@jumpstack.com\",\n    \"phone\": \"+1 (968) 458-2531\",\n    \"address\": \"782 Winthrop Street, Dotsero, South Carolina, 5062\",\n    \"about\": \"Amet deserunt pariatur in elit exercitation labore. Quis dolore Lorem pariatur irure tempor amet culpa duis enim deserunt exercitation proident. Nostrud magna qui irure dolore est excepteur magna nulla ipsum anim ullamco. Velit occaecat sunt exercitation minim consequat. Eu sunt cillum non amet pariatur mollit sunt amet ad non irure.\\r\\n\",\n    \"registered\": \"2014-09-14T04:22:20 -01:00\",\n    \"latitude\": 29.814291,\n    \"longitude\": 61.37831,\n    \"tags\": [\n      \"sint\",\n      \"elit\",\n      \"ad\",\n      \"ad\",\n      \"cupidatat\",\n      \"cillum\",\n      \"sit\"\n    ],\n    \"friends\": [\n      {\n        \"id\": 0,\n        \"name\": \"Rosales Richmond\"\n      },\n      {\n        \"id\": 1,\n        \"name\": \"Sara Duffy\"\n      },\n      {\n        \"id\": 2,\n        \"name\": \"Freida Pollard\"\n      }\n    ],\n    \"greeting\": \"Hello, Jewell Bradshaw! You have 10 unread messages.\",\n    \"favoriteFruit\": \"strawberry\"\n  },\n  {\n    \"_id\": \"59b53bcb431347b2e14132f2\",\n    \"index\": 88,\n    \"guid\": \"caf8be88-33b4-4c13-8fba-e0e573a30583\",\n    \"isActive\": true,\n    \"balance\": \"$1,502.06\",\n    \"picture\": \"http://placehold.it/32x32\",\n    \"age\": 40,\n    \"eyeColor\": \"blue\",\n    \"name\": \"Langley Bauer\",\n    \"gender\": \"male\",\n    \"company\": \"PORTICA\",\n    \"email\": \"langleybauer@portica.com\",\n    \"phone\": \"+1 (980) 600-2629\",\n    \"address\": \"193 George Street, Navarre, Mississippi, 3789\",\n    \"about\": \"Exercitation irure ad magna sunt consequat non. Do amet tempor consequat adipisicing reprehenderit sunt. Do ipsum aliquip dolore amet ullamco. Eu proident reprehenderit consequat velit. Exercitation minim eiusmod quis incididunt magna magna exercitation consectetur irure.\\r\\n\",\n    \"registered\": \"2015-12-09T03:10:32 -00:00\",\n    \"latitude\": 14.711439,\n    \"longitude\": 101.330203,\n    \"tags\": [\n      \"sunt\",\n      \"laboris\",\n      \"nisi\",\n      \"velit\",\n      \"ipsum\",\n      \"fugiat\",\n      \"amet\"\n    ],\n    \"friends\": [\n      {\n        \"id\": 0,\n        \"name\": \"Noble Odom\"\n      },\n      {\n        \"id\": 1,\n        \"name\": \"Mara Everett\"\n      },\n      {\n        \"id\": 2,\n        \"name\": \"Carole Benson\"\n      }\n    ],\n    \"greeting\": \"Hello, Langley Bauer! You have 1 unread messages.\",\n    \"favoriteFruit\": \"apple\"\n  },\n  {\n    \"_id\": \"59b53bcb9cfbbb3d3b86db36\",\n    \"index\": 89,\n    \"guid\": \"585ace61-13af-493d-9fa6-61d9246efb80\",\n    \"isActive\": true,\n    \"balance\": \"$2,788.64\",\n    \"picture\": \"http://placehold.it/32x32\",\n    \"age\": 39,\n    \"eyeColor\": \"green\",\n    \"name\": \"Walker Sandoval\",\n    \"gender\": \"male\",\n    \"company\": \"EXPOSA\",\n    \"email\": \"walkersandoval@exposa.com\",\n    \"phone\": \"+1 (813) 589-3863\",\n    \"address\": \"597 Dunham Place, Albrightsville, Wisconsin, 6040\",\n    \"about\": \"Cillum ipsum velit ea esse cupidatat aliquip deserunt. Velit labore enim et et dolor esse duis voluptate Lorem ea. Esse Lorem excepteur quis cillum mollit anim voluptate fugiat est culpa. Ullamco Lorem fugiat tempor sunt incididunt aliquip occaecat mollit sit aliqua velit. Ex ullamco consequat minim minim do sint commodo anim fugiat do. Cupidatat id nulla in adipisicing magna consequat deserunt cillum. Ad id occaecat mollit id ullamco.\\r\\n\",\n    \"registered\": \"2016-04-14T12:25:38 -01:00\",\n    \"latitude\": -16.535757,\n    \"longitude\": -28.076556,\n    \"tags\": [\n      \"consectetur\",\n      \"commodo\",\n      \"magna\",\n      \"duis\",\n      \"cillum\",\n      \"id\",\n      \"mollit\"\n    ],\n    \"friends\": [\n      {\n        \"id\": 0,\n        \"name\": \"Tamra Watson\"\n      },\n      {\n        \"id\": 1,\n        \"name\": \"Deidre Gamble\"\n      },\n      {\n        \"id\": 2,\n        \"name\": \"Graham Harris\"\n      }\n    ],\n    \"greeting\": \"Hello, Walker Sandoval! You have 6 unread messages.\",\n    \"favoriteFruit\": \"banana\"\n  },\n  {\n    \"_id\": \"59b53bcb4f8125393e1be565\",\n    \"index\": 90,\n    \"guid\": \"50b5a169-63ec-430b-bd65-956e383c7b25\",\n    \"isActive\": true,\n    \"balance\": \"$2,863.84\",\n    \"picture\": \"http://placehold.it/32x32\",\n    \"age\": 33,\n    \"eyeColor\": \"brown\",\n    \"name\": \"Carlene Humphrey\",\n    \"gender\": \"female\",\n    \"company\": \"WEBIOTIC\",\n    \"email\": \"carlenehumphrey@webiotic.com\",\n    \"phone\": \"+1 (957) 535-2883\",\n    \"address\": \"367 Kensington Street, Carrizo, Indiana, 3136\",\n    \"about\": \"Voluptate pariatur ex pariatur duis non quis ex cillum. Labore occaecat tempor in enim proident aliquip. Consequat ex veniam ullamco aute aute cupidatat dolor dolore ad velit incididunt.\\r\\n\",\n    \"registered\": \"2015-09-17T11:41:14 -01:00\",\n    \"latitude\": -25.860369,\n    \"longitude\": 159.878255,\n    \"tags\": [\n      \"eiusmod\",\n      \"consectetur\",\n      \"consectetur\",\n      \"id\",\n      \"id\",\n      \"eiusmod\",\n      \"ad\"\n    ],\n    \"friends\": [\n      {\n        \"id\": 0,\n        \"name\": \"Baird Reed\"\n      },\n      {\n        \"id\": 1,\n        \"name\": \"Dollie Stephens\"\n      },\n      {\n        \"id\": 2,\n        \"name\": \"Greta Buckley\"\n      }\n    ],\n    \"greeting\": \"Hello, Carlene Humphrey! You have 6 unread messages.\",\n    \"favoriteFruit\": \"banana\"\n  },\n  {\n    \"_id\": \"59b53bcb68c2646e78378cd5\",\n    \"index\": 91,\n    \"guid\": \"ea0a37f9-d18f-4eba-8810-ab098ee81cd3\",\n    \"isActive\": true,\n    \"balance\": \"$1,333.07\",\n    \"picture\": \"http://placehold.it/32x32\",\n    \"age\": 22,\n    \"eyeColor\": \"brown\",\n    \"name\": \"Mattie Mckinney\",\n    \"gender\": \"female\",\n    \"company\": \"PATHWAYS\",\n    \"email\": \"mattiemckinney@pathways.com\",\n    \"phone\": \"+1 (985) 530-3103\",\n    \"address\": \"803 Taaffe Place, Brutus, Tennessee, 1065\",\n    \"about\": \"Aute aute ipsum nostrud commodo. Elit laboris magna irure id laboris eu et nisi. Sit ipsum irure deserunt voluptate nisi ut ut. Aute ullamco deserunt ex elit in et qui excepteur aliquip. Dolore id veniam irure irure anim irure ex exercitation id ea.\\r\\n\",\n    \"registered\": \"2014-11-08T08:00:06 -00:00\",\n    \"latitude\": -3.533773,\n    \"longitude\": -136.23028,\n    \"tags\": [\n      \"sit\",\n      \"excepteur\",\n      \"esse\",\n      \"fugiat\",\n      \"proident\",\n      \"id\",\n      \"veniam\"\n    ],\n    \"friends\": [\n      {\n        \"id\": 0,\n        \"name\": \"Latonya Wright\"\n      },\n      {\n        \"id\": 1,\n        \"name\": \"Mable Estrada\"\n      },\n      {\n        \"id\": 2,\n        \"name\": \"Estelle Henson\"\n      }\n    ],\n    \"greeting\": \"Hello, Mattie Mckinney! You have 2 unread messages.\",\n    \"favoriteFruit\": \"strawberry\"\n  },\n  {\n    \"_id\": \"59b53bcb88186672d782d77f\",\n    \"index\": 92,\n    \"guid\": \"63483e35-f63f-47ea-904f-a48dcde71fb1\",\n    \"isActive\": false,\n    \"balance\": \"$3,958.35\",\n    \"picture\": \"http://placehold.it/32x32\",\n    \"age\": 22,\n    \"eyeColor\": \"green\",\n    \"name\": \"Tamara Russo\",\n    \"gender\": \"female\",\n    \"company\": \"EBIDCO\",\n    \"email\": \"tamararusso@ebidco.com\",\n    \"phone\": \"+1 (941) 482-2355\",\n    \"address\": \"184 Dumont Avenue, Chumuckla, Georgia, 7344\",\n    \"about\": \"Tempor cupidatat labore excepteur irure velit sunt aliqua aliquip ea qui. Deserunt mollit cupidatat non amet exercitation eu proident. Occaecat excepteur aliqua exercitation irure dolor. Eiusmod adipisicing incididunt reprehenderit anim proident nulla cupidatat anim. In non consectetur laborum adipisicing nostrud. Eiusmod mollit voluptate aute et ut est voluptate enim laborum occaecat incididunt.\\r\\n\",\n    \"registered\": \"2014-01-11T06:03:38 -00:00\",\n    \"latitude\": 4.570218,\n    \"longitude\": 97.967557,\n    \"tags\": [\n      \"adipisicing\",\n      \"occaecat\",\n      \"tempor\",\n      \"anim\",\n      \"commodo\",\n      \"do\",\n      \"ea\"\n    ],\n    \"friends\": [\n      {\n        \"id\": 0,\n        \"name\": \"Suzette Burch\"\n      },\n      {\n        \"id\": 1,\n        \"name\": \"Velazquez Mayer\"\n      },\n      {\n        \"id\": 2,\n        \"name\": \"Shannon Powell\"\n      }\n    ],\n    \"greeting\": \"Hello, Tamara Russo! You have 9 unread messages.\",\n    \"favoriteFruit\": \"banana\"\n  },\n  {\n    \"_id\": \"59b53bcb9c166135e4f617f9\",\n    \"index\": 93,\n    \"guid\": \"93bacd52-b79c-429e-8685-45799e149002\",\n    \"isActive\": false,\n    \"balance\": \"$2,892.53\",\n    \"picture\": \"http://placehold.it/32x32\",\n    \"age\": 22,\n    \"eyeColor\": \"brown\",\n    \"name\": \"Camacho Talley\",\n    \"gender\": \"male\",\n    \"company\": \"GRAINSPOT\",\n    \"email\": \"camachotalley@grainspot.com\",\n    \"phone\": \"+1 (877) 502-3157\",\n    \"address\": \"977 Roosevelt Court, Gila, New Hampshire, 5370\",\n    \"about\": \"Duis nulla culpa cupidatat amet amet qui. Ut sit dolor laboris quis ullamco. Aute nulla aliqua voluptate fugiat labore ut. Sunt veniam veniam duis commodo pariatur. Commodo occaecat anim ad est aliquip.\\r\\n\",\n    \"registered\": \"2014-09-29T05:59:11 -01:00\",\n    \"latitude\": 65.471967,\n    \"longitude\": -142.24607,\n    \"tags\": [\n      \"id\",\n      \"aute\",\n      \"magna\",\n      \"eiusmod\",\n      \"mollit\",\n      \"ipsum\",\n      \"commodo\"\n    ],\n    \"friends\": [\n      {\n        \"id\": 0,\n        \"name\": \"Hopkins Atkins\"\n      },\n      {\n        \"id\": 1,\n        \"name\": \"Mcclain Santos\"\n      },\n      {\n        \"id\": 2,\n        \"name\": \"Enid Kemp\"\n      }\n    ],\n    \"greeting\": \"Hello, Camacho Talley! You have 5 unread messages.\",\n    \"favoriteFruit\": \"strawberry\"\n  },\n  {\n    \"_id\": \"59b53bcbe2a5bd209ec5b3c8\",\n    \"index\": 94,\n    \"guid\": \"036605db-b6ec-42e9-a1bc-ee2f3b70a5df\",\n    \"isActive\": false,\n    \"balance\": \"$3,938.69\",\n    \"picture\": \"http://placehold.it/32x32\",\n    \"age\": 38,\n    \"eyeColor\": \"green\",\n    \"name\": \"Barbra Morton\",\n    \"gender\": \"female\",\n    \"company\": \"DANJA\",\n    \"email\": \"barbramorton@danja.com\",\n    \"phone\": \"+1 (948) 444-3914\",\n    \"address\": \"970 Rutherford Place, Selma, Louisiana, 3091\",\n    \"about\": \"Proident labore esse non enim consequat laboris quis irure pariatur enim. Aliquip veniam id occaecat laborum consectetur proident ea cillum amet consequat in id. Esse fugiat veniam ullamco culpa exercitation. Pariatur deserunt consectetur qui consectetur aliquip ea irure eiusmod. Ipsum sint ad ex id. Veniam laborum quis cillum qui quis exercitation qui aliquip mollit eiusmod.\\r\\n\",\n    \"registered\": \"2017-08-11T12:43:09 -01:00\",\n    \"latitude\": 36.516788,\n    \"longitude\": 150.180024,\n    \"tags\": [\n      \"tempor\",\n      \"id\",\n      \"aliquip\",\n      \"sit\",\n      \"dolore\",\n      \"qui\",\n      \"nulla\"\n    ],\n    \"friends\": [\n      {\n        \"id\": 0,\n        \"name\": \"Benton Boyle\"\n      },\n      {\n        \"id\": 1,\n        \"name\": \"Bates Mejia\"\n      },\n      {\n        \"id\": 2,\n        \"name\": \"Montoya Weber\"\n      }\n    ],\n    \"greeting\": \"Hello, Barbra Morton! You have 3 unread messages.\",\n    \"favoriteFruit\": \"strawberry\"\n  },\n  {\n    \"_id\": \"59b53bcb7e036dc098f119d8\",\n    \"index\": 95,\n    \"guid\": \"acd5167b-c778-494e-9b08-c3867c5930d5\",\n    \"isActive\": true,\n    \"balance\": \"$3,887.96\",\n    \"picture\": \"http://placehold.it/32x32\",\n    \"age\": 28,\n    \"eyeColor\": \"blue\",\n    \"name\": \"Andrea Barton\",\n    \"gender\": \"female\",\n    \"company\": \"TRIPSCH\",\n    \"email\": \"andreabarton@tripsch.com\",\n    \"phone\": \"+1 (839) 508-3740\",\n    \"address\": \"531 Elm Place, Choctaw, Oklahoma, 4348\",\n    \"about\": \"Aute ullamco laborum esse quis voluptate enim amet consectetur non incididunt nostrud anim sit ea. Quis eiusmod reprehenderit tempor ea aliquip. Magna laboris pariatur id aliqua nostrud labore incididunt ut.\\r\\n\",\n    \"registered\": \"2017-01-18T09:09:30 -00:00\",\n    \"latitude\": 87.073078,\n    \"longitude\": -153.089878,\n    \"tags\": [\n      \"minim\",\n      \"deserunt\",\n      \"proident\",\n      \"dolore\",\n      \"sunt\",\n      \"excepteur\",\n      \"ea\"\n    ],\n    \"friends\": [\n      {\n        \"id\": 0,\n        \"name\": \"Samantha Carrillo\"\n      },\n      {\n        \"id\": 1,\n        \"name\": \"Burke Mckenzie\"\n      },\n      {\n        \"id\": 2,\n        \"name\": \"Alford Love\"\n      }\n    ],\n    \"greeting\": \"Hello, Andrea Barton! You have 6 unread messages.\",\n    \"favoriteFruit\": \"strawberry\"\n  },\n  {\n    \"_id\": \"59b53bcbe68489b710be92d8\",\n    \"index\": 96,\n    \"guid\": \"fcdbceb5-35bc-464d-9cda-0730a96ae61d\",\n    \"isActive\": false,\n    \"balance\": \"$3,067.07\",\n    \"picture\": \"http://placehold.it/32x32\",\n    \"age\": 29,\n    \"eyeColor\": \"blue\",\n    \"name\": \"Edna Simpson\",\n    \"gender\": \"female\",\n    \"company\": \"TYPHONICA\",\n    \"email\": \"ednasimpson@typhonica.com\",\n    \"phone\": \"+1 (887) 582-2829\",\n    \"address\": \"169 Dictum Court, Callaghan, Alaska, 6930\",\n    \"about\": \"Elit veniam ea culpa do nulla consequat culpa ad sunt enim. Laborum aliqua voluptate incididunt magna aliqua consectetur officia consequat anim fugiat aliquip proident cillum. Sunt proident occaecat dolore aute tempor labore minim consectetur. Esse mollit velit id aute minim eiusmod labore cillum. Adipisicing aliquip minim cupidatat nulla aliquip eiusmod quis ut nulla occaecat nulla cupidatat. Tempor laboris consectetur reprehenderit mollit eu cillum pariatur laboris commodo enim Lorem officia.\\r\\n\",\n    \"registered\": \"2016-05-10T05:37:46 -01:00\",\n    \"latitude\": -30.023422,\n    \"longitude\": 0.886087,\n    \"tags\": [\n      \"in\",\n      \"id\",\n      \"officia\",\n      \"anim\",\n      \"labore\",\n      \"ad\",\n      \"sunt\"\n    ],\n    \"friends\": [\n      {\n        \"id\": 0,\n        \"name\": \"Lina Brown\"\n      },\n      {\n        \"id\": 1,\n        \"name\": \"Cain Campos\"\n      },\n      {\n        \"id\": 2,\n        \"name\": \"Sparks Jones\"\n      }\n    ],\n    \"greeting\": \"Hello, Edna Simpson! You have 10 unread messages.\",\n    \"favoriteFruit\": \"banana\"\n  },\n  {\n    \"_id\": \"59b53bcbcfbbc8d0511541f4\",\n    \"index\": 97,\n    \"guid\": \"7281cfd2-d40d-48e4-957e-b86b371683a2\",\n    \"isActive\": true,\n    \"balance\": \"$2,179.76\",\n    \"picture\": \"http://placehold.it/32x32\",\n    \"age\": 35,\n    \"eyeColor\": \"brown\",\n    \"name\": \"Charlene Woods\",\n    \"gender\": \"female\",\n    \"company\": \"JUNIPOOR\",\n    \"email\": \"charlenewoods@junipoor.com\",\n    \"phone\": \"+1 (919) 557-3560\",\n    \"address\": \"161 Tabor Court, Itmann, North Dakota, 9686\",\n    \"about\": \"Mollit velit cillum irure Lorem id consectetur fugiat. Reprehenderit ipsum aliquip tempor dolor. Eu reprehenderit tempor adipisicing anim duis non quis officia excepteur fugiat sunt adipisicing. Consectetur qui aliquip eiusmod laborum do incididunt id ipsum sint est elit ad commodo. Adipisicing veniam eu tempor id et nisi fugiat. Qui duis aute fugiat qui ut id ut deserunt adipisicing aliqua. Fugiat aliqua incididunt Lorem esse ipsum elit magna quis eiusmod pariatur.\\r\\n\",\n    \"registered\": \"2014-09-19T12:55:15 -01:00\",\n    \"latitude\": 23.852484,\n    \"longitude\": 64.974725,\n    \"tags\": [\n      \"deserunt\",\n      \"pariatur\",\n      \"nulla\",\n      \"qui\",\n      \"nulla\",\n      \"proident\",\n      \"aliquip\"\n    ],\n    \"friends\": [\n      {\n        \"id\": 0,\n        \"name\": \"Rachael Cabrera\"\n      },\n      {\n        \"id\": 1,\n        \"name\": \"Best Huber\"\n      },\n      {\n        \"id\": 2,\n        \"name\": \"Luann Abbott\"\n      }\n    ],\n    \"greeting\": \"Hello, Charlene Woods! You have 2 unread messages.\",\n    \"favoriteFruit\": \"banana\"\n  },\n  {\n    \"_id\": \"59b53bcb678a7787e8012db4\",\n    \"index\": 98,\n    \"guid\": \"7519df16-5d86-4a4e-a0b6-19e2f100d49d\",\n    \"isActive\": true,\n    \"balance\": \"$3,153.52\",\n    \"picture\": \"http://placehold.it/32x32\",\n    \"age\": 31,\n    \"eyeColor\": \"blue\",\n    \"name\": \"Pugh Christensen\",\n    \"gender\": \"male\",\n    \"company\": \"PLEXIA\",\n    \"email\": \"pughchristensen@plexia.com\",\n    \"phone\": \"+1 (803) 541-2906\",\n    \"address\": \"514 Wyckoff Avenue, Concho, Washington, 1004\",\n    \"about\": \"Fugiat duis nisi esse duis ut tempor laborum amet. Ut et labore quis pariatur ullamco deserunt esse occaecat est pariatur. Ut cillum pariatur nulla dolor eu consequat nisi nisi occaecat occaecat ad veniam commodo. Cillum anim eu fugiat minim excepteur dolor sit. Dolore aute ipsum qui magna cillum ipsum enim aute ex. Sint veniam deserunt id do velit eu.\\r\\n\",\n    \"registered\": \"2016-10-15T11:07:09 -01:00\",\n    \"latitude\": -71.61758,\n    \"longitude\": -73.196318,\n    \"tags\": [\n      \"pariatur\",\n      \"officia\",\n      \"do\",\n      \"est\",\n      \"aute\",\n      \"ipsum\",\n      \"elit\"\n    ],\n    \"friends\": [\n      {\n        \"id\": 0,\n        \"name\": \"Todd Mccray\"\n      },\n      {\n        \"id\": 1,\n        \"name\": \"Carrillo Johns\"\n      },\n      {\n        \"id\": 2,\n        \"name\": \"Claire Evans\"\n      }\n    ],\n    \"greeting\": \"Hello, Pugh Christensen! You have 6 unread messages.\",\n    \"favoriteFruit\": \"strawberry\"\n  },\n  {\n    \"_id\": \"59b53bcb07c3d92599f358a7\",\n    \"index\": 99,\n    \"guid\": \"00eb41e9-cb16-49c9-84da-e139407a70e3\",\n    \"isActive\": true,\n    \"balance\": \"$3,233.68\",\n    \"picture\": \"http://placehold.it/32x32\",\n    \"age\": 37,\n    \"eyeColor\": \"blue\",\n    \"name\": \"Knapp Mccullough\",\n    \"gender\": \"male\",\n    \"company\": \"EARWAX\",\n    \"email\": \"knappmccullough@earwax.com\",\n    \"phone\": \"+1 (987) 583-3507\",\n    \"address\": \"180 Adelphi Street, Grahamtown, New York, 2149\",\n    \"about\": \"Aliquip aliquip enim ullamco minim consectetur consequat qui anim nulla do elit dolor dolore. Mollit mollit cillum aliquip culpa veniam esse dolor commodo aliqua laborum dolor duis culpa. Commodo ex id excepteur ipsum. Aliqua occaecat sunt ipsum aliqua exercitation irure. Nisi commodo eu consequat sit elit occaecat excepteur. Fugiat in ipsum excepteur magna minim eiusmod in eu consectetur minim qui exercitation. Laborum irure est ullamco aliqua consectetur aliqua.\\r\\n\",\n    \"registered\": \"2015-12-19T05:55:46 -00:00\",\n    \"latitude\": 46.042325,\n    \"longitude\": 3.527828,\n    \"tags\": [\n      \"occaecat\",\n      \"exercitation\",\n      \"enim\",\n      \"aliqua\",\n      \"ut\",\n      \"eu\",\n      \"amet\"\n    ],\n    \"friends\": [\n      {\n        \"id\": 0,\n        \"name\": \"Maryanne Finley\"\n      },\n      {\n        \"id\": 1,\n        \"name\": \"Goff Joyce\"\n      },\n      {\n        \"id\": 2,\n        \"name\": \"Scott Callahan\"\n      }\n    ],\n    \"greeting\": \"Hello, Knapp Mccullough! You have 4 unread messages.\",\n    \"favoriteFruit\": \"banana\"\n  }\n]"
  # "Example JSON from https://www.json-generator.com"
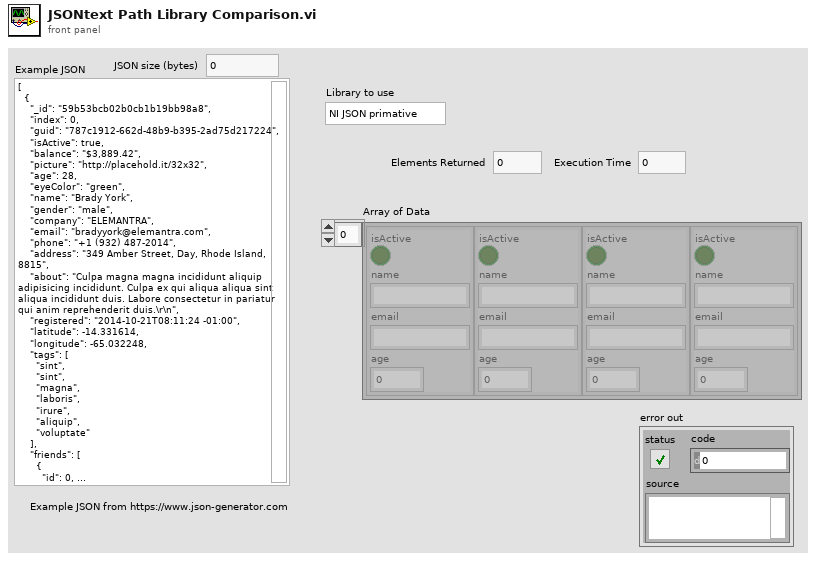
[diagram p1: front panel]
types:
  T1 = enum16{"NI JSON primative", "JSONtext", "LAVA-JSON", "JKI-JSON"}
  T2 = cluster{"isActive":bool, "name":string, "email":string, "age":i32}[]
  T3 = cluster{"isActive":bool, "name":string, "email":string, "age":i32}
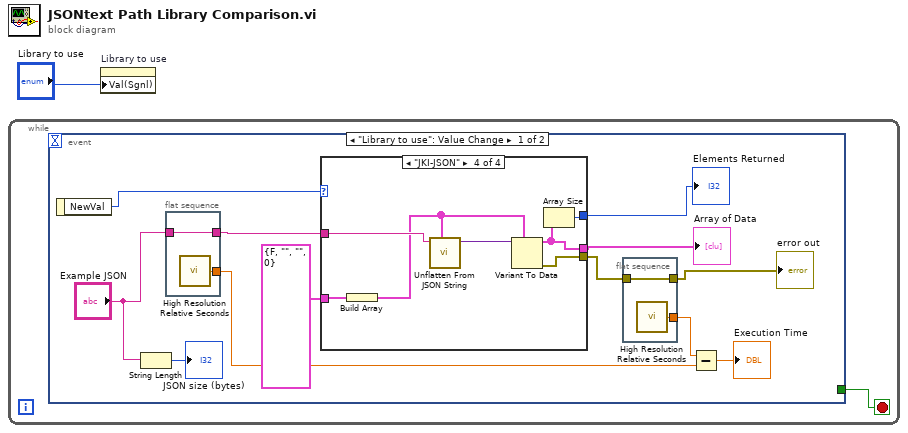
[diagram p0: block diagram]
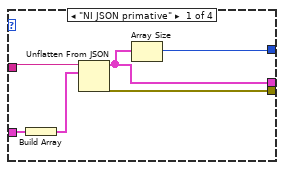
[diagram p2: hidden frame]
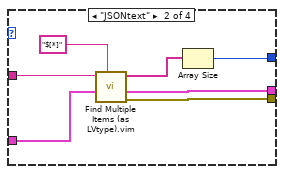
[diagram p3: hidden frame]
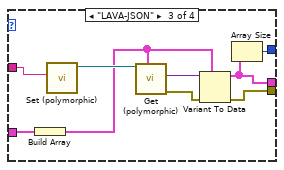
[diagram p4: hidden frame]
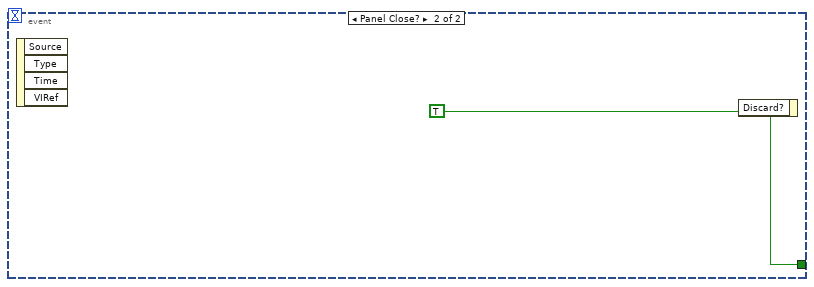
[diagram p5: hidden frame]
diagram:
  n1 = while {
    stop <- w2 stop-if-true
    n2 = event shown="[0] \"Library to use\": Value Change" {
      selector: _ -> [_ _]
      dyn-events: _ -> [_ _]
      timeout: _ -> [_ _]
      tunnel: [_ w48] -> w2
      event "Library to use": Value Change {
        n3 = event-data() -> ("NewVal"=w4:T1)  [unwired: 1 in]
        n4 = String Length(string="Example JSON") -> (length=→"JSON size (bytes)":i32)
        n5 = flat-sequence {
          tunnel: "Example JSON" -> [w47]
          tunnel: [w47] -> w8
          tunnel: [w46] -> w12
          frame #0 {
            n6 = call <vilib>:"High Resolution Relative Seconds.vi"() -> ("relative seconds"=w46:dbl)
          }
        }
        n7 = case shown="\"JKI-JSON\"" w4 {
          tunnel: w8 -> [w20 w27 w36 w38]
          tunnel: [w15 w26 w31 w42] -> w7
          tunnel: T3 {"isActive"=FALSE, "name"="", "email"="", "age"=0} -> [w19 w24 w34 w43]
          tunnel: [w17 w23 w28 w40] -> w3
          tunnel: [w16 w21 w29 w41] -> w5
          frame "NI JSON primative" {
            n8 = Build Array(w19) -> (w18:T2)
            n9 = Unflatten From JSON(JSON string=w20, type and defaults=w18) -> (value=w17:T2, error out=w15:errorcluster)  [unwired: 5 in]
            n10 = Array Size(array=w17) -> (size(s)=w16:i32)
          }
          frame "JSONtext" {
            n11 = call "Find Multiple Items (as LVtype).vim"("Item Path"="$[*]", "Data type of each item"=w24, "JSON"=w27) -> ("error out"=w26:errorcluster, "Array of Data"=w23:T2, "Names"=w22:string[])  [unwired: 5 in, 1 out]
            n12 = Array Size(array=w22) -> (size(s)=w21:i32)
          }
          frame "LAVA-JSON" {
            n13 = Build Array(w34) -> (w30:T2)
            n14 = call-poly <vilib>:"Set (polymorphic).vi"("JSON stream"=w36) -> ("JSON Value out"=w35:refnum<class "JSON Value.lvclass">)  [unwired: 8 in, 2 out]
            n15 = call-poly <vilib>:"Get (polymorphic).vi"("Variant (Data Type)"=w30, "JSON in"=w35) -> ("error out"=w32:errorcluster, "Variant out"=w33:variant)  [unwired: 7 in, 1 out]
            n16 = Variant To Data(error in=w32, type=w30, Variant=w33) -> (data=w28:T2, error out=w31:errorcluster)
            n17 = Array Size(array=w28) -> (size(s)=w29:i32)
          }
          frame "JKI-JSON" {
            n18 = Build Array(w43) -> (w37:T2)
            n19 = call <vilib>:"Unflatten From JSON String.vi"("Type and Defaults"=w37, "JSON String"=w38) -> ("Variant"=w39:variant)  [unwired: 8 in, 1 out]
            n20 = Variant To Data(type=w37, Variant=w39) -> (data=w40:T2, error out=w42:errorcluster)  [unwired: 1 in]
            n21 = Array Size(array=w40) -> (size(s)=w41:i32)
          }
        }
        "Elements Returned" <- w5
        "Array of Data" <- w3
        n22 = flat-sequence {
          tunnel: w7 -> [w45]
          tunnel: [w45] -> w14
          tunnel: [w44] -> w13
          frame #0 {
            n23 = call <vilib>:"High Resolution Relative Seconds.vi"() -> ("relative seconds"=w44:dbl)
          }
        }
        n24 = Subtract(x=w13, y=w12) -> (x-y=→"Execution Time":dbl)
        "error out" <- w14
      }
      event Panel Close? {
        w48 = TRUE
        n25 = event-data() -> ()  [unwired: 1 in, 4 out]
        n26 = event-data("Discard?"=w48) -> ()  [unwired: 1 in, 1 out]
      }
    }
  }
  n27 = property on="Library to use" class="Enum (strict)"("Val(Sgnl)"="Library to use") -> ()  [unwired: 2 in, 2 out]
